vi "HEWH Stand Overide.vi"() -> ()   [LabVIEW 2016]
uses:
  Type Definitions/HEWH Channel Settings.ctl
  Type Definitions/HEWH Tank Indicator.ctl
  Custom Instrument Control/Intellifaucet/Type Definitions/INTELLIFAUCET Set Mode.ctl
  Type Definitions/HEWH Output Information.ctl
  Type Definitions/HEWH GEA2 Cluster.ctl
  Utility/LabVIEW GEA2 Toolkit v1.0.0.0/type defs/Data In.ctl
  Utility/LabVIEW GEA2 Toolkit v1.0.0.0/library/GEA2_Toolkit.lvlib
  Type Definitions/HEWH User Controls.ctl
  Type Definitions/HEWH Power Elements.ctl
  Utility/GEA2 Commands/HEWH/Type Definitions/GEA2 Commands WaterHeater GEA2 Data.ctl
  Type Definitions/HEWH Power Data.ctl
  Utility/Custom Pallet Controls/Custom Pallet String.ctl
  Utility/Custom Pallet Controls/Custom Pallet Quit.ctl
  Utility/Custom Pallet Controls/Custom Pallet DBL.ctl
  Custom Instrument Control/Intellifaucet/Type Definitions/INTELLIFAUCET Tested Flowrate Scenarios.ctl
  Type Definitions/HEWH Draw Pattern Setup.ctl
  Utility/Custom Pallet Controls/Custom Pallet Number.ctl
  Utility/Custom Pallet Controls/Custom Pallet Timer.ctl
  <vilib>/Analysis/NI_AALBase.lvlib
  Type Definitions/HEWH Valve Bank Positions.ctl
  Utility/GEA2 Commands/HEWH/Type Definitions/GEA2 Commands Service Error Codes.ctl
  Utility/GEA2 Commands/HEWH/Type Definitions/GEA2 Commands Status Query.ctl
  Utility/GEA2 Commands/HEWH/Type Definitions/GEA2 Commands Button Status.ctl
  Type Definitions/HEWH Termination Condition Cluster.ctl
  Drivers/Yokogawa WT300 Series/Yokogawa WT300 Series.lvlib
  Drivers/Yokogawa WT200 Series/Yokogawa WT200 Series.lvlib
  <vilib>/Utility/file.llb/Write To Spreadsheet File (DBL).vi
  Utility/Type Definitions/UTILITY Power Analyzer.ctl
  Utility/GEA2 Commands/HEWH/Type Definitions/GEA2 Commands HEWH Mode.ctl
  Utility/GEA2 Commands/HEWH/Type Definitions/GEA2 Commands.ctl
  C:/Technology Lab/NI-2010/Trunk/Utility/LabVIEW GEA2 Toolkit v1.0.0.0/Appliance.NET/GeaCommunication.dll
  Utility/LabVIEW GEA2 Toolkit v1.0.0.0/Appliance.NET/GeaCommunication.dll
  Utility/Type Definitions/UTILITY Notifier.ctl
  <vilib>/Utility/file.llb/Read From Spreadsheet File (string).vi
  Utility/Save File/File Setup.lvlib
  Utility/Save File/File Setup (Public)/Type Definition/Save File DOE Configuration State.ctl
  Utility/Save File/File Setup (Public)/Type Definition/Save File DOE LabView Program.ctl
  Custom Instrument Control/MW100/Type Definitions/Station ID Selector.ctl
  Utility/Save File/File Setup (Public)/Type Definition/Save File HEWH Heating Control Mode.ctl
  Type Definitions/PRAT Test.ctl
  Custom Instrument Control/MW100/Type Definitions/HEWH Solenoid Valve Status.ctl
  Type Definitions/HEWH Calc and Calibration.ctl
  Type Definitions/HEWH Start Conditions.ctl
  Support VIs/Draw Water Specific/Type Definitions/Terminate Draw Conditions.ctl
  Type Definitions/HEWH Draw Flag ENUM.ctl
  Support VIs/Draw Water Specific/Type Definitions/HEWH Special Condition Check.ctl
  Support VIs/Draw Water Specific/Type Definitions/Check Special Condtions.ctl
  <vilib>/Utility/file.llb/Write To Spreadsheet File (string).vi
  Type Definitions/HEWH Equipment References.ctl
  Utility/Custom Pallet Controls/Custom Pallet Chart.ctl
  Utility/Custom Pallet Controls/Custom Pallet Reverse.ctl
  Utility/Custom Pallet Controls/Custom Pallet Configuration.ctl
  Type Definitions/HEWH Program Names.ctl
  Type Definitions/HEWH PreDraw.ctl
  Utility/Save File/File Setup (Public)/Type Definition/Save File DOE Data Save Filepaths.ctl
  Utility/Save File/File Setup (Public)/Type Definition/Save File DOE File Path Control.ctl
  Utility/Type Definitions/UTILITY Power Inputs Control.ctl
  Drivers/IND560 Scale Monitor/Type Definitions/IND560 Configuration.ctl
  Type Definitions/HEWH Agilent Cluster.ctl
  Utility/Type Definitions/UTILITY TC Coefficients.ctl
  Washer DOE/Type Definitions/DOE Test Fixture Hardware.ctl
  Washer DOE/Configuration/GEA2.ctl
  Washer DOE/Type Definitions/DOE Capacity Measurments.ctl
  <vilib>/Platform/fileVersionInfo.llb/FileVersionInformation.ctl
  Utility/Save File/File Setup (Public)/Type Definition/Save File DISH Dishwasher Details.ctl
  Drivers/Omega FMA-1600A Series Gas Flow Meter/Type Definitions/FMA1600A COM Ports.ctl
  Washer DOE/Type Definitions/DOE Appliance Common.ctl
  Washer DOE/Type Definitions/DOE Dryer Standard.ctl
  Utility/Save File/File Setup (Public)/Type Definition/DPT IMC Data.ctl
panel:
  out "Error Out 2":errorcluster
  in  "24HR Error In":errorcluster
  in  "Skip Draw":bool
  in  "Skip Purge":bool
  out "DAQ Loop Complete":bool
  out "Core HEWH Data DAQ LOOP":T1={"Scan Rate Adjust"=0.0, "Draw Count"=0, "Test Patten Setup"={"Dispense Times"=[], "Total Gallons Schedule"=[], "Flow Rate Schedule "=[], "Incoming Water Temperature"=[], "PreDraw Pattern"=[], "24 Hour PreDraw"=enum."Zero Pre-Draws", "Pre-Draw Until?"=[], "Purge Until Cutout"=FALSE, "Heating Flag"=FALSE, "PRAT/RLT Sequence"=[]}, "Condition Cluster Output"={"Condition #1"=FALSE, "Condition #2"=FALSE, "Special Last Draw (HU Test)"=FALSE, "RTD Out Temperature <="=0.0, "Condition #3"=FALSE, "Mean Tank Temperature <="=0.0, "Condition #4"=FALSE, "Decrease Outlet Temperature \nBy (RTD Out)"=0.0, "Condition #5"=FALSE, "Condition #6"=FALSE, "Time (Seconds)"=0.0, "Condition #7"=FALSE, "Condition #8"=FALSE, "Draw Until Condition"={"UE"=FALSE, "LE"=FALSE, "COMP"=FALSE, "FANS"=FALSE}, "Condition #9"=FALSE}, "HEWH Specific DAQ"={"HEWH Data"={"HEWH Standard"={"Voltage (Volts)"=0.0, "Current (Amps)"=0.0, "Power (Watts)"=0.0, "WattHours (Wh)"=0.0, "TC Tree (AVG)"=0.0, "Flow Rate (GPM)"=0.0, "Gallons (Gal)"=0.0, "RTD Out (Deg F)"=0.0, "RTD In (Deg F)"=0.0, "RTD Amb (Deg F)"=0.0, "TC Down"=0.0, "UE Event Lead"=0, "LE Event Lead"=0, "TC Tree Array"=[]}, "PRAT"={"Power (Watts) A"=0.0, "Power (Watts) B"=0.0, "Power (Watts) C"=0.0, "Power (Watts) D"=0.0, "TC1"=0.0, "TC2"=0.0, "TC3"=0.0, "TC4"=0.0, "WattHours (Wh) A"=0.0, "WattHours (Wh) B"=0.0, "WattHours (Wh) C"=0.0, "WattHours (Wh) D"=0.0, "Ambient"=0.0, "Extra Temp"=0.0}, "Additional Power Data"={"Vthd"=0.0, "Frequency (Hz)"=0.0, "Apparent Power (VA)"=0.0, "Power Factor"=0.0, "Current Crest Factor"=0.0, "Voltage Crest Factor"=0.0, "Integration Time (sec)"=0.0}}, "Intellif Valve % Open"=0.0, "Power State"={"UE"=FALSE, "LE"=FALSE, "COMP"=FALSE, "FANS"=FALSE}, "Power Analyzer"=enum."", "Intellifaucet Configuration"=enum."DRK500,Station1"}, "Test Output Data"={"PreDraw Data Table"=[], "Data Table"=[], "MW100 TC Headers"=[]}, "Calc and Calibration"={"Mean SD Var Max Min Array"=[], "Draw Statistics (DBL)"=[], "Calibration Coefficients DBL"=[], "Start Gallons"=0.0, "Starting Temp Decline"=0.0, "K-Factor (Intellifaucet)"=0.0, "All Draw Stats"=[], "RTD Terminate Value"=0.0}, "Current Draw Time"=0.0, "LV Program"=enum."HEWH", "Station ID"=enum."A"} {"Test Patten Setup"."PRAT/RLT Sequence"."Time" format="%<%H:%M:%S>t"; "Test Patten Setup"."Incoming Water Temperature" format="%.2f"; "Test Patten Setup"."Flow Rate Schedule" format="%.2f"; "Test Patten Setup"."Total Gallons Schedule" format="%.2f"; "Test Patten Setup"."Dispense Times" format="%<%H:%M:%S>t"}
  out "Description 4":string
  out "Description":string="HEWH Stand Override"
  out "Station":string
  out "TC Tree Average":T19 format="%.2f"
  out "Elapsed Time Output":T20 format="%<%H:%M:%S>t"
  out "Continuous Data Collection Output":bool
  out "Cutout Draw":bool
  in  "Scan Rate (Seconds)":T19=3.0 format="%#.0f"
  in  "Tab Control 2":T21(tab)
  out "Data Table":string[][](array[string])
  in  "Inlet Valve A":enum8{"OPEN", "CLOSE"}(ring)=enum."CLOSE"
  in  "Drain Valve A":enum8{"OPEN", "CLOSE"}(ring)=enum."CLOSE"
  in  "Outlet Valve A":enum8{"CLOSE", "OPEN"}(ring)=enum."OPEN"
  in  "Stop Custom Draw":bool
  in  "Draw Until?":bool
  out "Multi-Draw":bool
  out "Remaining Draws":T22
  in  "Temperature":T19=58.0 format="%.2f"
  in  "Start Multi-Draw":bool
  in  "Draw Schedule":bool
  in  "GPM Target":T19=3.0 format="%.2f"
  in  "Gallon Target":T19=10.72 format="%.2f"
  out "Description 3":string="Custom Draw"
  out "Draw Time":T20 format="%<%H:%M:%S>t"
  in  "Dispense":bool
  out "Start Draw Routine":bool
  out "Start Draw Timer":bool
  out "Draw Count":T22
  out "Trigger With GEA2":bool
  in  "Super Water Heater":bool
  out "Sofware Version":T23
  in  "Software Version":bool
  in  "Setpoint":bool
  in  "Mode":T24
  in  "HEWH Setpoint":T22=135
  out "Start DAQ Write":bool
  out "Program Names Update":T25
  out "Flow Rate (GPM)":T19 format="%.2f"
  out "Tank Display":T26 {"TC6" format="%.2g"; "TIN" format="%.2g"; "TOUT" format="%.2g"; "TC5" format="%.2g"; "TC4" format="%.2g"; "TC3" format="%.2g"; "TC2" format="%.2g"; "TC1" format="%.2g"}
  out "Gallons":T19 format="%.2f"
  out "Voltage (Volts)":T19=240.0 format="%.3f"
  out "Current":T19=240.0 format="%.3f"
  out "Power (Watts)":T19=240.0 format="%.3f"
  out "Watt Hours (Wh)":T19=240.0 format="%.3f"
  out "Custom Draw\nDispensed Gallons (Gal)":T19 format="%.2f"
  out "POWER":T12
  in  "Shutdown Sequence":string
  in  "Settings":T27
  out "Intellifaucet Type":string
  out "Message":T23
  out "Shutdown DAQ":string="Stop Flow\nMacro: Exit"
  out "POWER DAQ LOOP":T12
  out "Out VLV UI":enum8{"CLOSE", "OPEN"}(ring)
  out "Drain VLV UI":enum8{"OPEN", "CLOSE"}(ring)
  out "In Valve UI":enum8{"OPEN", "CLOSE"}(ring)
  out "User Controls DAQ LOOP":T28={"Main Power Control"=FALSE, "Flow Totalizer Control"=TRUE, "Intellifaucet Temperature"=58.0, "Percent Flow"=100.0, "Safe Mode"=TRUE, "GEA2?"=FALSE, "Use Agilent?"=FALSE, "Valve Set A"=enum."Heating", "Valve Set B"=enum."Heating", "Valve Set C"=enum."Heating", "Valve Set D"=enum."Heating", "Valves"={"In VLV A"=enum."OPEN", "Drain VLV A"=enum."CLOSE", "Out VLV A"=enum."CLOSE", "In VLV B"=enum."CLOSE", "Drain VLV B"=enum."CLOSE", "Out VLV B"=enum."CLOSE", "In VLV C"=enum."OPEN", "Drain VLV C"=enum."CLOSE", "Out VLV C"=enum."CLOSE", "In VLV D"=enum."OPEN", "Drain VLV D"=enum."CLOSE", "Out VLV D"=enum."CLOSE"}} {"Percent Flow" scale=40.0..120.0; "Intellifaucet Temperature" scale=40.0..120.0}
  out "Shutdown":string="Stop Flow\nMacro: Exit"
  out "Elapsed Time":T20 format="%<%H:%M:%S>t"
  in  "Main":T30
  in  "Quit":T31
  in  "Tab Control 3":T32(tab)
  in  "Heat Up Panel":bool
  in  "First Hour Rating Panel":bool
  in  "24 Hour Rating Panel":bool
  in  "Stand Override Panel":bool
  in  "Program Names":T25
  in  "Tab Control 5":enum32{"Control", "Analysis"}(tab)
  in  "Flow Totalizer Control":bool
  in  "Reset Totalizer":bool
  in  "Pressurize Tank?":bool=TRUE
  out "Description 2":string="Intellifaucet Control"
  in  "IF Stop":bool
  in  "IF Start":bool
  in  "Valve % Open":dbl(slide)=100.0 scale=0.0..100.0
  in  "Temperature":dbl(slide)=58.0 scale=40.0..120.0
  in  "HEWH Power":bool
  in  "Write To File":bool
  out "Flow Meter 2":T33
  in  "Y-Axis":string(combo)
  in  "X-Axis":string(combo)
  out "XY Graph":cluster{dbl[], dbl[]}(graph)
  in  "Start 24 Hour Rating":bool
  out "24 Hr Test Complete":bool
  in  "Start First Hour Rating":bool
  in  "Start Heat Up Test":bool
  out "Save File Path":path
  in  "Tab Control 4":T34(tab)
  in  "Purge Time (Seconds)":T19=180.0 format="%.2f"
  in  "Last Draw TC Tree AVG Decline Amount (Degrees F)":T19=0.2 format="%.2f"
  in  "Decrease Outlet\nTemperature By (RTD Out)":T19=15.0 format="%.2f"
  out "RTD Max Min Array":dbl[][](array[numeric])
  in  "First Hour GPM Target":T19=3.0 format="%.2f"
  in  "First Hour Temperature":T19=58.0 format="%.2f"
  in  "Total Test Timer (1hr)":T19=3600.0 format="%.2f"
  in  "T2 Degree Diff for Purge":T19=8.0 format="%.2f"
  in  "Heat Up Temperature":T19=58.0 format="%.2f"
  in  "Heat Up GPM Target":T19=3.0 format="%.2f"
  in  "Step 1 Wait Time":T20=1800.0 format="%<%H:%M:%S>t"
  in  "Step 1A Gallon Target":T19=10.72 format="%.2f"
  in  "Step 2 Gallon Target":T19=10.72 format="%.2f"
  in  "Data File Directory":path=path "c:/data"
  in  "Tab Control":T35(tab)
  out "Write To File Change":bool
  out "Heat Up Step 4 Flag":bool
  out "Start UI Loop":bool
  out "Use Agilent?":bool
  out "Loop Time":dbl
  out "Newfi Time":dbl format="%.2f"
  out "Power Display Time":dbl format="%.2f"
  out "Start Time":dbl format="%.2f"
  in  "Scan Rate Adjust":T19=1000.0 format="%.2f"
  out "MW100 Data":string[][](array[string])
  in  "Standard Command":u8(ring)=13 items=["RQST_SOFTWARE_VERSION", "RQST_T2_RESISTANCE", "RQST_T3A_RESISTANCE", "RQST_T3B_RESISTANCE", "RQST_T4_RESISTANCE", "RQST_T5_RESISTANCE", "RQST_IDLB_RESISTANCE", "RQST_MODE_SELECT_RESISTANCE", "RQST_DATA_FROM_MEMORY", "RQST_DATA_FROM_DATA_FLASH", "RQST_SS_FAULT_COUNTS", "RQST_OTHER_FAULT_COUNTS", "CMD_CLEAR_FAULT_COUNTS", "RQST_HYPERTERM_OUTPUT_DATA", "CMD_RESET_FILTER_TIMES", "CMD_WRITE_SETPOINTS", "CMD_TURN_ON_OFF_DLB", "CMD_ENTER_EXIT_FCT_MODE", "CMD_SET_LEDS", "CMD_SET_EEV_DRIVE_LINES", "REQ_READ_KEY_STATUS", "RQST_READ_PERSONALITY", "CMD_ENTER_FACT_MODE", "CMD_RESET", "CMD_RESTORE_EEPROM_DEFAULTS", "CMD_SET_MODEL_NUMBER", "CMD_SET_SERIAL_NUMBER", "RQST_MODEL_NUMBER", "RQST_SERIAL_NUMBER", "CMD_TOGGLE_SERVICE_MODE", "CMD_TOGGLE_UE_SERV", "CMD_TOGGLE_LE_SERV", "CMD_REFRESH_SERVICE_TIMEOUTS", "RQST_DSM_OVERRIDE_STATUS", "RQST_STATUS_QUERY", "RQST_HEM_KWH_DATA", "RQST_SERVICE_ERROR_CODES", "RQST_OVERRIDE_STATUS", "CMD_UPDATE_DSM_LEVEL", "CMD_OVERRIDE_STATUS_CHANGED", "CMD_CLEAR_OVERRIDE_STATUS", "CMD_CLEAR_ENERGY_USAGE_CTRS", "CMD_DSM_OVERRIDES", "CMD_UPDATE_MODE", "CMD_SET_PID_P_DENOMINATOR", "CMD_SET_PID_I_DENOM_UNDER_THR", "CMD_SET_PID_I_DENOM_OVER_THR", "CMD_SET_START_POS_UNDER_THR", "CMD_SET_START_POS_OVER_THR", "CMD_SET_EEV_STOP_POSITION", "CMD_SET_AMBIENT_THRESH_1", "CMD_SET_AMBIENT_THRESH_2", "CMD_SET_AMBIENT_THRESH_3", "CMD_SET_PID_LOW_SH_TARGET", "CMD_SET_PID_MID_SH_TARGET", "RQST_PID_PARAMETERS", "CMD_COMP_OFF", "CMD_TOGGLE_FAN", "CMD_RQST_LED_STATUS", "CMD_UE_2_SECONDS", "CMD_LE_2_SECONDS", "CMD_COMP_ON", "CMD_HP_RUN_6MIN", "RQST_TEMP_RANGE", "RQST_VACATION_RANGE", "RQST_STD_ELEC_RANGE", "RQST_WATER_CAPACITY", "CMD_CANCEL_EEV_POSITION", "CMD_EEV_POSITION", "CMD_SET_CURRENTS", "RQST_SUPPORTED_MODES"]
  out "Header Info":string[](array[string])
  out "Special Last Draw":bool
  in  "Timer Step Size":dbl=50.0 format="%#_13g"
  out "Full Cutout":bool
  out "States":string[](array[string])
  in  "Debug":bool
  out "Error Out":errorcluster
  out "Data With Header":string[][](array[string])
  out "Start Value Signal Data Table":bool
  in  "Plot File":path=path "C:/work/PlotData.csv"
  in  "LV Program":T17=enum."HEWH"
  out "Water Heater GEA2 Data":T36 {"Hyperterminal Data"."CRC" format="%x"; "Hyperterminal Data"."Length" format="%x"; "Hyperterminal Data"."Command" format="%x"; "Hyperterminal Data"."Destination" format="%x"; "Hyperterminal Data"."Source" format="%x"}
  in  "Equipment VISA":T40={"MW100"="MW100", "AG34970"="A-34972A", "WT210"="WT210"}
  in  "24 Hour Rating":string="24 Hour Rating"
  in  "First Hour Rating":string="First Hour Rating"
  in  "Stand Override":string="HEWH Stand Override"
  in  "Heat Up":string="Heat Up"
  in  "Main 2":string="Main"
  in  "Settings 2":string="Settings"
  in  "Filepath":T41={"General Setup Paths"={"Calibration File Path"=path "", "DOE Capacity Path"=path "", "All Models Excel Sheet"=path "", "Network Model Location"=path "", "Data Folder Path"=path "", "DOE Backup"=path "", "Tool Base Path"=path "C:/GE/Washer DOE", "Configuration Path"=path "", "Appliance Prev Run Path"=path ""}, "Data File Paths"={"Data File Path"=path "", "Debug File Path"=path "", "Bus Log Path"=path "", "Current"=path "", "Summary"=path ""}, "New Summary Created"=FALSE, "Check Location Interval (Second)"=0}
  out "Final Data Cluster":T1={"Scan Rate Adjust"=0.0, "Draw Count"=0, "Test Patten Setup"={"Dispense Times"=[], "Total Gallons Schedule"=[], "Flow Rate Schedule "=[], "Incoming Water Temperature"=[], "PreDraw Pattern"=[], "24 Hour PreDraw"=enum."Zero Pre-Draws", "Pre-Draw Until?"=[], "Purge Until Cutout"=FALSE, "Heating Flag"=FALSE, "PRAT/RLT Sequence"=[]}, "Condition Cluster Output"={"Condition #1"=FALSE, "Condition #2"=FALSE, "Special Last Draw (HU Test)"=FALSE, "RTD Out Temperature <="=0.0, "Condition #3"=FALSE, "Mean Tank Temperature <="=0.0, "Condition #4"=FALSE, "Decrease Outlet Temperature \nBy (RTD Out)"=0.0, "Condition #5"=FALSE, "Condition #6"=FALSE, "Time (Seconds)"=0.0, "Condition #7"=FALSE, "Condition #8"=FALSE, "Draw Until Condition"={"UE"=FALSE, "LE"=FALSE, "COMP"=FALSE, "FANS"=FALSE}, "Condition #9"=FALSE}, "HEWH Specific DAQ"={"HEWH Data"={"HEWH Standard"={"Voltage (Volts)"=0.0, "Current (Amps)"=0.0, "Power (Watts)"=0.0, "WattHours (Wh)"=0.0, "TC Tree (AVG)"=0.0, "Flow Rate (GPM)"=0.0, "Gallons (Gal)"=0.0, "RTD Out (Deg F)"=0.0, "RTD In (Deg F)"=0.0, "RTD Amb (Deg F)"=0.0, "TC Down"=0.0, "UE Event Lead"=0, "LE Event Lead"=0, "TC Tree Array"=[]}, "PRAT"={"Power (Watts) A"=0.0, "Power (Watts) B"=0.0, "Power (Watts) C"=0.0, "Power (Watts) D"=0.0, "TC1"=0.0, "TC2"=0.0, "TC3"=0.0, "TC4"=0.0, "WattHours (Wh) A"=0.0, "WattHours (Wh) B"=0.0, "WattHours (Wh) C"=0.0, "WattHours (Wh) D"=0.0, "Ambient"=0.0, "Extra Temp"=0.0}, "Additional Power Data"={"Vthd"=0.0, "Frequency (Hz)"=0.0, "Apparent Power (VA)"=0.0, "Power Factor"=0.0, "Current Crest Factor"=0.0, "Voltage Crest Factor"=0.0, "Integration Time (sec)"=0.0}}, "Intellif Valve % Open"=0.0, "Power State"={"UE"=FALSE, "LE"=FALSE, "COMP"=FALSE, "FANS"=FALSE}, "Power Analyzer"=enum."", "Intellifaucet Configuration"=enum."DRK500,Station1"}, "Test Output Data"={"PreDraw Data Table"=[], "Data Table"=[], "MW100 TC Headers"=[]}, "Calc and Calibration"={"Mean SD Var Max Min Array"=[], "Draw Statistics (DBL)"=[], "Calibration Coefficients DBL"=[], "Start Gallons"=0.0, "Starting Temp Decline"=0.0, "K-Factor (Intellifaucet)"=0.0, "All Draw Stats"=[], "RTD Terminate Value"=0.0}, "Current Draw Time"=0.0, "LV Program"=enum."HEWH", "Station ID"=enum."A"} {"Test Patten Setup"."PRAT/RLT Sequence"."Time" format="%<%H:%M:%S>t"; "Test Patten Setup"."Incoming Water Temperature" format="%.2f"; "Test Patten Setup"."Flow Rate Schedule" format="%.2f"; "Test Patten Setup"."Total Gallons Schedule" format="%.2f"; "Test Patten Setup"."Dispense Times" format="%<%H:%M:%S>t"}
  in  "Washer Controls":T56={"Test Fixture Hardware"={"Power "={"Yokogawa"={"WT210"={"Sample Rate (1: 0.25s)"=1, "A Range (12: 20A)"=12, "V Range (6: 600V)"=4, "Power VISA Yokogawa WT210"="WT210"}, "WT500"={"Power VISA Yokogawa WT500"="WT500", "V Range (8: 1000V)"=0, "I Range (7: 40A)"=0, "Update Rate (3: 500ms)"=2}, "WT310_2"={"Sample Rate (1: 0.25s)"=1, "A Range (12: 20A)"=11, "V Range (6: 600V)"=4, "Power VISA Yokogawa WT310_2"="WT310_2"}, "WT310_3"={"Sample Rate (1: 0.25s)"=1, "A Range (12: 20A)"=11, "V Range (6: 600V)"=4, "Power VISA Yokogawa WT310_3"="WT310_3"}}, "Aplus"={"Aplus IP Address"="192.168.1.101", "Remote Port"=502, "Instrument"="APLUS", "Instr Driver Revision"="1.03.0053"}, "Power Limits"={"Crest Factor"={"Upper Limit"=1.49, "Lower Limit"=1.34}, "Harmonic Content"={"Uthd"=2.0}, "Voltage"={"% Error"=2.0}, "Stability"={"<1 Watt "={"Wattage"=1.0, "Slope (mW/H)"=10.0}, ">1 Watt"={"1%Power/Hour"=1.0}}}, "Nominal Voltage"=120, "Time Limit (s)"=10800.0, "Power Variation Limit (%)"=50.0, "Power Supply"={"Chroma 61605"="CHROMA", "Use Chroma?"=FALSE}}, "Weight Scale"={"Com Options"={"IND560Scale VISA"="LaurelMeter_Hot", "IP Address"="192.168.1.50", "Remote Port"=502, "Setra Scale VISA"="SETRA", "GSE 350"="GSE350"}, "Select Scale"=""}, "Flow Rates"={"Laurel Cold IP Address"="", "Laurel Hot IP Address"="", "Hot Water Laurel VISA"="34972A_3", "Cold Water Laurel VISA"="MW100", "Remote Port"=0, "Laurel Communication Type"="", "Meters To Collect (Hot Cold)"="", "HOT Laurel Reference"=refnum, "COLD Laurel Reference"=refnum}, "Analog Data"={"Agilent"={"Agilent 34972_1"="34972A_1", "Agilent 34972_2"="34972A_2", "Agilent 34972_3"="34972A_3", "Agilent 34972_4"="34972A_3", "Agilent 34972_5"="34972A_3", "Agilent 34972_6"="34972A_3", "Agilent Gain"=0.0, "TC Type (K,J,T)"="", "Instrument IDN?"="", "TC Channels-List"="", "Analog Channels-List"="", "Agilent Cluster Array"=[], "TC Channels-List 2"="", "Analog Channels-List 2"=""}, "Yokogawa"={"MW100"="MW100", "Intellifaucet"=FALSE}, "Select Analog"="", "TC Coefficients"={"TC Coefficients 1"=[], "TC Coefficients 2"=[], "TC Coefficients 3"=[], "TC Coefficients 4"=[], "TC Coefficients 5"=[], "TC Coefficients 6"=[], "TC Coefficients 7"=[]}, "NI Tasks (Dryer DOE)"=["TC Temps-Module 1", "TC Temps-Module 2", "TC Temps-Module 3", "TC Temps-Module 4", "TC Temps-Module 5", "Gas and Temp-Module 6", "AC_DC Events-Module 7"], "Laurel Analog"={"Laurel IP (Water Temp)"="", "Laurel IP (Pressure)"=""}}, "ITHX-Temp Humidity"={"IP Address 1"="", "Remote Port"=0, "IP Address 2"="", "IP Address 3"=""}, "Gas Meter COM Ports"={"Gas Meter 1"="COM3", "Gas Meter 2"="COM4", "Gas Meter 3"="COM5", "Gas Meter 4"="COM6", "Gas Meter 5"="COM7", "Gas Meter 6"="COM8"}, "Barometric Pressure"={"HEISE 901A"="HEISE", "Use Barometer?"=FALSE}}, "GEA2"={"Address"=35, "Source"=228, "Viper/Hawk"=0}, "DOE Capacity Measurments"={"Weight 1"=35.0, "Model Number 1"="", "Temp 1"=0.0, "Serial Number 1"="", "Lab Number 1"="", "Lab Number 2"="", "Serial Number 2"="", "Temp 2"=0.0, "Model Number 2"="", "Weight 2"=0.0, "Lab Number 3"="", "Serial Number 3"="", "Temp 3"=0.0, "Model Number 3"="", "Weight 3"=0.0, "Lab Number 4"="", "Serial Number 4"="", "Temp 4"=0.0, "Model Number 4"="", "Weight 4"=0.0, "Capacity Measurment Output String"=[]}, "Appliance Details"={"FileVersionInfo"={"FileVersion"="", "ProductName"="", "InternalName"="", "CompanyName"="", "LegalCopyright"="", "FileDescription"=""}, "Dishwasher Info"={"Open Cup Weight (gm):"=0.0, "Auto Cup Weight (gm):"=0.0, "Detergent-Dish:"="", "Inlet Temperature-Dish:"="", "Cycle Mode-Dish:"="", "Unit Control-Dish:"="", "Manufacturer-Dish:"=""}, "Washer Info"={"Hot Water Temperature (Fahrenheit):"="", "Cold Water Temperature (Fahrenheit):"="", "Capacity (cu.ft):"=0.0, "Initial Cloth Weight:"=0.0, "Cloth Lot:"=0, "Model Family:"="", "Program Name:"="", "Cycle Selection:"="", "Wash Temperature:"="", "Rinse Temperature:"="", "Load Size:"=""}, "File Name Output Array"=[], "Calibration Output Array"=[], "Appliance Common"={"Engineer:"="", "Model Number:"="", "Serial Number:"="", "Comments:"="", "Station ID:"="", "Technician:"="", "TR Number:"="", "Lab ID:"="", "Voltage:"="", "Water Pressure (PSI):"="", "Test Date:"="", "Computer Name:"="", "IP Address:"="", "Ambient RH:"="", "Frequency:"="", "Build:"="", "Filename:"="", "Test Type:"="", "Load Run #:"=0, "Ambient Temperature (F):"="", "File Path:"=path "", "Cycles Per Year"=60}, "Water Heater"={"Heating Mode:"=""}, "Dryer"={"Heat Setting:"="", "Washer Water Temperature (60 ± 5°F):"=60, "Water Hardness (PPM):"=17, "Dryness Setting:"="", "Dryer Type:"="", "Exhaust:"="", "Drying Cycle:"="", "Load Type:"="", "Nominal Load Weight"="", "Dryer Initial IMC Data"={"Measured IMC (lbs)"=7.0, "Actual Initial RMC (%)"=7.0, "RMC (Desired %)"=100.0, "Bone Dry Wt(lbs)"=7.0, "Tolerance(%)"=5.0, "Actual Final RMC (%)"=7.0, "CEF (lbf/kWh)"=0.0, "Minimum Weight (lbf)"=0.0, "Average Weight (lbf)"=0.0, "Maximum Weight (lbf)"=0.0, "Measured IMC In Range?"=FALSE, "Moisture Reduction Factor"=55.5, "Field Use Factor"=1.04, "Empty Dryer Cold Weigth"=0.0, "Energy Standard"=enum."D2-Automatic Dryer", "Weight Cloth (lbs)"=0.0, "Relative Moisture Content (%)"=0.0, "Relative Moisture Content - Avg (%)"=0.0}}}} {"Appliance Details"."Dryer"."Dryer Initial IMC Data"."Maximum Weight (lbf)" format="%03_6g"; "Appliance Details"."Dryer"."Dryer Initial IMC Data"."Average Weight (lbf)" format="%03_6g"; "Appliance Details"."Dryer"."Dryer Initial IMC Data"."Minimum Weight (lbf)" format="%03_6g"; "Appliance Details"."Dryer"."Dryer Initial IMC Data"."CEF (lbf/kWh)" format="%03_6g"; "Appliance Details"."Dryer"."Dryer Initial IMC Data"."Actual Final RMC (%)" format="%03_6g"; "Appliance Details"."Dryer"."Dryer Initial IMC Data"."Tolerance(%)" format="%0#_6g"; "Appliance Details"."Dryer"."Dryer Initial IMC Data"."Bone Dry Wt(lbs)" format="%03_6g"; "Appliance Details"."Dryer"."Dryer Initial IMC Data"."RMC (Desired %)" format="%0#_6g"; "Appliance Details"."Dryer"."Dryer Initial IMC Data"."Actual Initial RMC (%)" format="%03_6g"; "Appliance Details"."Dryer"."Dryer Initial IMC Data"."Measured IMC (lbs)" format="%0#_6g"; "GEA2"."Address" format="%x"; "GEA2"."Source" format="%x"; "GEA2"."Viper/Hawk" items=["Viper", "Hawk"]; "Test Fixture Hardware"."Power"."Yokogawa"."WT310_3"."V Range (6: 600V)" items=["Auto", "15V", "30V", "60V", "150V", "300V", "600V"]; "Test Fixture Hardware"."Power"."Yokogawa"."WT310_3"."A Range (12: 20A)" items=["Auto", "5mA", "10mA", "20mA", "50mA", "100mA", "200mA", "0.5A", "1A", "2A", "5A", "10A", "20A", "50mV", "100mV", "200mV", "2.5V", "5V", "10V"]; "Test Fixture Hardware"."Power"."Yokogawa"."WT310_3"."Sample Rate (1: 0.25s)" items=["0.1s", "0.25s", "0.5s", "1s", "2s", "5s"]; "Test Fixture Hardware"."Power"."Yokogawa"."WT310_2"."V Range (6: 600V)" items=["Auto", "15V", "30V", "60V", "150V", "300V", "600V"]; "Test Fixture Hardware"."Power"."Yokogawa"."WT310_2"."A Range (12: 20A)" items=["Auto", "5mA", "10mA", "20mA", "50mA", "100mA", "200mA", "0.5A", "1A", "2A", "5A", "10A", "20A", "50mV", "100mV", "200mV", "2.5V", "5V", "10V"]; "Test Fixture Hardware"."Power"."Yokogawa"."WT310_2"."Sample Rate (1: 0.25s)" items=["0.1s", "0.25s", "0.5s", "1s", "2s", "5s"]; "Test Fixture Hardware"."Power"."Yokogawa"."WT500"."Update Rate (3: 500ms)" items=["-", "100ms", "200ms", "500ms", "1s", "2s", "5s"]; "Test Fixture Hardware"."Power"."Yokogawa"."WT500"."I Range (7: 40A)" items=["AUTO", "500 mA", "1 A", "2 A", "5 A", "10 A", "20 A", "40 A", "S-AUTO", "50 mV", "100 mV", "200 mV", "500 mV", "1 V", "2 V", "5 V", "10 V", "250 mA", "500 mA", "1 A", "2.5 A", "5 A", "10 A", "20 A", "25 mV", "50 mV", "100 mV", "250 mV", "500 mV", "1 V", "2.5 V", "5 V"]; "Test Fixture Hardware"."Power"."Yokogawa"."WT500"."V Range (8: 1000V)" items=["AUTO", "15", "30", "60", "100", "150", "300", "600", "1000", "7.5", "15", "30", "50", "75", "150", "300", "500"]; "Test Fixture Hardware"."Power"."Yokogawa"."WT210"."V Range (6: 600V)" items=["Auto", "15V", "30V", "60V", "150V", "300V", "600V"]; "Test Fixture Hardware"."Power"."Yokogawa"."WT210"."A Range (12: 20A)" items=["Auto", "5mA", "10mA", "20mA", "50mA", "100mA", "200mA", "0.5A", "1A", "2A", "5A", "10A", "20A", "50mV", "100mV", "200mV", "2.5V", "5V", "10V"]; "Test Fixture Hardware"."Power"."Yokogawa"."WT210"."Sample Rate (1: 0.25s)" items=["0.1s", "0.25s", "0.5s", "1s", "2s", "5s"]}
  in  "Error In":errorcluster
  out "Flow Meter":dbl(graph)
  out "Total Dispensed Gallons":dbl(graph)
  out "Average TC Tree Temperature":dbl(graph)
  # "This is the software that I used in production. I have moved most of the draw sequence out....so it does not work.\n\nI recommned using the HEWH RLT PRAT software. It combined all packages in one software"
  # "Select Only One Condition"
  # "Just Draw Water!"
  # "Condition #1"
  # "Draw Until Any Heat Source"
  # "Condition #2"
  # "Start Dispense Pattern"
  # "Draw Until Specific Heat Source"
  # "Condition #3"
  # "Dispense PRAT Sequence"
  # "Not Working"
  # "Condition #4"
  # "Condition #5"
  # "Condition #6"
  # "Draw Pattern Setup (24 Hour)"
  # "Pre-Draw Items"
  # "Draw Start \nTime"
  # "Draw End\nTime"
  # "Max Temp\nDuring Draw"
  # "Min Temp\nDuring Draw"
  # "Mean Flow\nRate (GPM)"
  # "Flow Rate\nSTDev"
  # "Total\nGallons"
  # "Draw Count"
  # "Select Only One Condition"
  # "Just Draw Water!"
  # "Condition #1"
  # "Draw Until Any Heat Source"
  # "Condition #2"
  # "Start Dispense Pattern"
  # "Draw Until Specific Heat Source"
  # "Condition #3"
  # "Dispense PRAT Sequence"
  # "Not Working"
  # "Condition #4"
  # "Condition #5"
  # "Condition #6"
  # "Draw Pattern Setup (24 Hour)"
  # "Pre-Draw Items"
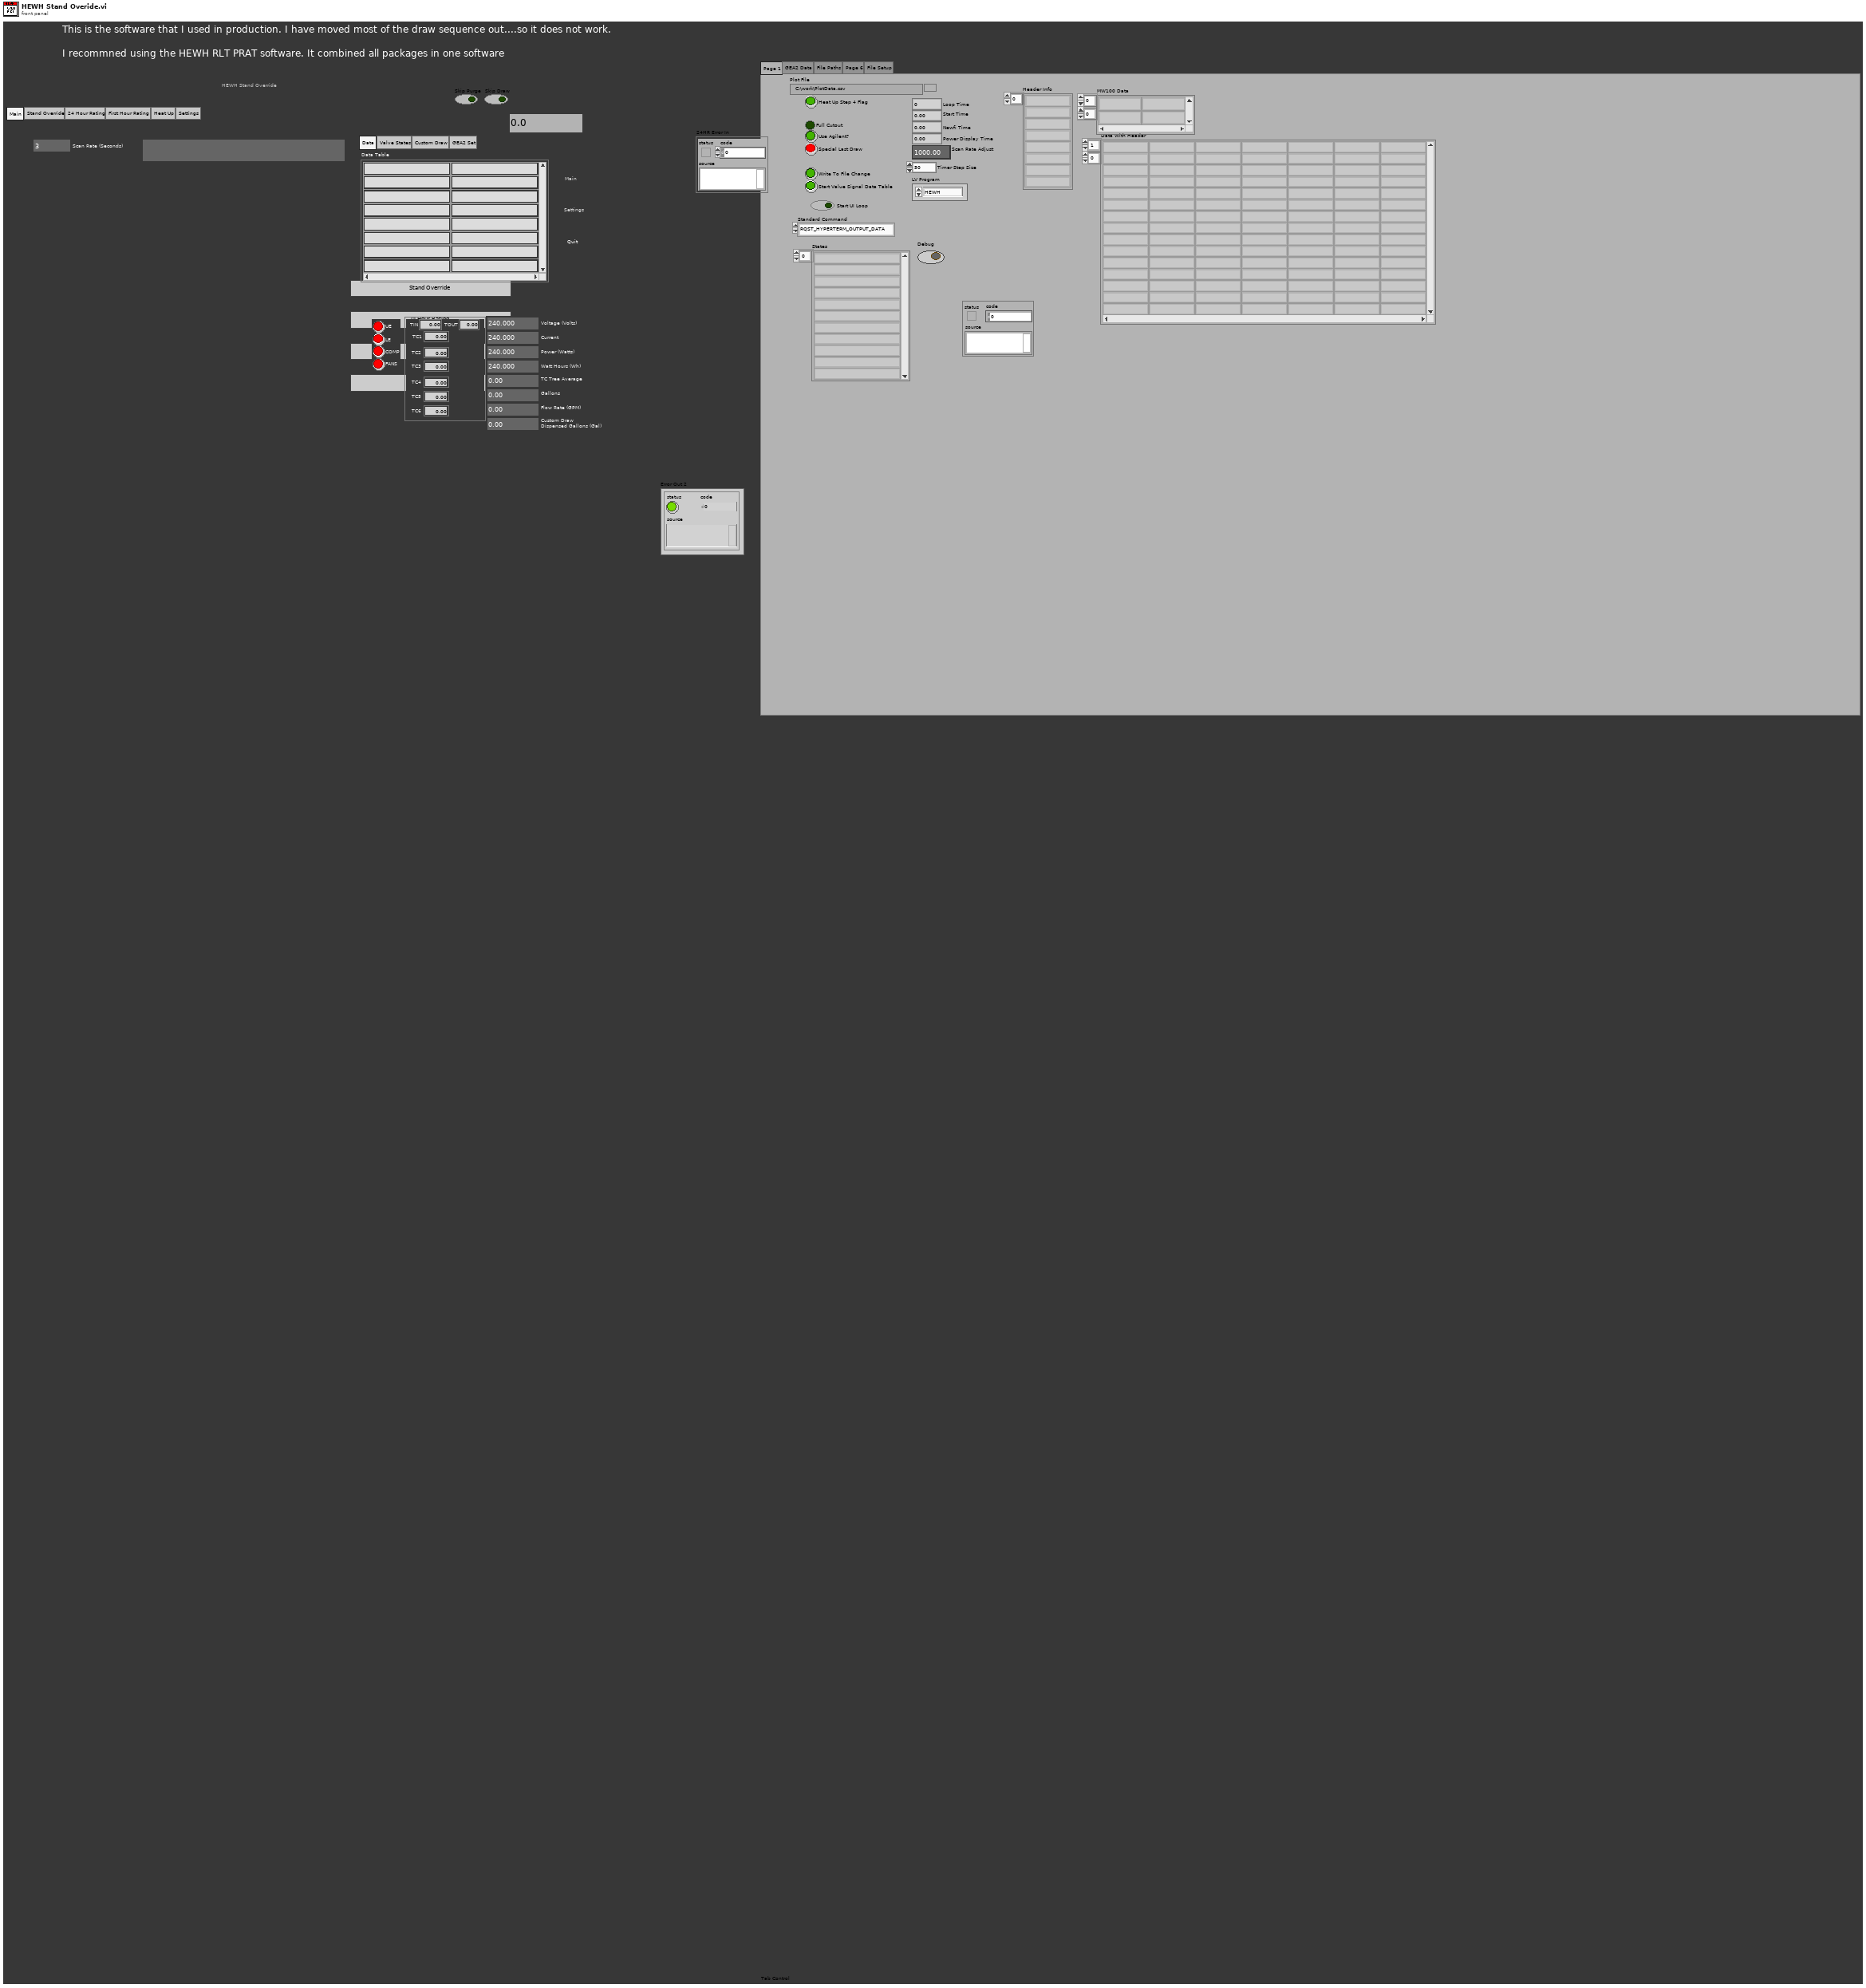
[diagram p1: front panel]
types:
  T1 = typedef "HEWH Output Information.ctl" = cluster{"Scan Rate Adjust":dbl, "Draw Count":i32, "Test Patten Setup":T2, "Condition Cluster Output":T11, "HEWH Specific DAQ":cluster{"HEWH Data":T13, "Intellif Valve % Open":dbl, "Power State":T12, "Power Analyzer":T14, "Intellifaucet Configuration":T15}, "Test Output Data":cluster{"PreDraw Data Table":string[][], "Data Table":string[][], "MW100 TC Headers":string[]}, "Calc and Calibration":T16, "Current Draw Time":dbl, "LV Program":T17, "Station ID":T18}
  T2 = typedef "HEWH Draw Pattern Setup.ctl" = cluster{"Dispense Times":dbl[], "Total Gallons Schedule":dbl[], "Flow Rate Schedule ":dbl[], "Incoming Water Temperature":dbl[], "PreDraw Pattern":dbl[][], "24 Hour PreDraw":T3, "Pre-Draw Until?":bool[], "Purge Until Cutout":bool, "Heating Flag":bool, "PRAT/RLT Sequence":T4[]}
  T3 = typedef "HEWH PreDraw.ctl" = enum16{"Zero Pre-Draws", "One Pre- Draws", "Two Pre-Draws", "Three Pre-Draws", ""}
  T4 = typedef "PRAT Test.ctl" = cluster{"Sequence #":dbl, "Cycles":i32, "Mode Setting":T5, "Flow Rate (GPM)":dbl, "Temperature (F)":dbl, "Reset Timer":bool, "Use Temp Decline Method":bool, "Terminate Condition":T6, "Condition Value #1":dbl, "UE":bool, "LE":bool, "Comp":bool, "Fan":bool, "Test End Time (Sec)":dbl, "Purge Until Cutout":bool, "Start Conditions":T7, "Condition Value #2":dbl, "Remove Power":bool, "Time":dbl, "Check Special Cond.":T8, "Condition#":T9, "Draw Flags":T10, "Data Processing Delay (FHD 15sec, UEF 5 Sec)":dbl, "Test Complete":bool}
  T5 = typedef "File Setup.lvlib/Save File HEWH Heating Control Mode.ctl" = string
  T6 = typedef "Terminate Draw Conditions.ctl" = enum16{"C1-Terminate Draw @ Gallon Mark", "C2-Special Last Draw (HU Test)", "C3-RTD Out <=", "C4-Mean Tank Temp <=", "C5-Decrease RTD Out (Deg F)", "C6-Time (Seconds)", "C7-Until Any Heat Source", "C8-Specific Heat Source", "C9-Do Nothing"}
  T7 = typedef "HEWH Start Conditions.ctl" = enum16{"Heat Source Cutout", "At Time (Seconds)", "Every X (Seconds)", "T2 >= X° Below Setpoint", "Seconds From Complete", "Wait for LE & Comp Cutout", "Wait for Comp Cutout", "Wait for LE Cutout", "Wait for UE Cutout"}
  T8 = typedef "Check Special Condtions.ctl" = enum16{"SC1-Do Nothing", "SC2-Check Heat Source (On-C2/Off-C1)", "SC3-Check Skip Condition", "SC4-Check Heat Source ON/Fail"}
  T9 = typedef "HEWH Special Condition Check.ctl" = enum16{"N/A", "C1", "C2", "Reset/Fail", "Skip Draw Sequence"}
  T10 = typedef "HEWH Draw Flag ENUM.ctl" = enum16{"N/A", "None(0)", "Sml(1)", "Med(2)", "SmlMed(3)", "Lrg(4)", "SmlLrg(5)", "MedLrg(6)", "SmlMedLrg(7)"}
  T11 = typedef "HEWH Termination Condition Cluster.ctl" = cluster{"Condition #1":bool, "Condition #2":bool, "Special Last Draw (HU Test)":bool, "RTD Out Temperature <=":dbl, "Condition #3":bool, "Mean Tank Temperature <=":dbl, "Condition #4":bool, "Decrease Outlet Temperature \nBy (RTD Out)":dbl, "Condition #5":bool, "Condition #6":bool, "Time (Seconds)":dbl, "Condition #7":bool, "Condition #8":bool, "Draw Until Condition":T12, "Condition #9":bool}
  T12 = typedef "HEWH Power Elements.ctl" = cluster{"UE":bool, "LE":bool, "COMP":bool, "FANS":bool}
  T13 = typedef "HEWH Power Data.ctl" = cluster{"HEWH Standard":cluster{"Voltage (Volts)":dbl, "Current (Amps)":dbl, "Power (Watts)":dbl, "WattHours (Wh)":dbl, "TC Tree (AVG)":dbl, "Flow Rate (GPM)":dbl, "Gallons (Gal)":dbl, "RTD Out (Deg F)":dbl, "RTD In (Deg F)":dbl, "RTD Amb (Deg F)":dbl, "TC Down":dbl, "UE Event Lead":i32, "LE Event Lead":i32, "TC Tree Array":dbl[]}, "PRAT":cluster{"Power (Watts) A":dbl, "Power (Watts) B":dbl, "Power (Watts) C":dbl, "Power (Watts) D":dbl, "TC1":dbl, "TC2":dbl, "TC3":dbl, "TC4":dbl, "WattHours (Wh) A":dbl, "WattHours (Wh) B":dbl, "WattHours (Wh) C":dbl, "WattHours (Wh) D":dbl, "Ambient":dbl, "Extra Temp":dbl}, "Additional Power Data":cluster{"Vthd":dbl, "Frequency (Hz)":dbl, "Apparent Power (VA)":dbl, "Power Factor":dbl, "Current Crest Factor":dbl, "Voltage Crest Factor":dbl, "Integration Time (sec)":dbl}}
  T14 = typedef "UTILITY Power Analyzer.ctl" = enum16{"", "APLUS", "WT210", "WT500", "WT300", "OSI", "Debug", "WT230", "WT300_1", "WT300_2"}
  T15 = typedef "INTELLIFAUCET Tested Flowrate Scenarios.ctl" = enum16{"DRK500,Station1", "DRK375,Lab", "SRK500,Station1,5GPM FR", "DRK375,STATION3,1/2\"HOSE", "DRK500,Station1,downspout", "DRK375,Station3,thruEcocute", "DRK375,Station3,purge", "Build2,2B,Purge", "Global, Purge", "Global, Tank", "DRK250"}
  T16 = typedef "HEWH Calc and Calibration.ctl" = cluster{"Mean SD Var Max Min Array":string[][], "Draw Statistics (DBL)":dbl[][], "Calibration Coefficients DBL":dbl[][], "Start Gallons":dbl, "Starting Temp Decline":dbl, "K-Factor (Intellifaucet)":dbl, "All Draw Stats":string[][], "RTD Terminate Value":dbl}
  T17 = typedef "File Setup.lvlib/Save File DOE LabView Program.ctl" = enum16{"No Name Found", "DOE Stand", "Dishwasher Kitchen", "Portable Stand", "HEWH", "Dryer", "Dryer WILT", "HCC", "PRAT", "HEWH RLT"}
  T18 = typedef "Station ID Selector.ctl" = enum16{"", "A", "B", "C", "D", "Global"}
  T19 = typedef "Custom Pallet DBL.ctl" = dbl
  T20 = typedef "Custom Pallet Timer.ctl" = dbl
  T21 = enum32{"Data", "Valve States", "Custom Draw", "GEA2 Set"}
  T22 = typedef "Custom Pallet Number.ctl" = u8
  T23 = typedef "Custom Pallet String.ctl" = string
  T24 = typedef "GEA2 Commands HEWH Mode.ctl" = enum16{"Hybrid", "Std Electric", "eHeat", "HighDemand", "Vacation"}
  T25 = typedef "HEWH Program Names.ctl" = cluster{"Stand Override":bool, "24 Hour Rating":bool, "First Hour Rating":bool, "Heat Up":bool, "Channel Tester":bool}
  T26 = typedef "HEWH Tank Indicator.ctl" = cluster{"TC1":dbl, "TC2":dbl, "TC3":dbl, "TC4":dbl, "TC5":dbl, "TIN":dbl, "TOUT":dbl, "TC6":dbl, "TC6-Color":u32, "TC5-Color":u32, "TC4-Color":u32, "TC3-Color":u32, "TC2-Color":u32, "TC1-Color":u32, "RTD-Out":u32, "RTD-In":u32}
  T27 = typedef "Custom Pallet Configuration.ctl" = bool
  T28 = typedef "HEWH User Controls.ctl" = cluster{"Main Power Control":bool, "Flow Totalizer Control":bool, "Intellifaucet Temperature":dbl, "Percent Flow":dbl, "Safe Mode":bool, "GEA2?":bool, "Use Agilent?":bool, "Valve Set A":enum16{"Heating", "Purge", "Resting", "Draw"}, "Valve Set B":enum16{"Heating", "Purge", "Resting", "Draw"}, "Valve Set C":enum16{"Heating", "Purge", "Resting", "Draw"}, "Valve Set D":enum16{"Heating", "Purge", "Resting", "Draw"}, "Valves":cluster{"In VLV A":T29, "Drain VLV A":T29, "Out VLV A":T29, "In VLV B":T29, "Drain VLV B":T29, "Out VLV B":T29, "In VLV C":T29, "Drain VLV C":T29, "Out VLV C":T29, "In VLV D":T29, "Drain VLV D":T29, "Out VLV D":T29}}
  T29 = typedef "HEWH Solenoid Valve Status.ctl" = enum8{"CLOSE", "OPEN"}
  T30 = typedef "Custom Pallet Reverse.ctl" = bool
  T31 = typedef "Custom Pallet Quit.ctl" = bool
  T32 = enum32{"Main", "Stand Override", "24 Hour Rating", "First Hour Rating", "Heat Up", "Settings"}
  T33 = typedef "Custom Pallet Chart.ctl" = dbl
  T34 = enum32{"Stand Override", "24 Hour Rating", "First Hour Rating", "Heat Up", "Channel Tester"}
  T35 = enum32{"Page 1", "GEA2 Data", "File Paths", "Page 6", "File Setup"}
  T36 = typedef "GEA2 Commands WaterHeater GEA2 Data.ctl" = cluster{"GEA2 Label Array":string[], "PID_PARAMETERS":string[][], "SUPPORTED_MODES":string[][], "Button Status":T37, "Status Query":T38, "Service Error Codes":T39, "HEM_KWH_DATA":string[][], "OTHER_FAULT_COUNTS":string[][], "GEA2 Raw Message":string, "Hyperterminal Data":cluster{"Source":u8, "Destination":u8, "Command":u8, "Length":u8, "CRC":u16, "UE - state (1/0 on off)":u8, "LE - state (1/0 on off)":u8, "Comp - state (1/0 on off)":u8, "Fan  - state (1/0 on off)":u8, "Setpoint Deg F":i32, "T2(TankSensor)":dbl, "T3A(EvapIn)":dbl, "T3B(EvapOut)":dbl, "T4(CompressorDischarge)":dbl, "T5(Ambient)":dbl, "Current":dbl, "Voltage (Volts)":u16, "EEV Position (0-480)":u16, "Reason for last heating cycle termination":u16, "Reason Data word 1":string, "Reason Data word 2":string, "Reason Data word 3":string, "Reason Data word 4":string, "SW Debug Data":string, "Flow Events (Bit Encoded)":u16, "Heating Control Mode":u16}, "Extra Data":cluster{"Water Capacity (Gallons)":u32, "Max Vacation Duration Days":u32, "Min Vacation Duration Days":u32, "Max Set Point (Deg F)":u32, "Min Set Point (Deg F)":u32, "T5 Resistance":u32, "T4 Resistance":u32, "T3B Resistance":u32, "T2 Resistance":u32, "STD_ELEC_RANGE":string, "SS_FAULT_COUNTS":string, "SERIAL_NUMBER":string, "READ_PERSONALITY":u8, "RQST_OVERRIDE_STATUS":string, "MODEL_SELECT_AD_VALUE":u32, "MODEL NUMBER":string, "IDLB_RESISTANCE":u32, "DSM Override Status":string, "RQST_DATA_FROM_Memory":string, "RQST_DATA_FROM_DATA_FLASH":string, "RQST_CURRENT_PID_SH_TARGET":u16, "Unit System Mode":string}}
  T37 = typedef "GEA2 Commands Button Status.ctl" = cluster{"Switch 1":bool, "Switch 2":bool, "Switch 3":bool, "Switch 4":bool, "Switch 5":bool, "Switch 6":bool, "Switch 7":bool, "Switch 8":bool, "Switch 9":bool, "Switch 10":bool, "Switch 11":bool, "Switch 12":bool, "Switch 13":bool, "Switch 14":bool, "Switch 15":bool, "Switch 16":bool}
  T38 = typedef "GEA2 Commands Status Query.ctl" = cluster{"Days Remaining (For Std Electric and Vacation)":u8, "Unit Status":string, "Current Tank Temp in Deg F":u8, "Current Setpoint in Deg F":u8, "Filter Status (% used)":u8, "Fallback Status (Fallback heating mode)":string, "Fallback Temp":u8, "\"Set Mode\" Selection":string}
  T39 = typedef "GEA2 Commands Service Error Codes.ctl" = cluster{"Reserved":bool, "Reserved 1":bool, "Reserved 2":bool, "Reserved 3":bool, "Reserved 4":bool, "Reserved 5":bool, "Reserved 6":bool, "Reserved 7":bool, "DataFlash Fail Status":bool, "Stuck Key Fail Status":bool, "Dry Tank Fail Status":bool, "Miswire Fail Status":bool, "Reserved 8":bool, "Reserved 9":bool, "Reserved 10":bool, "Reserved 11":bool, "UE Fail Status":bool, "LE Fail Status":bool, "Filter Fail Status":bool, "T3A Fail Status":bool, "T3B Fail Status":bool, "T4 Fail Status":bool, "T5 Fail Status":bool, "T2 Fail Status":bool, "SS Cond A Status":bool, "SS Cond B Status":bool, "SS Cond C Status":bool, "SS Cond D Status":bool, "SS Cond E Status":bool, "SS Cond F Status":bool, "SS Fan Status":bool, "CMP Fail Status":bool}
  T40 = typedef "HEWH Equipment References.ctl" = cluster{"MW100":refnum<visa-resource-name>, "AG34970":refnum<visa-resource-name>, "WT210":refnum<visa-resource-name>}
  T41 = typedef "File Setup.lvlib/Save File DOE File Path Control.ctl" = cluster{"General Setup Paths":cluster{"Calibration File Path":path, "DOE Capacity Path":path, "All Models Excel Sheet":path, "Network Model Location":path, "Data Folder Path":path, "DOE Backup":path, "Tool Base Path":path, "Configuration Path":path, "Appliance Prev Run Path":path}, "Data File Paths":T42, "New Summary Created":bool, "Check Location Interval (Second)":i32}
  T42 = typedef "File Setup.lvlib/Save File DOE Data Save Filepaths.ctl" = cluster{"Data File Path":path, "Debug File Path":path, "Bus Log Path":path, "Current":path, "Summary":path}
  T43 = typedef "DOE Test Fixture Hardware.ctl" = cluster{"Power ":T44, "Weight Scale":cluster{"Com Options":T45, "Select Scale":string}, "Flow Rates":cluster{"Laurel Cold IP Address":string, "Laurel Hot IP Address":string, "Hot Water Laurel VISA":refnum<visa-resource-name>, "Cold Water Laurel VISA":refnum<visa-resource-name>, "Remote Port":u16, "Laurel Communication Type":string, "Meters To Collect (Hot Cold)":string, "HOT Laurel Reference":refnum<k5>, "COLD Laurel Reference":refnum<k5>}, "Analog Data":cluster{"Agilent":cluster{"Agilent 34972_1":refnum<visa-resource-name>, "Agilent 34972_2":refnum<visa-resource-name>, "Agilent 34972_3":refnum<visa-resource-name>, "Agilent 34972_4":refnum<visa-resource-name>, "Agilent 34972_5":refnum<visa-resource-name>, "Agilent 34972_6":refnum<visa-resource-name>, "Agilent Gain":dbl, "TC Type (K,J,T)":string, "Instrument IDN?":string, "TC Channels-List":string, "Analog Channels-List":string, "Agilent Cluster Array":T46[], "TC Channels-List 2":string, "Analog Channels-List 2":string}, "Yokogawa":cluster{"MW100":refnum<visa-resource-name>, "Intellifaucet":bool}, "Select Analog":string, "TC Coefficients":T47, "NI Tasks (Dryer DOE)":refnum<k21>[], "Laurel Analog":cluster{"Laurel IP (Water Temp)":string, "Laurel IP (Pressure)":string}}, "ITHX-Temp Humidity":cluster{"IP Address 1":string, "Remote Port":u16, "IP Address 2":string, "IP Address 3":string}, "Gas Meter COM Ports":T48, "Barometric Pressure":cluster{"HEISE 901A":refnum<visa-resource-name>, "Use Barometer?":bool}}
  T44 = typedef "UTILITY Power Inputs Control.ctl" = cluster{"Yokogawa":cluster{"WT210":cluster{"Sample Rate (1: 0.25s)":i32, "A Range (12: 20A)":i32, "V Range (6: 600V)":i32, "Power VISA Yokogawa WT210":refnum<visa-resource-name>}, "WT500":cluster{"Power VISA Yokogawa WT500":refnum<visa-resource-name>, "V Range (8: 1000V)":i32, "I Range (7: 40A)":i32, "Update Rate (3: 500ms)":i32}, "WT310_2":cluster{"Sample Rate (1: 0.25s)":i32, "A Range (12: 20A)":i32, "V Range (6: 600V)":i32, "Power VISA Yokogawa WT310_2":refnum<visa-resource-name>}, "WT310_3":cluster{"Sample Rate (1: 0.25s)":i32, "A Range (12: 20A)":i32, "V Range (6: 600V)":i32, "Power VISA Yokogawa WT310_3":refnum<visa-resource-name>}}, "Aplus":cluster{"Aplus IP Address":string, "Remote Port":i32, "Instrument":string, "Instr Driver Revision":string}, "Power Limits":cluster{"Crest Factor":cluster{"Upper Limit":dbl, "Lower Limit":dbl}, "Harmonic Content":cluster{"Uthd":dbl}, "Voltage":cluster{"% Error":dbl}, "Stability":cluster{"<1 Watt ":cluster{"Wattage":dbl, "Slope (mW/H)":dbl}, ">1 Watt":cluster{"1%Power/Hour":dbl}}}, "Nominal Voltage":i32, "Time Limit (s)":dbl, "Power Variation Limit (%)":dbl, "Power Supply":cluster{"Chroma 61605":refnum<visa-resource-name>, "Use Chroma?":bool}}
  T45 = typedef "IND560 Configuration.ctl" = cluster{"IND560Scale VISA":refnum<visa-resource-name>, "IP Address":string, "Remote Port":u16, "Setra Scale VISA":refnum<visa-resource-name>, "GSE 350":refnum<visa-resource-name>}
  T46 = typedef "HEWH Agilent Cluster.ctl" = cluster{"Label":string, "Agilent Channel":string, "Panel ID":string, "Source":string, "Temperature":dbl}
  T47 = typedef "UTILITY TC Coefficients.ctl" = cluster{"TC Coefficients 1":dbl[], "TC Coefficients 2":dbl[], "TC Coefficients 3":dbl[], "TC Coefficients 4":dbl[], "TC Coefficients 5":dbl[], "TC Coefficients 6":dbl[], "TC Coefficients 7":dbl[]}
  T48 = typedef "FMA1600A COM Ports.ctl" = cluster{"Gas Meter 1":refnum<visa-resource-name>, "Gas Meter 2":refnum<visa-resource-name>, "Gas Meter 3":refnum<visa-resource-name>, "Gas Meter 4":refnum<visa-resource-name>, "Gas Meter 5":refnum<visa-resource-name>, "Gas Meter 6":refnum<visa-resource-name>}
  T49 = typedef "GEA2.ctl" = cluster{"Address":u8, "Source":u8, "Viper/Hawk":u8}
  T50 = typedef "DOE Capacity Measurments.ctl" = cluster{"Weight 1":dbl, "Model Number 1":string, "Temp 1":dbl, "Serial Number 1":string, "Lab Number 1":string, "Lab Number 2":string, "Serial Number 2":string, "Temp 2":dbl, "Model Number 2":string, "Weight 2":dbl, "Lab Number 3":string, "Serial Number 3":string, "Temp 3":dbl, "Model Number 3":string, "Weight 3":dbl, "Lab Number 4":string, "Serial Number 4":string, "Temp 4":dbl, "Model Number 4":string, "Weight 4":dbl, "Capacity Measurment Output String":string[][]}
  T51 = typedef "File Setup.lvlib/Save File DISH Dishwasher Details.ctl" = cluster{"FileVersionInfo":T52, "Dishwasher Info":cluster{"Open Cup Weight (gm):":dbl, "Auto Cup Weight (gm):":dbl, "Detergent-Dish:":string, "Inlet Temperature-Dish:":string, "Cycle Mode-Dish:":string, "Unit Control-Dish:":string, "Manufacturer-Dish:":string}, "Washer Info":cluster{"Hot Water Temperature (Fahrenheit):":string, "Cold Water Temperature (Fahrenheit):":string, "Capacity (cu.ft):":dbl, "Initial Cloth Weight:":dbl, "Cloth Lot:":i32, "Model Family:":string, "Program Name:":string, "Cycle Selection:":string, "Wash Temperature:":string, "Rinse Temperature:":string, "Load Size:":string}, "File Name Output Array":string[][], "Calibration Output Array":string[][], "Appliance Common":T53, "Water Heater":cluster{"Heating Mode:":string}, "Dryer":cluster{"Heat Setting:":T23, "Washer Water Temperature (60 ± 5°F):":u16, "Water Hardness (PPM):":u16, "Dryness Setting:":T23, "Dryer Type:":string, "Exhaust:":string, "Drying Cycle:":string, "Load Type:":string, "Nominal Load Weight":string, "Dryer Initial IMC Data":T54}}
  T52 = typedef "FileVersionInformation.ctl" = cluster{"FileVersion":string, "ProductName":string, "InternalName":string, "CompanyName":string, "LegalCopyright":string, "FileDescription":string}
  T53 = typedef "DOE Appliance Common.ctl" = cluster{"Engineer:":string, "Model Number:":string, "Serial Number:":string, "Comments:":string, "Station ID:":string, "Technician:":string, "TR Number:":string, "Lab ID:":string, "Voltage:":string, "Water Pressure (PSI):":string, "Test Date:":string, "Computer Name:":string, "IP Address:":string, "Ambient RH:":string, "Frequency:":string, "Build:":string, "Filename:":string, "Test Type:":string, "Load Run #:":i32, "Ambient Temperature (F):":string, "File Path:":path, "Cycles Per Year":u32}
  T54 = typedef "DPT IMC Data.ctl" = cluster{"Measured IMC (lbs)":dbl, "Actual Initial RMC (%)":dbl, "RMC (Desired %)":dbl, "Bone Dry Wt(lbs)":dbl, "Tolerance(%)":dbl, "Actual Final RMC (%)":dbl, "CEF (lbf/kWh)":dbl, "Minimum Weight (lbf)":dbl, "Average Weight (lbf)":dbl, "Maximum Weight (lbf)":dbl, "Measured IMC In Range?":bool, "Moisture Reduction Factor":dbl, "Field Use Factor":dbl, "Empty Dryer Cold Weigth":dbl, "Energy Standard":T55, "Weight Cloth (lbs)":dbl, "Relative Moisture Content (%)":dbl, "Relative Moisture Content - Avg (%)":dbl}
  T55 = typedef "DOE Dryer Standard.ctl" = enum16{"D2-Automatic Dryer", "D2-Timer Dryer", "D1-Automatic Dryer", "D1-Timer Dryer", "Other"}
  T56 = cluster{"Test Fixture Hardware":T43, "GEA2":T49, "DOE Capacity Measurments":T50, "Appliance Details":T51}
  T57 = typedef "UTILITY Notifier.ctl" = enum16{"Set", "Read", "Release Ref"}
  T58 = typedef "GEA2 Commands.ctl" = enum16{"CMD_CANCEL_EEV_POSITION", "CMD_CLEAR_ENERGY_USAGE_CTRS", "CMD_CLEAR_FAULT_COUNTS", "CMD_CLEAR_OVERRIDE_STATUS", "CMD_COMP_OFF", "CMD_COMP_ON", "CMD_DSM_OVERRIDES", "CMD_EEV_POSITION", "CMD_ENTER_EXIT_FCT_MODE", "CMD_ENTER_FACT_MODE", "CMD_HP_RUN_6MIN", "CMD_INITIATE_REMOTE_DSM_OVERRIDE", "CMD_LE_2_SECONDS", "CMD_REFRESH_SERVICE_TIMEOUTS", "CMD_RESET", "CMD_RESET_FILTER_TIMES", "CMD_RESTORE_EEPROM_DEFAULTS", "CMD_RQST_LED_STATUS", "CMD_SET_AMBIENT_THRESH_1", "CMD_SET_AMBIENT_THRESH_2", "CMD_SET_AMBIENT_THRESH_3", "CMD_SET_CURRENTS", "CMD_SET_EEV_DRIVE_LINES", "CMD_SET_EEV_STOP_POSITION", "CMD_SET_LEDS", "CMD_SET_MODEL_NUMBER", "CMD_SET_PID_I_DENOM_OVER_THR", "CMD_SET_PID_I_DENOM_UNDER_THR", "CMD_SET_PID_LOW_SH_TARGET", "CMD_SET_PID_MID_SH_TARGET", "CMD_SET_PID_P_DENOMINATOR", "CMD_SET_SERIAL_NUMBER", "CMD_SET_START_POS_OVER_THR", "CMD_SET_START_POS_UNDER_THR", "CMD_TOGGLE_FAN", "CMD_TOGGLE_LE_SERV", "CMD_TOGGLE_SERVICE_MODE", "CMD_TOGGLE_UE_SERV", "CMD_TURN_ON_OFF_DLB", "CMD_UE_2_SECONDS", "CMD_UPDATE_DSM_LEVEL", "CMD_UPDATE_MODE", "CMD_WRITE_SETPOINTS", "REQ_READ_KEY_STATUS", "REQ_SYSTEM_MODE", "RQST_CURRENT_PID_SH_TARGET", "RQST_DATA_FROM_DATA_FLASH", "RQST_DATA_FROM_MEMORY", "RQST_DSM_OVERRIDE_STATUS", "RQST_HEM_KWH_DATA", "RQST_HYPERTERM_OUTPUT_DATA", "RQST_IDLB_RESISTANCE", "RQST_MODEL_NUMBER", "RQST_MODEL_SELECT_AD_VALUE", "RQST_OTHER_FAULT_COUNTS", "RQST_OVERRIDE_STATUS", "RQST_PID_PARAMETERS", "RQST_READ_PERSONALITY", "RQST_SERIAL_NUMBER", "RQST_SERVICE_ERROR_CODES", "RQST_Software_Version", "RQST_SS_FAULT_COUNTS", "RQST_STATUS_QUERY", "RQST_STD_ELEC_RANGE", "RQST_SUPPORTED_MODES", "RQST_T2_RESISTANCE", "RQST_T3B_RESISTANCE", "RQST_T4_RESISTANCE", "RQST_T5_RESISTANCE", "RQST_TEMP_RANGE", "RQST_VACATION_RANGE", "RQST_WATER_CAPACITY"}
  T59 = typedef "GEA2_Toolkit.lvlib/Data In.ctl" = cluster{"Source":u8, "Destination":u8, "Command":u8, "Message":string}
  T60 = typedef "HEWH GEA2 Cluster.ctl" = cluster{"GEA2 Reference Out":refnum<k24>, "Data In":T59, "Water Heater GEA2 Data":T36, "GEA2 Commands and Requests":T58}
  T61 = cluster{"Equipment VISA":T40, "Save Data":string[][], "GEA2 Reference Out":T60, "User Controls DAQ LOOP":T28, "Core HEWH Data DAQ LOOP":T1, "POWER DAQ LOOP":T12}
  T62 = typedef "GEA2_Toolkit.lvlib/Data Out.ctl" = cluster{"Source":u8, "Destination":u8, "Command":u8, "Length":u8, "CRC":u16, "Message":string}
  T63 = typedef "ViperHawk Data.ctl" = cluster{"GEA Diagnostic Data - Washer":T64, "Software Version":T65, "Debug Search Parameters":T66, "Message Count":i32, "Number of Messages":i32, "Partial Message String":string, "Full Message to Save":string, "Board ID":string, "Board Index":i32, "Source Address":u8, "Destination Address":u8, "Data to send":u8[], "ReceivedData":u8[], "Debug/GEA Data":string[], "Command":u8, "GEA2 Reference Out":refnum<k24>, "GEA2 Event Registration":refnum<event-registration>, "Bus Data":string, "GEA Data":string[][], "Network Variable Location":i32, "Water Heater GEA2 Data":T36}
  T64 = typedef "ViperHawk Diagnostic Data.ctl" = cluster{"Speed (RPM)":u32, "Load Size":u32, "Temperature":u32, "Water Pressure":dbl, "Detergent":u32, "Fabric Softener":u32, "Tub Direction":string, "Detergent Valve":bool, "Fabric Softener Valve":bool, "Recirculating Pump":bool, "Drain Valve":bool, "Hot Valve":bool, "Cold Valve":bool, "Lid Closed Status":string, "Lid Lock Status":string, "Error Count":u32, "IGBT Temperature (Deg C)":u32, "Motor Speed":u32, "Latched OOB":u32, "Raw OOB":u32, "Plaster Status":u32, "Inverter Power (W)":u32, "Target Speed(BRPM)":u32, "Latched Agitate Motor Temp (Deg C)":u32, "Current Motor Temp (Deg C)":u32, "Profiler Status":string, "Current Inverter Action":string, "Error Codes":string, "Lid Locked":bool, "Lid Closed":bool, "9E Diagnostic Data":cluster{"Total Cycle Time (Min)":u32, "Total Cycle Count (Current)":u16, "Total Error Count":u16, "Machine Error History":u32, "Washer UI History":u32, "Inverter Error History":u32, "Cycle Storage Limit":u8, "Error Storage Limit":u8, "Cycle Pages Supported":u8, "Error Pages Supported":u8, "Inverter Reset Count":u16}, "9F Diagnostic Data":cluster{"Cycle Buffer Index":string, "Page Number":string, "Total Cycle Count":u32, "Delay Start Time":u32, "Stain Selected":string, "Selected Cycle":u32, "eWash":string, "Soil Level":string, "Temperature":string, "Overnight Ready":string, "Spin Setting":string, "Control Lock Status":string, "Stain Remover":string, "Steam Assist":string, "My Cycle":string, "PreWash":string, "Debug Log Enabled":string, "Rinse":string, "Signal Level":string, "PreSoak":string}}
  T65 = typedef "Save File.lvlib/Save File Software Version.ctl" = cluster{"Critical Major SW Version":string, "Critical Minor SW Version":string, "Major SW Version":string, "Minor SW Version":string, "Parametric Data Ver. Major":string, "Parametric Data Ver. Minor":string, "Diagnostics Data Ver. Major":string, "Diagnostics Data Ver. Minor":string, "Current Personality Setting":string}
  T66 = typedef "ViperHawk Search Control.ctl" = cluster{"Pause":string[], "Run":string[], "EOC":string[], "Error Codes":string[]}
  T67 = typedef "UTILITY Power Data.ctl" = cluster{"Current (A):Element 1":dbl, "Current (A):Element 2":dbl, "Power (W):Sigma":dbl, "Watt Hours (Wh):Sigma":dbl, "Voltage (V):Element 2":dbl, "Voltage (V):Element 1":dbl, "Current Crest Factor:Element 1":dbl, "Current Crest Factor:Element 2":dbl, "Voltage Harmonic (%):Element 1":dbl, "Voltage Harmonic (%):Element 2":dbl, "Voltage Crest Factor:Element 1":dbl, "Voltage Crest Factor:Element 2":dbl, "Time:Element 1":dbl, "Frequency (Hz):Element 1":dbl, "Apparent Power (VA):Element 1":dbl, "Apparent Power (VA):Element 2":dbl, "Power Factor:Element 1":dbl, "Power Factor:Element 2":dbl, "Max Watt Hours":dbl, "Voltage (V):Element 2 Avg":dbl, "Voltage (V):Element 1 Avg":dbl}
  T68 = enum32{"invalid app kind", "Development System", "Run Time System", "Student Edition", "Embedded LabVIEW", "Evaluation", "Custom"}
  T69 = typedef "HEWH Valve Bank Positions.ctl" = enum16{"Heating", "Purge", "Resting", "Draw"}
  T70 = enum32{"Invalid", "Standard", "Closed", "Hidden", "Minimized", "Maximized"}
  T71 = typedef "File Setup.lvlib/Save File DOE Configuration State.ctl" = enum16{"Open Front Panel", "Load Config"}
  T72 = typedef "INTELLIFAUCET Set Mode.ctl" = enum16{"Adjust Temp", "Adjust Flow", "Start Flow", "Stop Flow"}
  T73 = typedef "HEWH Output Information.ctl" = cluster{"Scan Rate Adjust":dbl, "Draw Count":i32, "Test Patten Setup":T74, "Condition Cluster Output":T11, "HEWH Specific DAQ":cluster{"HEWH Data":T13, "Intellif Valve % Open":dbl, "Power State":T12, "Power Analyzer":T14, "Intellifaucet Configuration":T15}, "Test Output Data":cluster{"PreDraw Data Table":string[][], "Data Table":string[][], "MW100 TC Headers":string[]}, "Calc and Calibration":T75, "Current Draw Time":dbl, "LV Program":T17, "Station ID":T18}
  T74 = typedef "HEWH Draw Pattern Setup.ctl" = cluster{"Total Gallons Schedule":dbl[], "PRAT/RLT Sequence":T4[], "Current Sequence Index":i32}
  T75 = typedef "HEWH Calc and Calibration.ctl" = cluster{"RTD Max Min Array":dbl[][], "Draw Statistics":dbl[][], "Calibration Coefficients DBL":dbl[][], "Min RTD Temp\nDuring Draw":dbl, "Start Gallons":dbl, "Starting Temp Decline A":dbl, "Max RTD Temp\nDuring Draw":dbl, "Draw Start Time":dbl, "Delay Start Time":dbl, "Current Purge Start Time":dbl, "K-Factor (Intellifaucet)":dbl, "Starting Temp Decline B":dbl, "Starting Temp Decline C":dbl, "Starting Temp Decline D":dbl}
  T76 = cluster{"Core":cluster{"Current VI Reference":refnum<vi>, "Close Panel on Exit?":bool}, "Data File Directory":path, "Core HEWH Data":T73, "Equipment VISA":T40, "User Controls":T28, "Save Data":string[][], "Filepath":T41, "LV Program":T17, "Washer Controls":cluster{"Test Fixture Hardware":T43, "GEA2":T49, "DOE Capacity Measurments":T50, "Appliance Details":T51}}
  T77 = cluster{"Current VI Reference":refnum<vi>, "Close Panel on Exit?":bool}
  T78 = typedef "DOE Main Control.ctl" = cluster{"Test Fixture Hardware":T43, "GEA2":T49, "DOE Capacity Measurments":T50, "Initialize.Washer In":T79}
  T79 = typedef "Save File.lvlib/Save File Washer.ctl" = cluster{"Appliance Details":T51, "Display Data (RLT)":T80}
  T80 = typedef "Save File Appliance Display.ctl" = cluster{"Status Color":u32, "Serial Number Display":string, "Cycle Count Display":i32, "Station Label Display":string, "Current Run Start Time Display":dbl, "Board ID Display":string, "RPM Display":u32, "Current Display":dbl, "Current Path Display":path, "Saving Display":bool, "Unit Type Display":T81, "Total Time On Display":dbl, "UI Button":bool}
  T81 = typedef "Save File.lvlib/Save File Unit Type.ctl" = enum32{"", "Viper", "Hawk", "2015"}
  T82 = typedef "File Setup.lvlib/Save File DOE File Path Control.ctl" = cluster{"General Setup Paths":cluster{"Calibration File Path":path, "DOE Capacity Path":path, "Data Folder Path":path, "RLT Backup Data Path":path, "Tool Base Path":path, "General Startup Config Path":path, "File Save Previous Run Path":path, "File Save Configuration Data Path":path}, "Data File Paths":T42, "New Summary Created":bool, "Check Location Interval (Second)":i32}
  T83 = typedef "HEWH Output Information.ctl" = cluster{"Scan Rate Adjust":dbl, "Draw Count":i32, "Test Patten Setup":T74, "HEWH Specific DAQ":T84, "Test Output Data":cluster{"PreDraw Data Table":string[][], "Data Table":string[][], "MW100 TC Headers":string[]}, "Calc and Calibration":T16, "Current Draw Time":dbl, "LV Program":T17, "Station ID":T18, "Current Cond":T9, "Test Complete":bool}
  T84 = typedef "HEWH Specific DAQ.ctl" = cluster{"HEWH Data":T13, "Intellif Valve % Open":dbl, "Power State":T12, "Power Analyzer":T14}
  T85 = typedef "HEWH Channel Settings.ctl" = u32
  T86 = cluster{"User Controls DAQ LOOP":T28, "Program Names":T25}
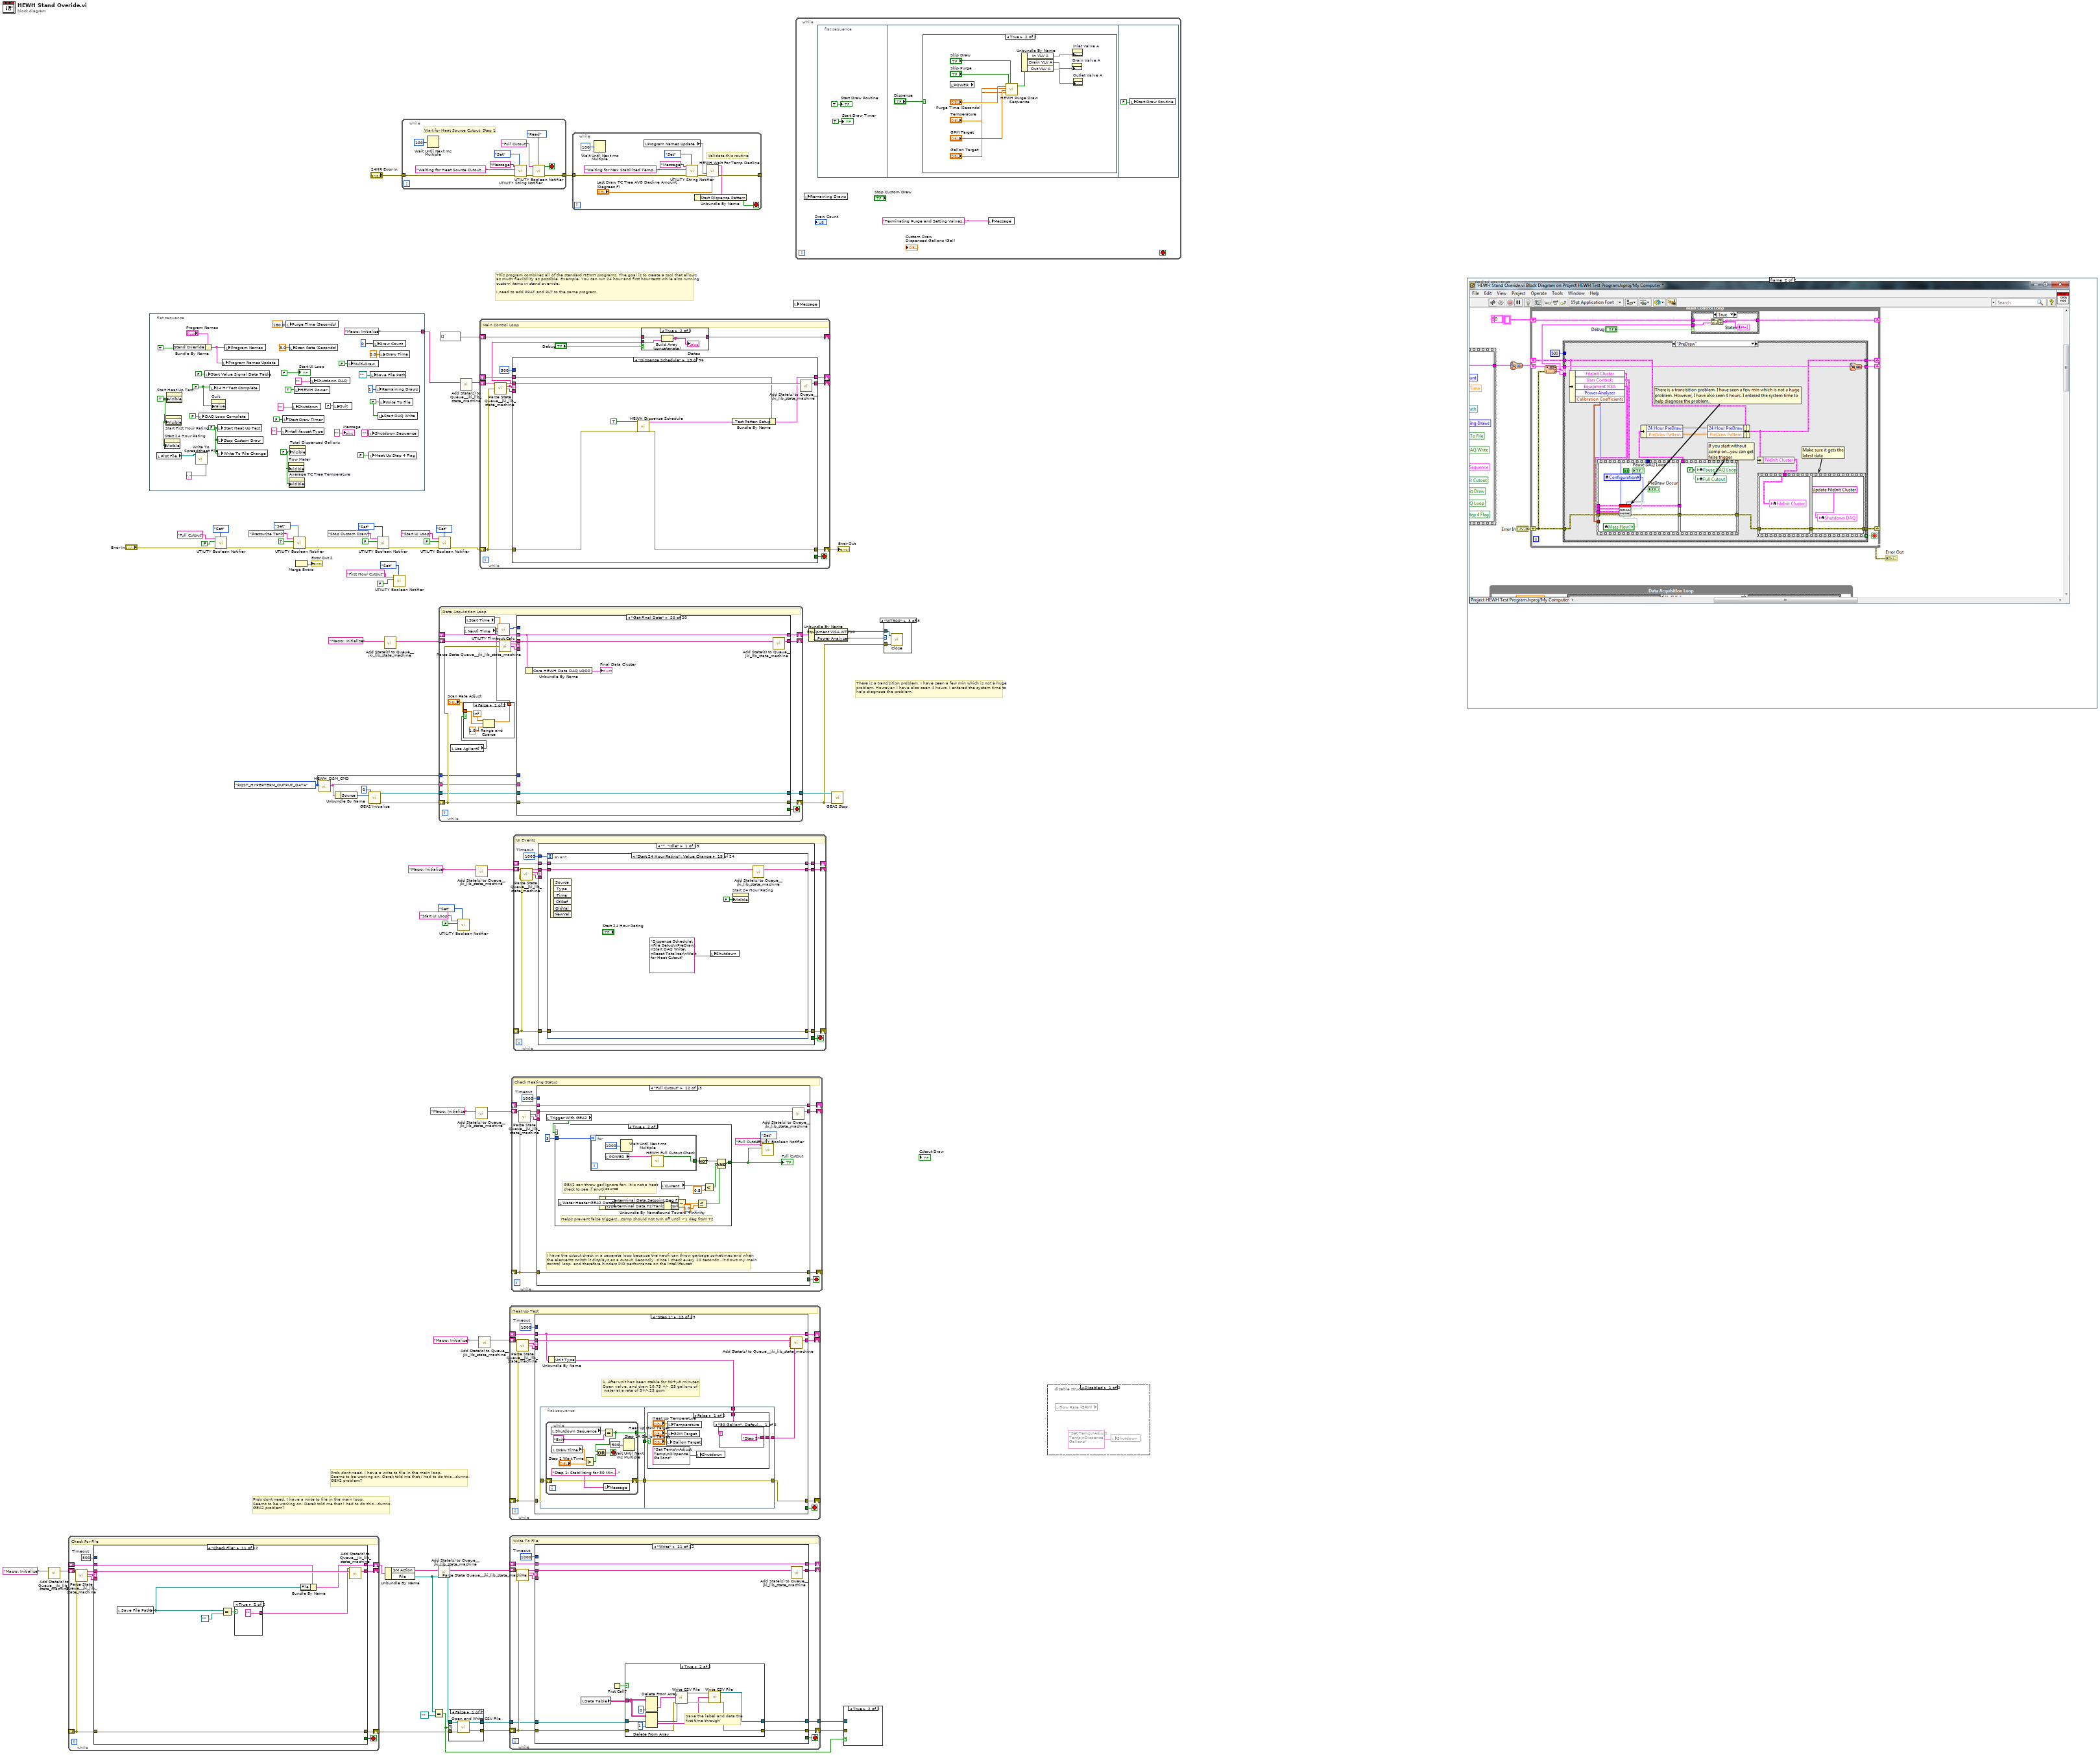
[diagram p0: block diagram]
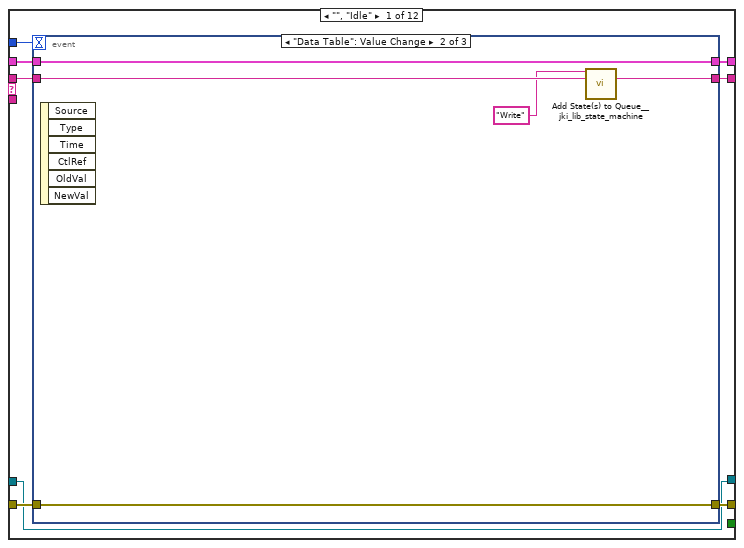
[diagram p5: hidden frame]
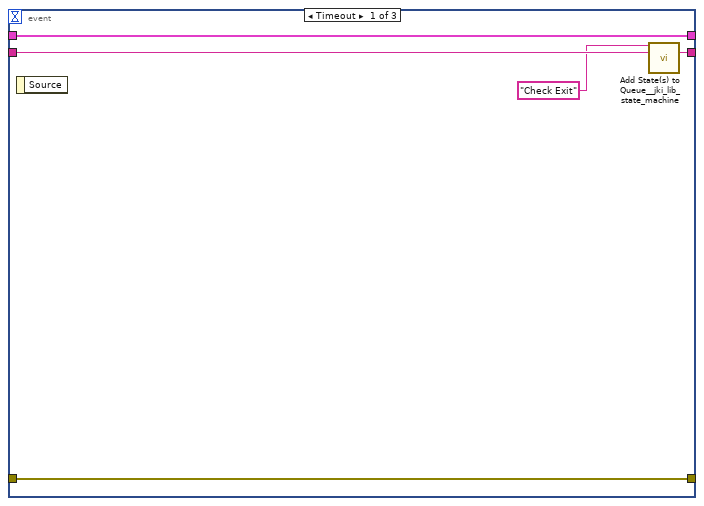
[diagram p6: hidden frame]
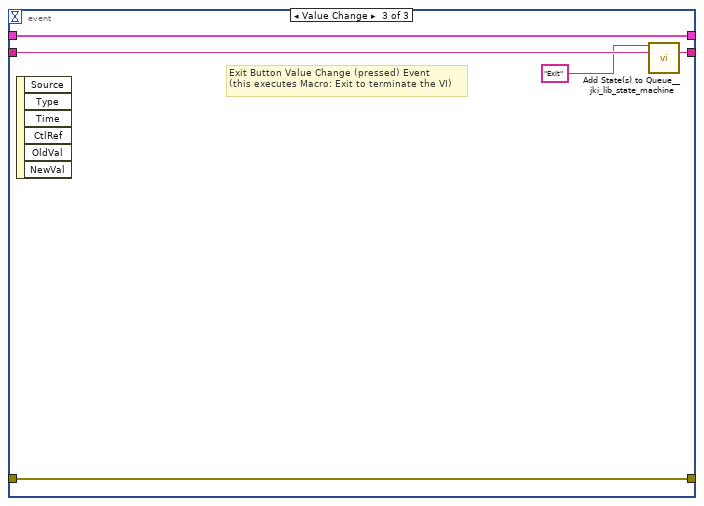
[diagram p7: hidden frame]
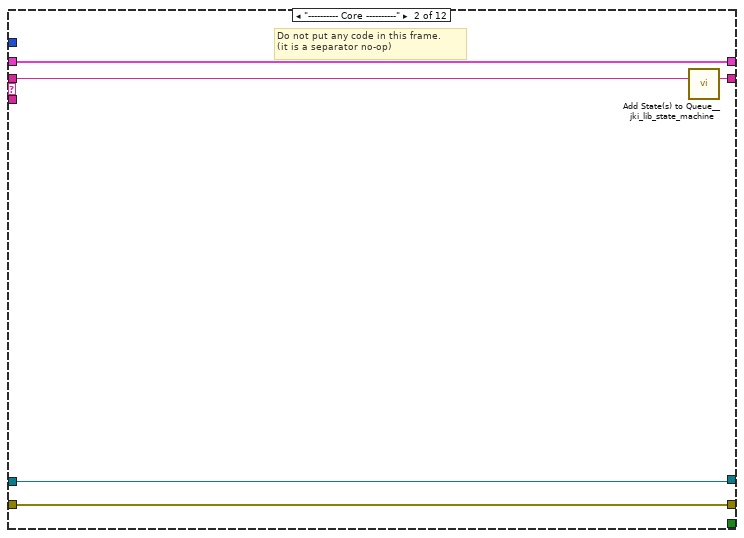
[diagram p8: hidden frame]
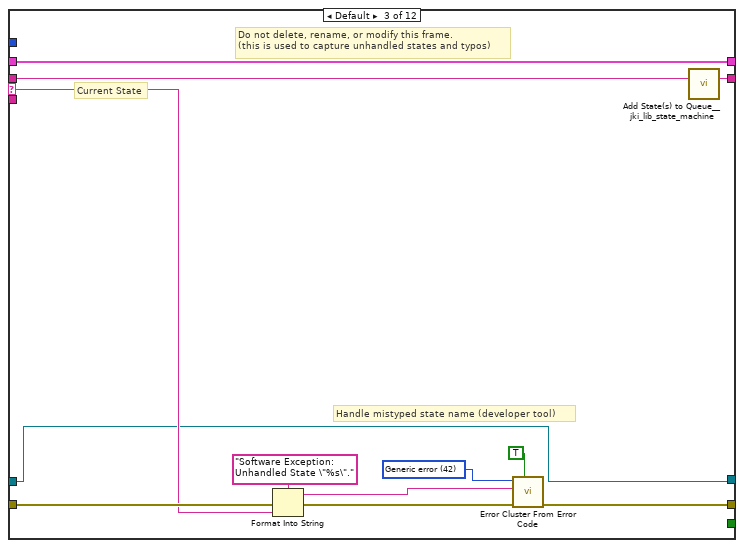
[diagram p9: hidden frame]
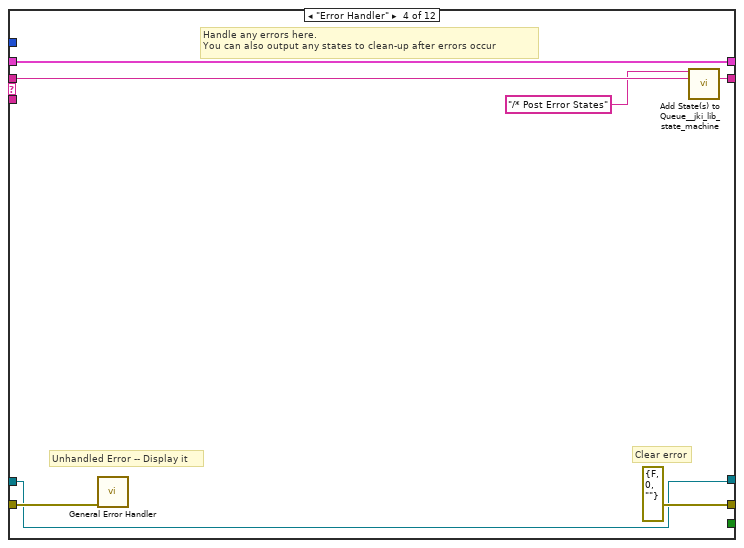
[diagram p10: hidden frame]
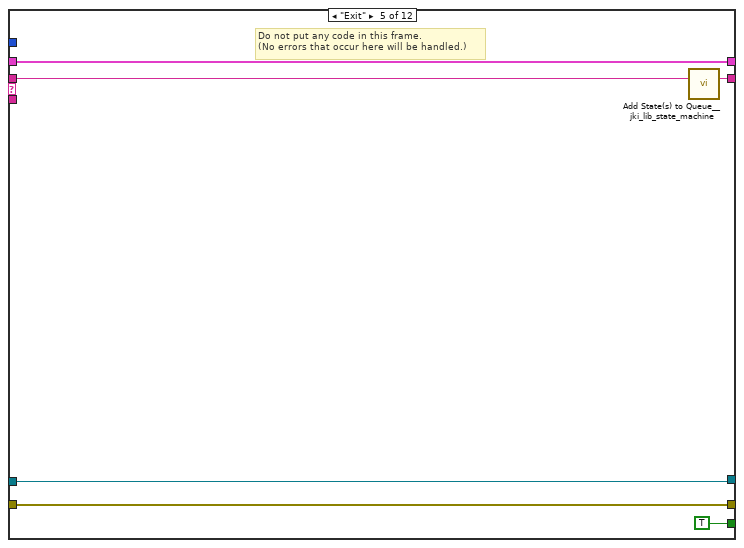
[diagram p11: hidden frame]
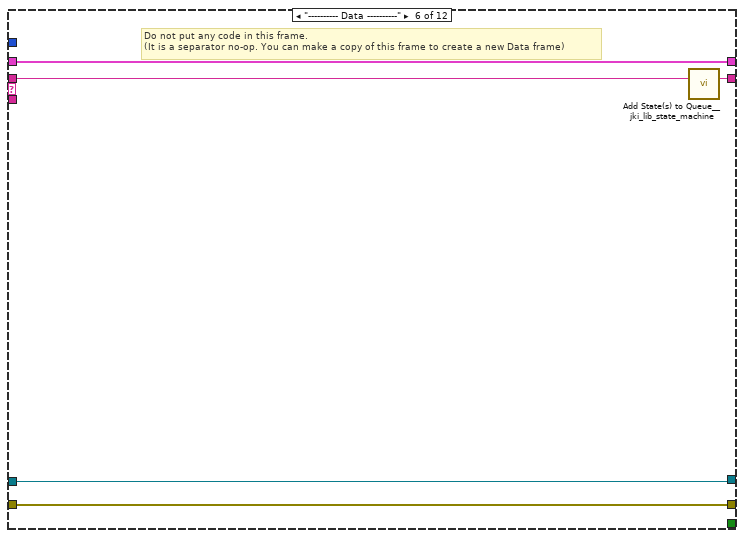
[diagram p12: hidden frame]
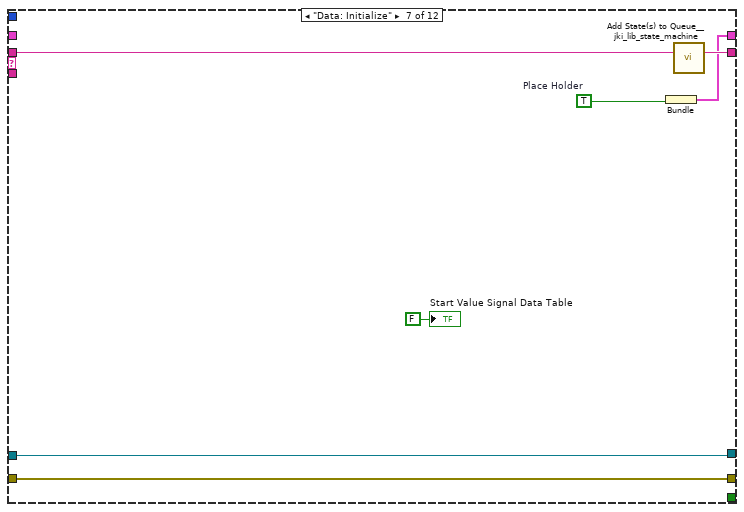
[diagram p13: hidden frame]
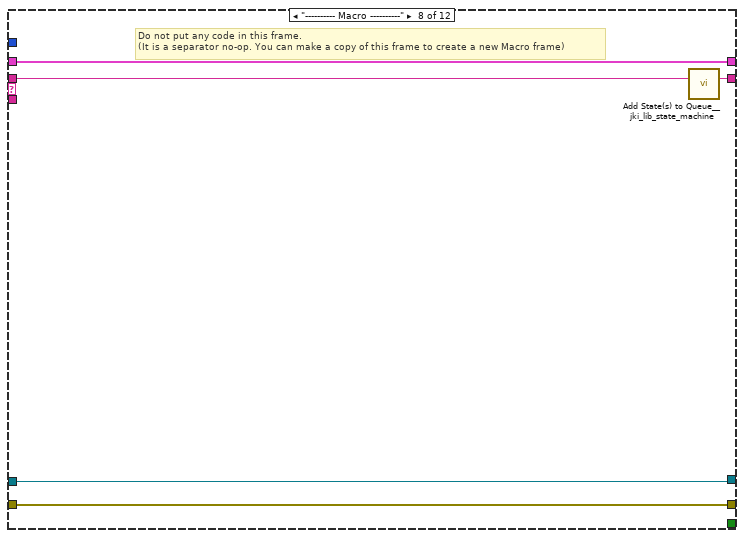
[diagram p14: hidden frame]
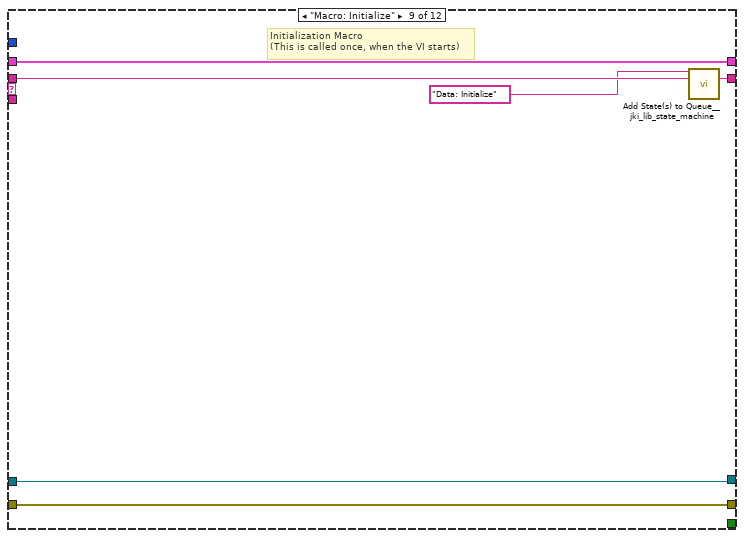
[diagram p15: hidden frame]
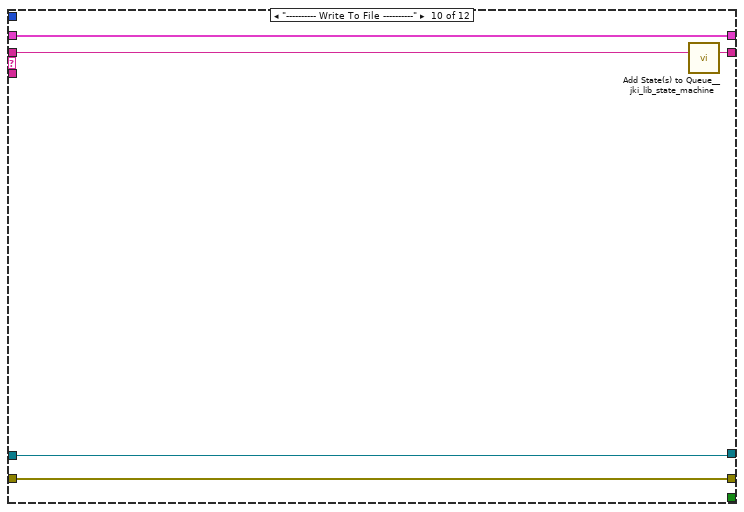
[diagram p16: hidden frame]
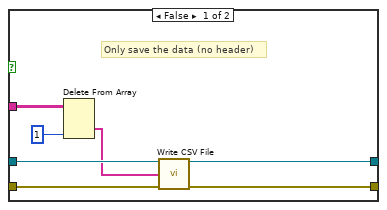
[diagram p17: hidden frame]
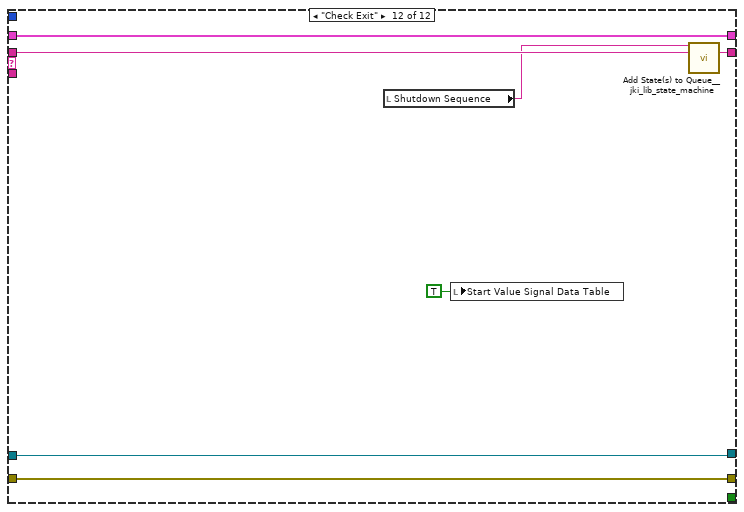
[diagram p18: hidden frame]
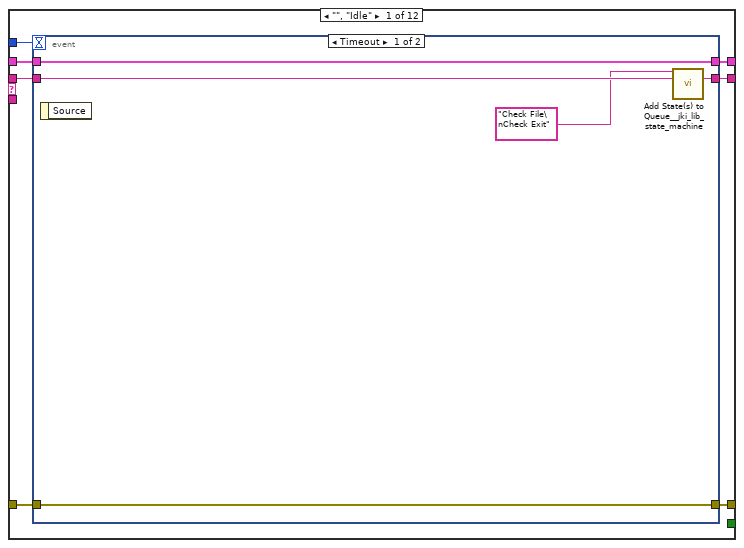
[diagram p19: hidden frame]
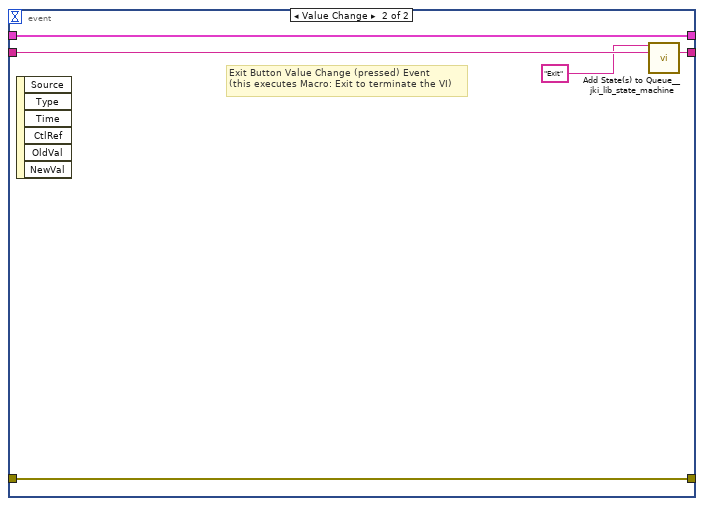
[diagram p20: hidden frame]
diagram:
  w52 = GEA2_Commands."RQST_HYPERTERM_OUTPUT_DATA" ("GEA2 Commands and Requests")
  # "There is a transisition problem. I have seen a few min which is not a huge \nproblem. However, I have also seen 4 hours. I entered the system time to\nhelp diagnose the problem."
  # "This program combines all of the standard HEWH programs. The goal is to create a tool that allows\nas much flexibility as possible. Example. You can run 24 hour and first hour tests while also running \ncustom items in stand override.\n\nI need to add PRAT and RLT to the same program."
  # "Prob dont need. I have a write to file in the main loop.\nSeems to be working on. Derek told me that i had to do this...dunno.\nGEA2 problem?"
  # "Prob dont need. I have a write to file in the main loop.\nSeems to be working on. Derek told me that i had to do this...dunno.\nGEA2 problem?"
  n1 = call <vilib>:"Add State(s) to Queue__jki_lib_state_machine.vi"("State(s) in (\"\")"="Macro: Initialize") -> ("States Out"=w27:string)  [unwired: 14 in]
  n2 = while "Write to File" {
    shift-right: [w66] -> w31
    shift-left: _ -> [w65]
    shift-right: [w69] -> w32
    shift-left: _ -> [w63]
    shift-right: [w68] -> _
    shift-left: w27 -> [w70]
    stop <- w67 stop-if-true
    w64 = 500  # Timeout
    # "Check For File"
    n3 = call <vilib>:"Parse State Queue__jki_lib_state_machine.vi"("State Queue"=w70, "Error In (no error)"=w63) -> ("Remaining States"=w72:string, "Current State"=w73:string, "Arguments"=w71:string)  [unwired: 11 in]
    n4 = case shown="\"Check File\"" w73 {
      selector: w73 -> [_ _ w95 _ _ _ _ _ _ _ _ _]
      tunnel: w72 -> [w80 w94 w99 w111 w121 w127 w133 w144 w149 w153 w162 w169]
      tunnel: w71 -> [_ _ _ _ _ _ _ _ _ _ _ _]
      tunnel: w65 -> [w78 w91 w97 w108 w116 w124 _ w141 w146 w150 w159 w167]
      tunnel: [w77 w92 w101 errorcluster {"status"=FALSE, "code"=0, "source"=""} ("error out") w119 w125 w130 w142 w147 w151 w160 w166] -> w69
      tunnel: w63 -> [w76 w92 w100 w107 w119 w125 w130 w142 w147 w151 w160 w166]
      tunnel: [w79 w93 w98 w110 w120 w126 w132 w143 w148 w152 w161 w168] -> w68
      tunnel: [_ _ _ _ TRUE _ _ _ _ _ _ _] -> w67
      tunnel: [w75 w91 w97 w108 w117 w124 w131 w141 w146 w150 w158 w167] -> w66
      tunnel: w64 -> [w74 _ _ _ _ _ _ _ _ _ _ _]
      frame "", "Idle" {
        n5 = event shown="[0] Timeout" {
          selector: _ -> [_ _]
          dyn-events: _ -> [_ _]
          timeout: w74 -> [_ _]
          tunnel: w80 -> [w85 w90]
          tunnel: [w84 w89] -> w79
          tunnel: w78 -> [w83 w87]
          tunnel: [w82 w88] -> w77
          tunnel: w76 -> [w82 w88]
          tunnel: [w83 w87] -> w75
          event Timeout {
            n6 = event-data() -> ()  [unwired: 1 in, 1 out]
            n7 = call <vilib>:"Add State(s) to Queue__jki_lib_state_machine.vi"("State(s) in Front (\"\")"="Check File\nCheck Exit" ("State(s) in Front (\"\")"), "State(s) in (\"\")"=w85) -> ("States Out"=w84:string)  [unwired: 13 in]
          }
          event Value Change {
            # "Exit Button Value Change (pressed) Event\n(this executes Macro: Exit to terminate the VI)"
            n8 = event-data() -> ()  [unwired: 1 in, 6 out]
            n9 = call <vilib>:"Add State(s) to Queue__jki_lib_state_machine.vi"("State(s) in Front (\"\")"="Exit", "State(s) in (\"\")"=w90) -> ("States Out"=w89:string)  [unwired: 13 in]
          }
        }
      }
      frame "---------- Core ----------" {
        # "Do not put any code in this frame.\n(it is a separator no-op)"
        n10 = call <vilib>:"Add State(s) to Queue__jki_lib_state_machine.vi"("State(s) in (\"\")"=w94) -> ("States Out"=w93:string)  [unwired: 14 in]
      }
      frame Default {
        w104 = 42 items=["No error", "Argument error", "Memory is full", "Out of zone", "End of file", "File already open", "Generic file I/O error", "File not found", "File permission error", "Disk is full", "Duplicate path", "Too many files open", "System feature not enabled", "Resource file not found", "Cannot add resource", "Resource not found", "Image not found", "Image memory error", "Pen does not exist", "Config type invalid", "Config token not found", "Config parse error", "Config memory error", "Bad external code format", "Bad external code offset", "External code not present", "Null window", "Destroy window error", "Null menu", "Print aborted", "Bad print record", "Print driver error", "Windows error during printing", "Memory error during printing", "Print dialog error", "Generic print error", "Invalid device refnum", "Device not found", "Device parameter error", "Device unit error", "Cannot open device", "Device call aborted", "Generic error", "Cancelled by user", "Object ID too low", "Object ID too high", "Object not in heap", "Unknown heap", "Unknown object (invalid DefProc)", "Unknown object (DefProc not in table)", "Message out of range", "Invalid (null) method", "Unknown message", "Manager call not supported", "Bad address", "Network operation in progress", "Network operation timed out", "Connection is busy", "Network attribute not supported", "Network error", "Address in use", "System out of memory", "Connection aborted", "Connection refused", "Not connected", "Already connected", "Connection closed", "Initialization error (interapplication manager)", "Bad occurrence", "Wait on unbound occurrence handler", "Occurrence queue overflow", "Datalog type conflict", "Unused", "Unrecognized type (interapplication manager)", "Memory corrupt", "Failed to make temporary DLL", "Old CIN version", "Drag socket not found", "Failed to load drop-object", "Failed to register OLE object", "Failed to release OLE object", "Format specifier type mismatch", "Unknown format specifier", "Too few format specifiers", "Too many format specifiers", "Scan failed", "Newer CIN version", "Error converting to variant", "Runtime menu error", "Password tampered", "Variant attribute not found", "Incompatible variant data type", "Event data is not available", "Event Store is not present", "Occurrence is not found", "Event Queue is not created", "Event info is not available", "Refnum passed is NULL", "Error retrieving Class GUID", "Error retrieving CoClass GUID", "Error retrieving TypeLib GUID.", "Bad built application magic bytes.", "Specific driver is different from the specific driver associated with the Logical Name.", "There is no session opened to the class driver.", "Max Error", "MAX - Error with config objects", "MAX - Error loading configuration", "MAX - Group not supported"]
        # "Current State"
        # "Do not delete, rename, or modify this frame.\n(this is used to capture unhandled states and typos)"
        # "Handle mistyped state name (developer tool)"
        n11 = Format Into String(format string="Software Exception: Unhandled State \"%s\"." ("message"), error in=w100, w95) -> (resulting string=w103:string, error out=w102:errorcluster)  [unwired: 1 in]
        n12 = call <vilib>:"Error Cluster From Error Code.vi"("show call chain? (False)"=TRUE, "error in (no error)"=w102, "error message (\"\")"=w103, "error code (0)"=w104) -> ("error out"=w101:errorcluster)  [unwired: 5 in]
        n13 = call <vilib>:"Add State(s) to Queue__jki_lib_state_machine.vi"("State(s) in (\"\")"=w99) -> ("States Out"=w98:string)  [unwired: 14 in]
      }
      frame "Error Handler" {
        # "Unhandled Error -- Display it"
        # "Handle any errors here.\nYou can also output any states to clean-up after errors occur"
        # "Clear error"
        n14 = call <vilib>:"General Error Handler.vi"("error in (no error)"=w107) -> ()  [unwired: 10 in, 5 out]
        n15 = call <vilib>:"Add State(s) to Queue__jki_lib_state_machine.vi"("State(s) in Front (\"\")"="/* Post Error States", "State(s) in (\"\")"=w111) -> ("States Out"=w110:string)  [unwired: 13 in]
      }
      frame "Exit" {
        n16 = Unbundle By Name(w116) -> ("File"=w114:path)
        n17 = Equal?(x=w114, y=path "") -> (x = y?=w113:bool)
        n18 = case shown="False" w113 {
          tunnel: ["Macro: Initialize" "Exit"] -> w112
          frame False {
          }
          frame True {
          }
        }
        n19 = Bundle By Name(cluster=w116, "SM Action"=w112) -> (w117:cluster{"File":path, "SM Action":string})
        n20 = call <vilib>:"Add State(s) to Queue__jki_lib_state_machine.vi"("State(s) in (\"\")"=w121) -> ("States Out"=w120:string)  [unwired: 14 in]
      }
      frame "---------- Data ----------" {
        # "Do not put any code in this frame.\n(It is a separator no-op. You can make a copy of this frame to create a new Data frame)"
        n21 = call <vilib>:"Add State(s) to Queue__jki_lib_state_machine.vi"("State(s) in (\"\")"=w127) -> ("States Out"=w126:string)  [unwired: 14 in]
      }
      frame "Data: Initialize" {
        n22 = while {
          tunnel: [w139] -> w129
          tunnel: [w138] -> w128
          stop <- w135 stop-if-true
          w138 = ""  # SM Action
          w139 = path ""  # File
          n23 = call "UTILITY Boolean Notifier.vi"("Status"=UTILITY_Notifier."Read", "Set Status"=FALSE, "name (unnamed)"="Start UI Loop") -> ("latest READ notification"=w135:bool)  [unwired: 7 in, 1 out]
          n24 = Wait Until Next ms Multiple(millisecond multiple=u32 250) -> ()  [unwired: 1 out]
        }
        n25 = Bundle("File"=w129, "SM Action"=w128) -> (w131:cluster{"File":path, "SM Action":string})  [unwired: 1 in]
        n26 = call <vilib>:"Add State(s) to Queue__jki_lib_state_machine.vi"("State(s) in (\"\")"=w133) -> ("States Out"=w132:string)  [unwired: 14 in]
      }
      frame "---------- Macro ----------" {
        # "Do not put any code in this frame.\n(It is a separator no-op. You can make a copy of this frame to create a new Macro frame)"
        n27 = call <vilib>:"Add State(s) to Queue__jki_lib_state_machine.vi"("State(s) in (\"\")"=w144) -> ("States Out"=w143:string)  [unwired: 14 in]
      }
      frame "Macro: Initialize" {
        n28 = call <vilib>:"Add State(s) to Queue__jki_lib_state_machine.vi"("State(s) in Front (\"\")"="Data: Initialize", "State(s) in (\"\")"=w149) -> ("States Out"=w148:string)  [unwired: 13 in]
      }
      frame "---------- Write To File ----------" {
        n29 = call <vilib>:"Add State(s) to Queue__jki_lib_state_machine.vi"("State(s) in (\"\")"=w153) -> ("States Out"=w152:string)  [unwired: 14 in]
      }
      frame "Check File" {
        n30 = local read "Save File Path"() -> (w156:path)
        n31 = Equal?(x=w156, y=path "") -> (x = y?=w155:bool)
        n32 = case shown="True" w155 {
          tunnel: ["Exit" ""] -> w154
          frame False {
          }
          frame True {
          }
        }
        n33 = Bundle By Name(cluster=w159, "File"=w156) -> (w158:cluster{"File":path, "SM Action":string})
        n34 = call <vilib>:"Add State(s) to Queue__jki_lib_state_machine.vi"("State(s) in Front (\"\")"=w154, "State(s) in (\"\")"=w162) -> ("States Out"=w161:string)  [unwired: 13 in]
      }
      frame "Check Exit" {
        n35 = local read "Shutdown Sequence"() -> (w165:string)
        n36 = call <vilib>:"Add State(s) to Queue__jki_lib_state_machine.vi"("State(s) in Front (\"\")"=w165, "State(s) in (\"\")"=w169) -> ("States Out"=w168:string)  [unwired: 13 in]
      }
    }
  }
  n37 = flat-sequence {
    tunnel: ["Macro: Initialize"] -> w61
    frame #0 {
      w173 = TRUE ("Visible")
      w175 = FALSE ("Start Heat Up Test")
      w176 = FALSE ("24 Hr Test Complete")
      w181 = FALSE ("Visible")
      w185 = FALSE ("Write To File")
      n38 = local read "Plot File"() -> (w170:path)
      n39 = property on="Start 24 Hour Rating" class="Bool"("Visible"=w173) -> ()  [unwired: 2 in, 2 out]
      n40 = property on="Start First Hour Rating" class="Bool"("Visible"=w173) -> ()  [unwired: 2 in, 2 out]
      n41 = property on="Start Heat Up Test" class="Bool (strict)"("Visible"=w173) -> ()  [unwired: 2 in, 2 out]
      n42 = Bundle By Name(cluster="Program Names", "Stand Override"=TRUE) -> (w182:T25)
      n43 = call-poly <vilib>:"Write To Spreadsheet File.vi"("delimiter (\\t)"="," ("delimiter (\\t)"), "file path (dialog if empty)"=w170) -> ()  [unwired: 6 in, 1 out]
      n44 = local write "DAQ Loop Complete"(FALSE ("DAQ Loop Complete")) -> ()
      n45 = local write "Start Value Signal Data Table"(FALSE ("Start Value Signal Data Table")) -> ()
      n46 = local write "24 Hr Test Complete"(w176) -> ()
      n47 = property on="Quit" class="Bool (strict)"("Value"=w176) -> ()  [unwired: 2 in, 2 out]
      n48 = local write "Start Heat Up Test"(w175) -> ()
      n49 = local write "Stop Custom Draw"(w175) -> ()
      n50 = local write "Write To File Change"(w175) -> ()
      n51 = local write "Program Names Update"(w182) -> ()
      n52 = local write "Program Names"(w182) -> ()
      n53 = local write "Intellifaucet Type"("" ("Shutdown")) -> ()
      n54 = local write "Start Draw Timer"(FALSE ("Start Draw Timer")) -> ()
      n55 = local write "Purge Time (Seconds)"(T19 180.0 ("Purge Time (Seconds)")) -> ()
      n56 = property on="Flow Meter" class="WFChart (strict)"("Visible"=w181) -> ()  [unwired: 2 in, 2 out]
      n57 = property on="Average TC Tree Temperature" class="WFChart (strict)"("Visible"=w181) -> ()  [unwired: 2 in, 2 out]
      n58 = local write "Scan Rate (Seconds)"(T19 3.0 ("Scan Rate (Seconds)")) -> ()
      n59 = property on="Total Dispensed Gallons" class="WFChart (strict)"("Visible"=w181) -> ()  [unwired: 2 in, 2 out]
      n60 = local write "Shutdown"("" ("Shutdown")) -> ()
      n61 = local write "HEWH Power"(TRUE ("HEWH Power")) -> ()
      n62 = local write "Shutdown DAQ"("") -> ()
      n63 = local write "Quit"(T31 FALSE ("Quit")) -> ()
      n64 = local write "Multi-Draw"(FALSE ("Mult-Draw")) -> ()
      n65 = local write "Shutdown Sequence"("" ("Shutdown Sequence")) -> ()
      n66 = local write "Heat Up Step 4 Flag"(FALSE ("Skip Purge")) -> ()
      n67 = local write "Save File Path"(path "" ("Save File Path")) -> ()
      n68 = local write "Draw Count"(u8 0) -> ()
      n69 = local write "Remaining Draws"(T22 1 ("Remaining Draws")) -> ()
      n70 = local write "Start DAQ Write"(w185) -> ()
      n71 = local write "Write To File"(w185) -> ()
      n72 = local write "Draw Time"(T20 0.0 ("Draw Time")) -> ()
      "Start UI Loop" <- FALSE
      "Message" <- T23 "" ("Message")
    }
  }
  n73 = call "UTILITY Boolean Notifier.vi"("Status"=UTILITY_Notifier."Set", "error in (no error)"="Error In", "Set Status"=FALSE, "name (unnamed)"="Full Cutout") -> ("error out"=w4:errorcluster)  [unwired: 6 in, 1 out]
  n74 = call "UTILITY Boolean Notifier.vi"("Status"=UTILITY_Notifier."Set", "error in (no error)"=w4, "Set Status"=TRUE, "name (unnamed)"="Pressurize Tank?") -> ("error out"=w9:errorcluster)  [unwired: 6 in, 1 out]
  n75 = Merge Errors() -> (→"Error Out 2":errorcluster)  [unwired: 2 in]
  n76 = call "HEWH_DSM_CMD.vi"("GEA2 Commands and Requests"=w52) -> ("Input Data"=w49:T59)  [unwired: 8 in, 1 out]
  n77 = Unbundle By Name(w49) -> ("Source"=w41:u8)
  n78 = call "GEA2 Initialize.vi"("Board Index"=0, "Source Address"=w41) -> ("GEA2 Reference Out"=w51:refnum<k24>, "error out"=w44:errorcluster)  [unwired: 11 in, 1 out]
  n79 = call "UTILITY Boolean Notifier.vi"("Status"=UTILITY_Notifier."Set", "error in (no error)"=w9, "Set Status"=FALSE, "name (unnamed)"="Stop Custom Draw") -> ("error out"=w13:errorcluster)  [unwired: 6 in, 1 out]
  n80 = call <vilib>:"Add State(s) to Queue__jki_lib_state_machine.vi"("State(s) in (\"\")"="Macro: Initialize") -> ("States Out"=w57:string)  [unwired: 14 in]
  n81 = Unbundle By Name(w31) -> ("SM Action"=w29:string, "File"=w30:path)
  n82 = call "UTILITY Boolean Notifier.vi"("Status"=UTILITY_Notifier."Set", "Set Status"=FALSE, "name (unnamed)"="First Hour Cutout") -> ()  [unwired: 7 in, 2 out]
  n83 = while {
    tunnel: "24HR Error In" -> [w202]
    tunnel: [w200] -> w2
    stop <- w204 stop-if-true
    # "Wait for Heat Source Cutout: Step 1"
    n84 = Wait Until Next ms Multiple(millisecond multiple=u32 100) -> ()  [unwired: 1 out]
    n85 = call "UTILITY String Notifier.vi"("Status"=UTILITY_Notifier."Set", "error in (no error)"=w202, "Set Status"="Waiting for Heat Source Cutout....", "name (unnamed)"="Message") -> ("error out"=w201:errorcluster)  [unwired: 6 in, 1 out]
    n86 = call "UTILITY Boolean Notifier.vi"("Status"=UTILITY_Notifier."Read", "error in (no error)"=w201, "name (unnamed)"="Full Cutout") -> ("error out"=w200:errorcluster, "latest READ notification"=w204:bool)  [unwired: 7 in]
  }
  n87 = Equal?(x=w30, y=path "") -> (x = y?=w34:bool)
  n88 = call <vilib>:"Add State(s) to Queue__jki_lib_state_machine.vi"("State(s) in (\"\")"=w29) -> ("States Out"=w39:string)  [unwired: 14 in]
  n89 = call "UTILITY Boolean Notifier.vi"("Status"=UTILITY_Notifier."Set", "error in (no error)"=w13, "Set Status"=FALSE, "name (unnamed)"="Start UI Loop") -> ("error out"=w25:errorcluster)  [unwired: 6 in, 1 out]
  n90 = while "Data Acquisition Loop" {
    shift-right: [w222] -> w48
    shift-left: _ -> [w221]
    shift-right: [w225] -> w45
    shift-left: w44 -> [w220]
    shift-right: [w224] -> _
    shift-left: w57 -> [w226]
    tunnel: w52 -> [w213]
    tunnel: w49 -> [w210]
    tunnel: w51 -> [w212]
    tunnel: [w211] -> w50
    stop <- w223 stop-if-true
    # "Data Acquisition Loop"
    n91 = local read "Use Agilent?"() -> (w216:bool)
    n92 = case shown="False" w216 {
      tunnel: "Scan Rate Adjust" -> [w232 w237]
      tunnel: [w230 w234] -> w214
      frame False {
        n93 = In Range and Coerce(upper limit=inf, x=w232, lower limit=1.0) -> (coerced(x)=w230:T19)  [unwired: 1 out]
      }
      frame True {
        n94 = In Range and Coerce(upper limit=inf, x=w237, lower limit=2.0) -> (coerced(x)=w234:T19)  [unwired: 1 out]
      }
    }
    n95 = local read "Newfi Time"() -> (w218:dbl)
    n96 = local read "Start Time"() -> (w219:dbl)
    n97 = call "UTILITY Timeout Calc.vi"(9:w218, "Gather Data Period"=w214, 11:w219) -> ("coerced(x)"=w217:i32)  [unwired: 7 in, 1 out]
    n98 = call <vilib>:"Parse State Queue__jki_lib_state_machine.vi"("State Queue"=w226, "Error In (no error)"=w220) -> ("Remaining States"=w228:string, "Current State"=w229:string, "Arguments"=w227:string)  [unwired: 11 in]
    n99 = case shown="\"Get Final Data\"" w229 {
      selector: w229 -> [_ _ w279 _ _ _ _ _ _ _ _ _ _ _ _ _ _ _ _ _]
      tunnel: w228 -> [w245 w277 w283 w296 w304 w309 w320 w336 w347 w352 w358 w363 w379 w408 w463 w474 w494 w514 w527 w533]
      tunnel: w227 -> [_ _ _ _ _ _ _ _ _ _ _ _ _ _ _ _ _ _ _ _]
      tunnel: w221 -> [w243 w274 w281 w293 w302 w306 _ w333 w345 w349 w355 w360 w366 w405 w453 w469 w481 w511 w526 w532]
      tunnel: [w242 w275 w285 errorcluster {"status"=FALSE, "code"=0, "source"=""} ("error out") w301 w307 w317 w334 w338 w350 w356 w361 w377 w395 w454 w472 w487 w512 w528 w534] -> w225
      tunnel: w220 -> [w241 w275 w284 w292 w301 w307 w317 w334 w339 w350 w356 w361 w377 w398 w447 w472 w488 w512 w528 w534]
      tunnel: [w244 w276 w282 w295 w303 w308 w319 w335 w346 w351 w357 w362 w378 w407 w462 w473 w493 w513 w529 w535] -> w224
      tunnel: [_ _ _ _ w299 _ _ _ _ _ _ _ _ _ _ _ _ _ _ _] -> w223
      tunnel: [w240 w274 w281 w293 w302 w306 w318 w333 w345 w349 w355 w360 w365 w406 w452 w468 w481 w511 w521 w532] -> w222
      tunnel: w217 -> [w239 _ _ _ _ _ _ _ _ _ _ _ _ _ _ _ _ _ _ _]
      tunnel: w213 -> [_ _ _ _ _ _ _ _ _ _ _ _ _ _ w445 _ _ _ _ _]
      tunnel: w212 -> [w238 w273 w278 w290 w300 w305 w310 w332 w337 w348 w353 w359 w364 w394 w444 w466 w490 w509 w519 w530]
      tunnel: [w238 w273 w278 w290 w300 w305 w310 w332 w337 w348 w353 w359 w364 w394 w443 w466 w490 w509 w519 w530] -> w211
      tunnel: w210 -> [_ _ _ _ _ _ _ _ _ _ _ _ _ _ w442 _ _ _ _ _]
      frame "", "Idle" {
        n100 = event shown="[0] Timeout" {
          selector: _ -> [_ _]
          dyn-events: _ -> [_ _]
          timeout: w239 -> [_ _]
          tunnel: w245 -> [w254 w272]
          tunnel: [w249 w272] -> w244
          tunnel: w243 -> [w252 w270]
          tunnel: [w253 w271] -> w242
          tunnel: w241 -> [w253 w271]
          tunnel: [w252 w269] -> w240
          event Timeout {
            # "Pause the main data collection routine during pre-draw"
            n101 = event-data() -> ()  [unwired: 1 in, 1 out]
            n102 = local read item#-1() -> (w246)
            n103 = case shown="False" w246 {
              tunnel: [w257 ""] -> w247
              frame False {
                n104 = local read "Write To File Change"() -> (w255:bool)
                n105 = local read "Start DAQ Write"() -> (w256:bool)
                n106 = case shown="True" w256 {
                  tunnel: ["Time\nCollect Data\nGet Newfi Data\nUpdate Power Display" w260] -> w257
                  tunnel: w255 -> [_ w259]
                  frame False {
                  }
                  frame True {
                    n107 = case shown="True" w259 {
                      tunnel: ["Time\nCollect Data\nGet Newfi Data\nUpdate Power Display\nWrite Data" "Time\nCollect Data\nGet Newfi Data\nUpdate Power Display\nCheck Write Timer\nWrite Data"] -> w260
                      frame False {
                      }
                      frame True {
                      }
                    }
                  }
                }
              }
              frame True {
              }
            }
            n108 = local read "Shutdown DAQ"() -> (w248:string)
            n109 = call <vilib>:"Add State(s) to Queue__jki_lib_state_machine.vi"("State(s) in Front (\"\")"=w247, "State(s) in (\"\")"=w254) -> ("States Out"=w251:string)  [unwired: 13 in]
            n110 = call <vilib>:"Add State(s) to Queue__jki_lib_state_machine.vi"("State(s) in Front (\"\")"=w248, "State(s) in (\"\")"=w251) -> ("States Out"=w250:string)  [unwired: 13 in]
            n111 = flat-sequence {
              tunnel: w250 -> [w265]
              tunnel: [w265] -> w249
              frame #0 {
                n112 = local write "Shutdown DAQ"("" ("Shutdown")) -> ()
              }
            }
          }
          event Value Change {
            # "The scan rate uses a  control loop to insure it has the \nbest timing...this adjustment get the rate in the ball park...\nwhen i simply put the  scan rate into the timeout\nbox...it give weird scans..."
            n113 = event-data() -> ("NewVal"=w268:T19)  [unwired: 1 in, 5 out]
            n114 = Multiply(x=w268, y=T19 1000.0) -> (x*y=w266:T19)
            n115 = Bundle By Name(cluster=w270, "Core HEWH Data DAQ LOOP.Scan Rate Adjust"=w266) -> (w269:T61)
          }
        }
      }
      frame "---------- Core ----------" {
        # "Do not put any code in this frame.\n(it is a separator no-op)"
        n116 = call <vilib>:"Add State(s) to Queue__jki_lib_state_machine.vi"("State(s) in (\"\")"=w277) -> ("States Out"=w276:string)  [unwired: 14 in]
      }
      frame Default {
        w288 = 42 items=["No error", "Argument error", "Memory is full", "Out of zone", "End of file", "File already open", "Generic file I/O error", "File not found", "File permission error", "Disk is full", "Duplicate path", "Too many files open", "System feature not enabled", "Resource file not found", "Cannot add resource", "Resource not found", "Image not found", "Image memory error", "Pen does not exist", "Config type invalid", "Config token not found", "Config parse error", "Config memory error", "Bad external code format", "Bad external code offset", "External code not present", "Null window", "Destroy window error", "Null menu", "Print aborted", "Bad print record", "Print driver error", "Windows error during printing", "Memory error during printing", "Print dialog error", "Generic print error", "Invalid device refnum", "Device not found", "Device parameter error", "Device unit error", "Cannot open device", "Device call aborted", "Generic error", "Cancelled by user", "Object ID too low", "Object ID too high", "Object not in heap", "Unknown heap", "Unknown object (invalid DefProc)", "Unknown object (DefProc not in table)", "Message out of range", "Invalid (null) method", "Unknown message", "Manager call not supported", "Bad address", "Network operation in progress", "Network operation timed out", "Connection is busy", "Network attribute not supported", "Network error", "Address in use", "System out of memory", "Connection aborted", "Connection refused", "Not connected", "Already connected", "Connection closed", "Initialization error (interapplication manager)", "Bad occurrence", "Wait on unbound occurrence handler", "Occurrence queue overflow", "Datalog type conflict", "Unused", "Unrecognized type (interapplication manager)", "Memory corrupt", "Failed to make temporary DLL", "Old CIN version", "Drag socket not found", "Failed to load drop-object", "Failed to register OLE object", "Failed to release OLE object", "Format specifier type mismatch", "Unknown format specifier", "Too few format specifiers", "Too many format specifiers", "Scan failed", "Newer CIN version", "Error converting to variant", "Runtime menu error", "Password tampered", "Variant attribute not found", "Incompatible variant data type", "Event data is not available", "Event Store is not present", "Occurrence is not found", "Event Queue is not created", "Event info is not available", "Refnum passed is NULL", "Error retrieving Class GUID", "Error retrieving CoClass GUID", "Error retrieving TypeLib GUID.", "Bad built application magic bytes.", "Specific driver is different from the specific driver associated with the Logical Name.", "There is no session opened to the class driver.", "Max Error", "MAX - Error with config objects", "MAX - Error loading configuration", "MAX - Group not supported"]
        # "Current State"
        # "Do not delete, rename, or modify this frame.\n(this is used to capture unhandled states and typos)"
        # "Handle mistyped state name (developer tool)"
        n117 = Format Into String(format string="Software Exception: Unhandled State \"%s\"." ("message"), error in=w284, w279) -> (resulting string=w287:string, error out=w286:errorcluster)  [unwired: 1 in]
        n118 = call <vilib>:"Error Cluster From Error Code.vi"("show call chain? (False)"=TRUE, "error in (no error)"=w286, "error message (\"\")"=w287, "error code (0)"=w288) -> ("error out"=w285:errorcluster)  [unwired: 5 in]
        n119 = call <vilib>:"Add State(s) to Queue__jki_lib_state_machine.vi"("State(s) in (\"\")"=w283) -> ("States Out"=w282:string)  [unwired: 14 in]
      }
      frame "Error Handler" {
        # "Unhandled Error -- Display it"
        # "Handle any errors here.\nYou can also output any states to clean-up after errors occur"
        # "Clear error"
        n120 = call <vilib>:"General Error Handler.vi"("error in (no error)"=w292) -> ()  [unwired: 10 in, 5 out]
        n121 = call <vilib>:"Add State(s) to Queue__jki_lib_state_machine.vi"("State(s) in Front (\"\")"="/* Post Error States", "State(s) in (\"\")"=w296) -> ("States Out"=w295:string)  [unwired: 13 in]
      }
      frame "Exit" {
        w299 = TRUE
        # "Do not put any code in this frame.\n(No errors that occur here will be handled.)"
        n122 = local read "Plot File"() -> (w298:path)
        n123 = call-poly <vilib>:"Write To Spreadsheet File.vi"("delimiter (\\t)"="," ("delimiter (\\t)"), "file path (dialog if empty)"=w298) -> ()  [unwired: 6 in, 1 out]
        n124 = call <vilib>:"Add State(s) to Queue__jki_lib_state_machine.vi"("State(s) in (\"\")"=w304) -> ("States Out"=w303:string)  [unwired: 14 in]
        "DAQ Loop Complete" <- w299
      }
      frame "---------- Data ----------" {
        # "Do not put any code in this frame.\n(It is a separator no-op. You can make a copy of this frame to create a new Data frame)"
        n125 = call <vilib>:"Add State(s) to Queue__jki_lib_state_machine.vi"("State(s) in (\"\")"=w309) -> ("States Out"=w308:string)  [unwired: 14 in]
      }
      frame "Data: Initialize" {
        # "Initialize the shift-register data, here.\n(data names are defined by what you wire into the bundle function)"
        n126 = while {
          tunnel: [w330] -> w316
          tunnel: [w329] -> w315
          tunnel: [w325] -> w314
          tunnel: [w328] -> w313
          tunnel: [w327] -> w312
          tunnel: [w326] -> w311
          stop <- w322 stop-if-true
          w325 = T60 {"GEA2 Reference Out"=refnum, "Data In"={"Source"=0, "Destination"=0, "Command"=0, "Message"=""}, "Water Heater GEA2 Data"={"GEA2 Label Array"=[], "PID_PARAMETERS"=[], "SUPPORTED_MODES"=[], "Button Status"={"Switch 1"=FALSE, "Switch 2"=FALSE, "Switch 3"=FALSE, "Switch 4"=FALSE, "Switch 5"=FALSE, "Switch 6"=FALSE, "Switch 7"=FALSE, "Switch 8"=FALSE, "Switch 9"=FALSE, "Switch 10"=FALSE, "Switch 11"=FALSE, "Switch 12"=FALSE, "Switch 13"=FALSE, "Switch 14"=FALSE, "Switch 15"=FALSE, "Switch 16"=FALSE}, "Status Query"={"Days Remaining (For Std Electric and Vacation)"=0, "Unit Status"="", "Current Tank Temp in Deg F"=0, "Current Setpoint in Deg F"=0, "Filter Status (% used)"=0, "Fallback Status (Fallback heating mode)"="", "Fallback Temp"=0, "\"Set Mode\" Selection"=""}, "Service Error Codes"={"Reserved"=FALSE, "Reserved 1"=FALSE, "Reserved 2"=FALSE, "Reserved 3"=FALSE, "Reserved 4"=FALSE, "Reserved 5"=FALSE, "Reserved 6"=FALSE, "Reserved 7"=FALSE, "DataFlash Fail Status"=FALSE, "Stuck Key Fail Status"=FALSE, "Dry Tank Fail Status"=FALSE, "Miswire Fail Status"=FALSE, "Reserved 8"=FALSE, "Reserved 9"=FALSE, "Reserved 10"=FALSE, "Reserved 11"=FALSE, "UE Fail Status"=FALSE, "LE Fail Status"=FALSE, "Filter Fail Status"=FALSE, "T3A Fail Status"=FALSE, "T3B Fail Status"=FALSE, "T4 Fail Status"=FALSE, "T5 Fail Status"=FALSE, "T2 Fail Status"=FALSE, "SS Cond A Status"=FALSE, "SS Cond B Status"=FALSE, "SS Cond C Status"=FALSE, "SS Cond D Status"=FALSE, "SS Cond E Status"=FALSE, "SS Cond F Status"=FALSE, "SS Fan Status"=FALSE, "CMP Fail Status"=FALSE}, "HEM_KWH_DATA"=[], "OTHER_FAULT_COUNTS"=[], "GEA2 Raw Message"="", "Hyperterminal Data"={"Source"=0, "Destination"=0, "Command"=0, "Length"=0, "CRC"=0, "UE - state (1/0 on off)"=0, "LE - state (1/0 on off)"=0, "Comp - state (1/0 on off)"=0, "Fan  - state (1/0 on off)"=0, "Setpoint Deg F"=0, "T2(TankSensor)"=0.0, "T3A(EvapIn)"=0.0, "T3B(EvapOut)"=0.0, "T4(CompressorDischarge)"=0.0, "T5(Ambient)"=0.0, "Current"=0.0, "Voltage (Volts)"=0, "EEV Position (0-480)"=0, "Reason for last heating cycle termination"=0, "Reason Data word 1"="", "Reason Data word 2"="", "Reason Data word 3"="", "Reason Data word 4"="", "SW Debug Data"="", "Flow Events (Bit Encoded)"=0, "Heating Control Mode"=0}, "Extra Data"={"Water Capacity (Gallons)"=0, "Max Vacation Duration Days"=0, "Min Vacation Duration Days"=0, "Max Set Point (Deg F)"=0, "Min Set Point (Deg F)"=0, "T5 Resistance"=0, "T4 Resistance"=0, "T3B Resistance"=0, "T2 Resistance"=0, "STD_ELEC_RANGE"="", "SS_FAULT_COUNTS"="", "SERIAL_NUMBER"="", "READ_PERSONALITY"=0, "RQST_OVERRIDE_STATUS"="", "MODEL_SELECT_AD_VALUE"=0, "MODEL NUMBER"="", "IDLB_RESISTANCE"=0, "DSM Override Status"="", "RQST_DATA_FROM_Memory"="", "RQST_DATA_FROM_DATA_FLASH"="", "RQST_CURRENT_PID_SH_TARGET"=0, "Unit System Mode"=""}}, "GEA2 Commands and Requests"=enum."CMD_CANCEL_EEV_POSITION"}  # GEA2 Reference Out
          w329 = string[][] []  # Save Data
          n127 = Wait Until Next ms Multiple(millisecond multiple=u32 250) -> ()  [unwired: 1 out]
          n128 = local read "User Controls DAQ LOOP"() -> (w328:T28)
          n129 = local read "Core HEWH Data DAQ LOOP"() -> (w327:T1)
          n130 = local read "POWER DAQ LOOP"() -> (w326:T12)
          n131 = local read "Equipment VISA"() -> (w330:T40)
          n132 = call "UTILITY Boolean Notifier.vi"("Status"=UTILITY_Notifier."Read", "Set Status"=FALSE, "name (unnamed)"="Start UI Loop") -> ("latest READ notification"=w322:bool)  [unwired: 7 in, 1 out]
        }
        n133 = Bundle("Equipment VISA"=w316, "Save Data"=w315, "GEA2 Reference Out"=w314, "User Controls DAQ LOOP"=w313, "Core HEWH Data DAQ LOOP"=w312, "POWER DAQ LOOP"=w311) -> (w318:T61)  [unwired: 1 in]
        n134 = call <vilib>:"Add State(s) to Queue__jki_lib_state_machine.vi"("State(s) in (\"\")"=w320) -> ("States Out"=w319:string)  [unwired: 14 in]
      }
      frame "---------- UI ----------" {
        n135 = call <vilib>:"Add State(s) to Queue__jki_lib_state_machine.vi"("State(s) in (\"\")"=w336) -> ("States Out"=w335:string)  [unwired: 14 in]
      }
      frame "Get Software Version" {
        w343 = GEA2_Commands."RQST_Software_Version" ("GEA2 Commands and Requests")
        n136 = call "HEWH_DSM_CMD.vi"("GEA2 Commands and Requests"=w343) -> ("Input Data"=w341:T59)  [unwired: 8 in, 1 out]
        n137 = call "Send and Receive Example.vi"("Input Data"=w341, "Error In"=w339) -> ("Coverted Data Out"=w340:T62, "Error Out"=w338:errorcluster)  [unwired: 11 in, 1 out]
        n138 = call "GEA2 Message Decoder.vi"("GEA2 Commands and Requests"=w343, "Coverted Data Out"=w340) -> ("GEA Information Out"=w344:T63)  [unwired: 9 in]
        n139 = Unbundle By Name(w344) -> ("Software String"=w342:string)
        n140 = local write "Sofware Version"(w342) -> ()
        n141 = call <vilib>:"Add State(s) to Queue__jki_lib_state_machine.vi"("State(s) in (\"\")"=w347) -> ("States Out"=w346:string)  [unwired: 14 in]
      }
      frame "---------- Macro ----------" {
        n142 = call <vilib>:"Add State(s) to Queue__jki_lib_state_machine.vi"("State(s) in (\"\")"=w352) -> ("States Out"=w351:string)  [unwired: 14 in]
      }
      frame "Macro: Initialize" {
        n143 = call <vilib>:"Add State(s) to Queue__jki_lib_state_machine.vi"("State(s) in Front (\"\")"="Data: Initialize\nGet Software Version", "State(s) in (\"\")"=w358) -> ("States Out"=w357:string)  [unwired: 13 in]
      }
      frame "---------- Data Collection ----------" {
        n144 = call <vilib>:"Add State(s) to Queue__jki_lib_state_machine.vi"("State(s) in (\"\")"=w363) -> ("States Out"=w362:string)  [unwired: 14 in]
      }
      frame "Time" {
        # "I have found if you use all of the aglient TC's you can only scan at approximately 2s. Only MW100 will allow 1s probably\nfaster..but I limited to 1 sec. This routine also adjusts the scan rate (like a PID controller). I cannot just put in a constant \nvalue...does not seem to work."
        n145 = Unbundle By Name(w366) -> ("Core HEWH Data DAQ LOOP.Scan Rate Adjust"=w370:dbl, "User Controls DAQ LOOP.Use Agilent?"=w374:bool)
        n146 = case shown="False" w374 {
          tunnel: "Scan Rate (Seconds)" -> [w382 w387]
          tunnel: [w380 w384] -> w376
          frame False {
            n147 = In Range and Coerce(upper limit=inf, x=w382, lower limit=1.0) -> (coerced(x)=w380:T19)  [unwired: 1 out]
          }
          frame True {
            n148 = In Range and Coerce(upper limit=inf, x=w387, lower limit=2.0) -> (coerced(x)=w384:T19)  [unwired: 1 out]
          }
        }
        n149 = local read "Newfi Time"() -> (w368:dbl)
        n150 = local write "Scan Rate (Seconds)"(w376) -> ()
        n151 = call "UTILITY E-Time.vi"() -> ("Elapsed Time (sec)"=w367:dbl)  [unwired: 9 in, 2 out]
        "Start Time" <- w367
        n152 = Subtract(x=w367, y=w368) -> (x-y=w369:dbl)
        "Loop Time" <- w369
        n153 = Subtract(x=w369, y=w376) -> (x-y=w372:T19)
        n154 = Less Than 0?(x=w372) -> (x < 0?=w373:bool)
        n155 = case shown="False" w373 {
          tunnel: w370 -> [w390 w391]
          tunnel: [w389 w392] -> w371
          frame False {
            n156 = local read "Timer Step Size"() -> (w388:dbl)
            n157 = Subtract(x=w390, y=w388) -> (x-y=w389:dbl)
            n158 = local write "Scan Rate Adjust"(w389) -> ()
          }
          frame True {
            n159 = Add(x=w391, y="Timer Step Size") -> (x+y=w392:dbl)
            n160 = local write "Scan Rate Adjust"(w392) -> ()
          }
        }
        n161 = Bundle By Name(cluster=w366, "Core HEWH Data DAQ LOOP.Scan Rate Adjust"=w371) -> (w365:T61)
        n162 = call <vilib>:"Add State(s) to Queue__jki_lib_state_machine.vi"("State(s) in (\"\")"=w379) -> ("States Out"=w378:string)  [unwired: 14 in]
      }
      frame "Collect Data" {
        # "Over-Write MW Power \ndata"
        # "I allow the MW100 to run as fast as possible.\nThis is the control loop. It helps with a quicker \nintellifaucet control algorithm. This routine just \ncollects the data periodically"
        n163 = Unbundle By Name(w405) -> ("User Controls DAQ LOOP.Use Agilent?"=w404:bool, "Equipment VISA"=w402:T40, "Core HEWH Data DAQ LOOP"=w403:T1, "Core HEWH Data DAQ LOOP.HEWH Specific DAQ.Power Analyzer"=w401:T14)
        n164 = case shown="True" w404 {
          tunnel: w398 -> [w428 w432]
          tunnel: [w428 w431] -> w397
          tunnel: w403 -> [_ w429]
          tunnel: [string[][] [] ("Agilent Data") w430] -> w399
          frame False {
          }
          frame True {
            n165 = call "HEWH Get Agilent Data.vi"("error in (no error)"=w432, 10:w429) -> ("error out"=w431:errorcluster, 1:w430)  [unwired: 6 in, 2 out]
          }
        }
        n166 = case shown="\"WT300\"" w401 {
          tunnel: w402 -> [_ w416]
          tunnel: [w411 w418] -> w400
          tunnel: w399 -> [w410 w415]
          tunnel: w398 -> [w409 w417]
          tunnel: [w409 w413] -> w396
          frame "OSI", Default {
            n167 = local read "MW100 Data"() -> (w412:string[][])
            n168 = Build Array (concatenate)(w412, w410) -> (w411:string[][])
          }
          frame "WT300" {
            n169 = local read "MW100 Data"() -> (w425:string[][])
            n170 = Unbundle By Name(w416) -> ("WT210"=w426:refnum<visa-resource-name>)
            n171 = call "WT300 Get Data.vi"("error in (no error)"=w417, "VISA resource name"=w426) -> ("error out"=w414:errorcluster, "Power Data"=w423:T67)  [unwired: 4 in, 4 out]
            n172 = Unbundle By Name(w423) -> ("Voltage (V):Element 1"=w422:dbl, "Current (A):Element 1"=w421:dbl, "Power (W):Sigma"=w420:dbl, "Watt Hours (Wh):Sigma"=w419:dbl)
            n173 = call "HEWH WT210 Data Save.vi"("MW100 Data"=w425, "output cluster"=w423) -> ("MW100 Data"=w424:string[][])  [unwired: 9 in]
            n174 = local write "Voltage (Volts)"(w422) -> ()
            n175 = local write "Current"(w421) -> ()
            n176 = local write "Power (Watts)"(w420) -> ()
            n177 = local write "Watt Hours (Wh)"(w419) -> ()
            n178 = Build Array (concatenate)(w424, w415) -> (w418:string[][])
            n179 = call <vilib>:"Clear Errors.vi"("error in (no error)"=w414) -> ("error out"=w413:errorcluster)  [unwired: 5 in, 1 out]
          }
        }
        n180 = Bundle By Name(cluster=w405, "Save Data"=w400) -> (w406:T61)
        n181 = Merge Errors(w397, w396) -> (w395:errorcluster)
        n182 = call <vilib>:"Add State(s) to Queue__jki_lib_state_machine.vi"("State(s) in (\"\")"=w408) -> ("States Out"=w407:string)  [unwired: 14 in]
      }
      frame "Get Newfi Data" {
        # "Get GEA2 Data"
        n183 = Unbundle By Name(w453) -> ("Save Data"=w456:string[][])
        n184 = local read "Draw Time"() -> (w451:T20)
        n185 = call "GEA2 Send and Receive Message.vi"("GEA2 Reference In"=w444, "Input Data"=w442, "Error In"=w447) -> ("GEA2 Reference Out"=w443:refnum<k24>, "Converted Data Out"=w435:T62, "Error Out"=w446:errorcluster)  [unwired: 7 in, 3 out]
        n186 = Number To Fractional String(number=w451) -> (F-format string=w449:string)  [unwired: 3 in]
        n187 = call "GEA2 Message Decoder.vi"("GEA2 Commands and Requests"=w445, "Coverted Data Out"=w435) -> ("GEA Information Out"=w433:T63)  [unwired: 9 in]
        "Water Heater GEA2 Data" <- w433
        n188 = Unbundle By Name(w433) -> ("Water Heater GEA2 Data.GEA2 Label Array"=w436:string[], "GEA2 Data"=w441:string[])
        n189 = call "UTILITY System Time.vi"() -> ("System Time"=w434:string[])  [unwired: 10 in, 1 out]
        n190 = local read "Elapsed Time"() -> (w457:T20)
        n191 = Build Array("Draw Elapsed Time (s)" ("Serial Data 2"), w449) -> (w448:string[])
        n192 = Number To Fractional String(number=w457) -> (F-format string=w458:string)  [unwired: 3 in]
        n193 = Build Array("Elapsed Time (s)" ("Serial Data 2"), w458) -> (w460:string[])
        n194 = Build Array(w436, w441) -> (w440:string[][])
        n195 = local read "Start Value Signal Data Table"() -> (w437:bool)
        n196 = Build Array(w434, w448, w460) -> (w461:string[][])
        n197 = Transpose 2D Array(2D array=w440) -> (transposed array=w439:string[][])
        n198 = Build Array (concatenate)(w461, w439, w456) -> (w438:string[][])
        "Data Table" <- w438
        n199 = Bundle By Name(cluster=w453, "Core HEWH Data DAQ LOOP.Test Output Data.Data Table"=w438, "GEA2 Reference Out.Water Heater GEA2 Data"=w433) -> (w452:T61)
        n200 = case shown="True" w437 {
          tunnel: w438 -> [_ w464]
          frame False {
          }
          frame True {
            n201 = property on="Data Table Sig" class="Arr (strict)"("Val(Sgnl)"=w464) -> ()  [unwired: 2 in, 2 out]
          }
        }
        n202 = call "UTILITY E-Time.vi"("error in (no error)"=w446) -> ("error out"=w454:errorcluster, "Elapsed Time (sec)"=→"Newfi Time":dbl)  [unwired: 8 in, 1 out]
        n203 = call <vilib>:"Add State(s) to Queue__jki_lib_state_machine.vi"("State(s) in (\"\")"=w463) -> ("States Out"=w462:string)  [unwired: 14 in]
      }
      frame "Update Power Display" {
        n204 = Unbundle By Name(w469) -> ("User Controls DAQ LOOP.GEA2?"=w471:bool, "POWER DAQ LOOP"=w470:T12, "GEA2 Reference Out.Water Heater GEA2 Data"=w465:T36)
        n205 = case shown="True" w471 {
          tunnel: w470 -> [w475 w480]
          tunnel: [w475 w476] -> w467
          tunnel: w465 -> [_ w479]
          frame False {
            # "If no GEA2, let the control loop take care of the display."
          }
          frame True {
            n206 = call "HEWH Update Power Display.vi"("Water Heater GEA2 Data"=w479, "POWER DAQ LOOP in"=w480) -> ("POWER DAQ LOOP out"=w476:T12)  [unwired: 9 in]
            n207 = local write "POWER"(w476) -> ()
            n208 = call "HEWH Power Notifier.vi"("Status"=UTILITY_Notifier."Set", "Set Status"=w476, "name (unnamed)"="Power") -> ()  [unwired: 7 in, 2 out]
          }
        }
        n209 = Bundle By Name(cluster=w469, "POWER DAQ LOOP"=w467) -> (w468:T61)
        n210 = call <vilib>:"Add State(s) to Queue__jki_lib_state_machine.vi"("State(s) in (\"\")"=w474) -> ("States Out"=w473:string)  [unwired: 14 in]
      }
      frame "Write Data" {
        # "I use this array\nto plot on the analysis\ntab"
        # "I use the collection as you go technique for stand override currently. If its a full test..I wait until the end to put\nheaders on. (The file will collect...it will just be over written)"
        n211 = Unbundle By Name(w481) -> ("Core HEWH Data DAQ LOOP.Test Output Data.Data Table"=w486:string[][], "File Path"=→"Save File Path")
        n212 = Delete From Array(array=w486, index (col)=0 ("disabled index (col)")) -> (deleted portion=w489:string[])  [unwired: 2 in, 1 out]
        "Header Info" <- w489
        n213 = Delete From Array(array=w486, index (col)=1 ("disabled index (col)")) -> (deleted portion=w484:string[])  [unwired: 2 in, 1 out]
        n214 = First Call?() -> (First Call?: T/F=w482:bool)
        n215 = case shown="False" w482 {
          tunnel: w489 -> [_ w501]
          tunnel: w488 -> [w499 w508]
          tunnel: [w499 w508] -> w487
          tunnel: w484 -> [w495 w500]
          tunnel: "Plot File" -> [w496 w502]
          frame False {
            n216 = call-poly <vilib>:"Write To Spreadsheet File.vi"("delimiter (\\t)"="," ("delimiter (\\t)"), "append to file? (new file:F)"=TRUE, "1D data"=w495, "file path (dialog if empty)"=w496) -> ()  [unwired: 4 in, 1 out]
          }
          frame True {
            n217 = property on="Y-Axis" class="CmbBox"("Strings[]"=w501) -> ()  [unwired: 2 in, 2 out]
            n218 = property on="X-Axis" class="CmbBox"("Strings[]"=w501) -> ()  [unwired: 2 in, 2 out]
            n219 = call-poly <vilib>:"Write To Spreadsheet File.vi"("delimiter (\\t)"="," ("delimiter (\\t)"), "append to file? (new file:F)"=TRUE, "1D data"=w501, "file path (dialog if empty)"=w502) -> ("new file path (Not A Path if cancelled)"=w503:path)  [unwired: 4 in]
            n220 = call-poly <vilib>:"Write To Spreadsheet File.vi"("delimiter (\\t)"="," ("delimiter (\\t)"), "append to file? (new file:F)"=TRUE, "1D data"=w500, "file path (dialog if empty)"=w503) -> ()  [unwired: 4 in, 1 out]
          }
        }
        n221 = call <vilib>:"Add State(s) to Queue__jki_lib_state_machine.vi"("State(s) in (\"\")"=w494) -> ("States Out"=w493:string)  [unwired: 14 in]
      }
      frame "Check Write Timer" {
        n222 = local read "Continuous Data Collection Output"() -> (w510:bool)
        n223 = case shown="False" w510 {
          frame False {
            n224 = local read "Elapsed Time Output"() -> (w515:T20)
            n225 = local read "Elapsed Time"() -> (w516:T20)
            n226 = Greater?(x=w516, y=w515) -> (0:w517:bool)
            n227 = case shown="True" w517 {
              frame False {
              }
              frame True {
                # "Stop Test and add headers"
                n228 = local write "Shutdown"("Add Headers" ("Shutdown")) -> ()
              }
            }
          }
          frame True {
          }
        }
        n229 = call <vilib>:"Add State(s) to Queue__jki_lib_state_machine.vi"("State(s) in (\"\")"=w514) -> ("States Out"=w513:string)  [unwired: 14 in]
      }
      frame "Update FileInit Cluster" {
        # "Due to the reset, i have to\nreinitialize the scan rate adjust \nvalue"
        # "This state is only updated\nwhen you complete the FileInit Setup and after PreDraw"
        # "I update these values because I dont require a File setup screen until you \nstart writing data. This is because I select which program name goes in the\nheader and filename. It also allows you to collect data in Stand Override, then\nseemlessly start collecting data to a new file in 24 Hour Rating."
        n230 = local read "Core HEWH Data DAQ LOOP"() -> (w525:T1)
        n231 = local read "User Controls DAQ LOOP"() -> (w523:T28)
        n232 = local read "POWER DAQ LOOP"() -> (w524:T12)
        n233 = Bundle By Name(cluster=w526, "Core HEWH Data DAQ LOOP"=w525, "POWER DAQ LOOP"=w524, "User Controls DAQ LOOP"=w523) -> (w522:T61)
        n234 = local read "Scan Rate Adjust"() -> (w520:T19)
        n235 = Bundle By Name(cluster=w522, "Core HEWH Data DAQ LOOP.Scan Rate Adjust"=w520) -> (w521:T61)
        n236 = call <vilib>:"Add State(s) to Queue__jki_lib_state_machine.vi"("State(s) in (\"\")"=w527) -> ("States Out"=w529:string)  [unwired: 14 in]
      }
      frame "Get Final Data" {
        n237 = Unbundle By Name(w532) -> ("Core HEWH Data DAQ LOOP"=→"Final Data Cluster":T1)
        n238 = call <vilib>:"Add State(s) to Queue__jki_lib_state_machine.vi"("State(s) in (\"\")"=w533) -> ("States Out"=w535:string)  [unwired: 14 in]
      }
    }
  }
  n239 = case shown="False" w34 {
    tunnel: w30 -> [w539 _]
    tunnel: [w538 errorcluster {"status"=FALSE, "code"=0, "source"=""} ("Error Out")] -> w38
    tunnel: [w537 refnum<file> refnum ("Refnum Out")] -> w37
    tunnel: w32 -> [w536 _]
    frame False {
      n240 = call "Open and Write CSV File.vi"("File Path Control"=w539, "Error In"=w536) -> ("Refnum Out"=w537:refnum<file>, "Error Out"=w538:errorcluster)  [unwired: 12 in]
    }
    frame True {
    }
  }
  n241 = call "UTILITY Boolean Notifier.vi"("Status"=UTILITY_Notifier."Set", "Set Status"=FALSE, "name (unnamed)"="Start UI Loop") -> ()  [unwired: 7 in, 2 out]
  n242 = call <vilib>:"Add State(s) to Queue__jki_lib_state_machine.vi"("State(s) in (\"\")"=w61) -> ("States Out"=w62:string)  [unwired: 14 in]
  n243 = call <vilib>:"Add State(s) to Queue__jki_lib_state_machine.vi"("State(s) in (\"\")"="Macro: Initialize") -> ("States Out"=w42:string)  [unwired: 14 in]
  n244 = call <vilib>:"Add State(s) to Queue__jki_lib_state_machine.vi"("State(s) in (\"\")"="Macro: Initialize") -> ("States Out"=w59:string)  [unwired: 14 in]
  n245 = call <vilib>:"Add State(s) to Queue__jki_lib_state_machine.vi"("State(s) in (\"\")"="Macro: Initialize") -> ("States Out"=w53:string)  [unwired: 14 in]
  n246 = while "Main Control Loop" {
    shift-right: [w549] -> _
    shift-left: _ -> [w548]
    shift-right: [w552] -> w60
    shift-left: w25 -> [w547]
    shift-right: [w551] -> _
    shift-left: w62 -> [w553]
    shift-right: [w544] -> _
    shift-left: string[] [] -> [w545]
    stop <- w550 stop-if-true
    # "Main Control Loop"
    n247 = call <vilib>:"Parse State Queue__jki_lib_state_machine.vi"("State Queue"=w553, "Error In (no error)"=w547) -> ("Remaining States"=w555:string, "Current State"=w543:string, "Arguments"=w554:string)  [unwired: 11 in]
    n248 = case shown="\"Dispense Schedule\"" w543 {
      selector: w543 -> [_ _ w625 _ _ _ _ _ _ _ _ _ _ _ _ _ _ _ _ _ _ _ _ _ _ _ _ _ _ _ _ _ _ _ _ _ _ _ _ _ _ _ _ _ _ _ _ _ _ _ _ _ _ _ _ _]
      tunnel: w555 -> [w566 w624 w629 w647 w653 w658 w662 w678 w693 w697 w708 w714 w725 w754 w769 w780 w799 w813 w821 w829 w851 w865 w876 w882 w898 w903 w908 w919 w921 w930 w937 w944 w951 w956 w963 w970 w978 w986 w991 w1003 w1036 w1054 w1072 w1078 w1097 w1112 w1122 w1136 w1152 w1161 w1167 w1181 w1195 w1234 w1238 w1256]
      tunnel: w554 -> [_ _ _ _ _ _ _ _ _ _ _ w709 w719 _ _ _ _ _ _ _ _ _ _ _ _ _ _ _ _ _ _ _ _ _ _ _ _ _ _ _ _ _ _ _ _ _ _ _ _ _ _ _ _ _ _ _]
      tunnel: w548 -> [w564 w621 w627 w638 w650 w656 w659 _ w689 w694 w698 w712 w721 w751 w767 w772 w796 w808 w817 w826 w833 w861 w871 w880 w897 w900 w905 w916 w922 w931 w938 w945 w952 w955 w960 w967 w977 w985 w988 w994 w1032 w1038 w1067 w1075 w1082 w1111 w1121 w1131 w1147 w1155 w1166 w1176 w1184 w1227 w1237 w1246]
      tunnel: [w563 w622 w631 w644 errorcluster {"status"=FALSE, "code"=0, "source"=""} ("error out") w655 w660 w676 w690 w695 w704 w710 w722 w752 w765 w778 w793 w809 w818 w827 w838 w858 w874 w877 w893 w901 w904 w917 w920 w925 w934 w941 w949 w954 w958 w965 w974 w982 w989 w1002 w1030 w1049 w1071 w1076 w1096 w1107 w1120 w1135 w1151 w1160 w1165 w1180 w1194 w1233 w1236 w1254] -> w552
      tunnel: w547 -> [w562 w622 w630 w644 w648 w655 w660 w676 w686 w695 w705 w711 w723 w752 w764 w777 w795 w810 w819 w828 w846 w854 w874 w879 w894 w901 w904 w917 w920 w926 w935 w942 w950 w954 w961 w968 w975 w983 w989 w1002 w1033 w1050 w1071 w1077 w1096 w1110 w1120 w1135 w1151 w1160 w1165 w1180 w1194 w1233 w1236 w1249]
      tunnel: [w565 w623 w628 w646 w652 w657 w661 w677 w692 w696 w707 w713 w724 w753 w768 w779 w798 w812 w820 w830 w850 w864 w875 w883 w899 w902 w907 w918 w923 w932 w939 w946 w953 w957 w964 w971 w979 w987 w990 w997 w1035 w1053 w1062 w1080 w1098 w1113 w1123 w1137 w1153 w1162 w1168 w1182 w1196 w1235 w1239 w1257] -> w551
      tunnel: [_ _ _ _ _ TRUE _ _ _ _ _ _ _ _ _ _ _ _ _ _ _ _ _ _ _ _ _ _ _ _ _ _ _ _ _ _ _ _ _ _ _ _ _ _ _ _ _ _ _ _ _ _ _ _ _ _] -> w550
      tunnel: [w561 w621 w627 w645 w650 w656 w659 w666 w689 w694 w698 w712 w721 w751 w757 w772 w797 w806 w816 w825 w833 w860 w870 w880 w897 w900 w905 w916 w922 w931 w938 w945 w952 w955 w960 w967 w977 w985 w988 w994 w1034 w1038 w1065 w1074 w1082 w1111 w1121 w1131 w1146 w1155 w1166 w1173 w1192 w1226 w1237 w1246] -> w549
      tunnel: 500 ("coerced(x)") -> [w560 _ _ _ _ _ _ _ _ _ _ _ _ _ _ _ _ _ _ _ _ _ _ _ _ _ _ _ _ _ _ _ _ _ _ _ _ _ _ _ _ _ _ _ _ _ _ _ _ _ _ _ _ _ _ _]
      frame "", "Idle" {
        n249 = event shown="[2] \"Reset Totalizer\": Value Change" {
          selector: _ -> [_ _ _ _ _ _ _ _]
          dyn-events: _ -> [_ _ _ _ _ _ _ _]
          timeout: w560 -> [_ _ _ _ _ _ _ _]
          tunnel: w566 -> [w572 w577 w584 w592 w599 w605 w614 w620]
          tunnel: [w567 w576 w583 w591 w598 w606 w614 w619] -> w565
          tunnel: w564 -> [w570 w580 w586 w589 w597 w603 w613 w617]
          tunnel: [w571 w581 w585 w593 w600 w607 w609 w618] -> w563
          tunnel: w562 -> [w571 w581 w585 w593 w600 w607 w610 w618]
          tunnel: [w570 w579 w586 w588 w596 w602 w613 w617] -> w561
          event Timeout {
            # "If the purge until condition is true or draw count is greater than\none (this is becasuse the draw increment is already\npassed by the time it sees the timeout loop.) \nGo ahead and update the test timer"
            n250 = event-data() -> ()  [unwired: 1 in, 1 out]
            n251 = local read "Start Draw Timer"() -> (w568:bool)
            n252 = case shown="True" w568 {
              tunnel: ["Check for UI Event\nGather Data\nUpdate Power Display\nCheck For Draw" ("State(s) in Front (\"\")") "Check for UI Event\nGather Data\nUpdate Power Display\nCheck For Draw\nDraw Time" ("State(s) in Front (\"\")")] -> w569
              frame False {
              }
              frame True {
              }
            }
            n253 = call <vilib>:"Add State(s) to Queue__jki_lib_state_machine.vi"("State(s) in Front (\"\")"=w569, "State(s) in (\"\")"=w572) -> ("States Out"=w567:string)  [unwired: 13 in]
          }
          event "HEWH Power": Value Change {
            n254 = event-data() -> ("NewVal"=w578:bool)  [unwired: 1 in, 5 out]
            n255 = call <vilib>:"Add State(s) to Queue__jki_lib_state_machine.vi"("State(s) in Front (\"\")"="Main Power" ("State(s) in Front (\"\")"), "State(s) in (\"\")"=w577) -> ("States Out"=w576:string)  [unwired: 13 in]
            n256 = Bundle By Name(cluster=w580, "User Controls.Main Power Control"=w578) -> (w579:T76)
          }
          event "Reset Totalizer": Value Change {
            n257 = event-data() -> ()  [unwired: 1 in, 6 out]
            n258 = call <vilib>:"Add State(s) to Queue__jki_lib_state_machine.vi"("State(s) in Front (\"\")"="Reset Totalizer" ("State(s) in Front (\"\")"), "State(s) in (\"\")"=w584) -> ("States Out"=w583:string)  [unwired: 13 in]
          }
          event "Flow Totalizer Control": Value Change {
            n259 = event-data() -> ("NewVal"=w587:bool)  [unwired: 1 in, 5 out]
            n260 = Bundle By Name(cluster=w589, "User Controls.Flow Totalizer Control"=w587) -> (w588:T76)
            n261 = call <vilib>:"Add State(s) to Queue__jki_lib_state_machine.vi"("State(s) in Front (\"\")"="Totalize Flow" ("State(s) in Front (\"\")"), "State(s) in (\"\")"=w592) -> ("States Out"=w591:string)  [unwired: 13 in]
          }
          event "Temperature": Value Change {
            n262 = event-data() -> ("NewVal"=w595:dbl)  [unwired: 1 in, 5 out]
            n263 = Bundle By Name(cluster=w597, "User Controls.Intellifaucet Temperature"=w595) -> (w596:T76)
            n264 = call <vilib>:"Add State(s) to Queue__jki_lib_state_machine.vi"("State(s) in Front (\"\")"="Adjust Temp" ("State(s) in Front (\"\")"), "State(s) in (\"\")"=w599) -> ("States Out"=w598:string)  [unwired: 13 in]
          }
          event "Valve % Open": Value Change {
            n265 = event-data() -> ("NewVal"=w601:dbl)  [unwired: 1 in, 5 out]
            n266 = Bundle By Name(cluster=w603, "User Controls.Percent Flow"=w601) -> (w602:T76)
            n267 = call <vilib>:"Add State(s) to Queue__jki_lib_state_machine.vi"("State(s) in Front (\"\")"="Adjust Flow" ("State(s) in Front (\"\")"), "State(s) in (\"\")"=w605) -> ("States Out"=w606:string)  [unwired: 13 in]
          }
          event "Pressurize Tank?": Value Change {
            n268 = event-data() -> ("NewVal"=w608:bool)  [unwired: 1 in, 5 out]
            n269 = call "UTILITY Boolean Notifier.vi"("Status"=UTILITY_Notifier."Set", "error in (no error)"=w610, "Set Status"=w608, "name (unnamed)"="Pressurize Tank?") -> ("error out"=w609:errorcluster)  [unwired: 6 in, 1 out]
          }
          event Panel Close? {
            # "Close Panel button (pressed) Event\n(this executes Macro: Exit to terminate the VI)"
            n270 = event-data() -> ()  [unwired: 1 in, 1 out]
            n271 = event-data("Discard?"=TRUE) -> ()  [unwired: 1 in, 1 out]
            n272 = call <vilib>:"Add State(s) to Queue__jki_lib_state_machine.vi"("State(s) in Front (\"\")"="Macro: Exit", "State(s) in (\"\")"=w620) -> ("States Out"=w619:string)  [unwired: 13 in]
          }
        }
      }
      frame "---------- Core ----------" {
        # "Do not put any code in this frame.\n(it is a separator no-op)"
        n273 = call <vilib>:"Add State(s) to Queue__jki_lib_state_machine.vi"("State(s) in (\"\")"=w624) -> ("States Out"=w623:string)  [unwired: 14 in]
      }
      frame Default {
        w634 = 42 items=["No error", "Argument error", "Memory is full", "Out of zone", "End of file", "File already open", "Generic file I/O error", "File not found", "File permission error", "Disk is full", "Duplicate path", "Too many files open", "System feature not enabled", "Resource file not found", "Cannot add resource", "Resource not found", "Image not found", "Image memory error", "Pen does not exist", "Config type invalid", "Config token not found", "Config parse error", "Config memory error", "Bad external code format", "Bad external code offset", "External code not present", "Null window", "Destroy window error", "Null menu", "Print aborted", "Bad print record", "Print driver error", "Windows error during printing", "Memory error during printing", "Print dialog error", "Generic print error", "Invalid device refnum", "Device not found", "Device parameter error", "Device unit error", "Cannot open device", "Device call aborted", "Generic error", "Cancelled by user", "Object ID too low", "Object ID too high", "Object not in heap", "Unknown heap", "Unknown object (invalid DefProc)", "Unknown object (DefProc not in table)", "Message out of range", "Invalid (null) method", "Unknown message", "Manager call not supported", "Bad address", "Network operation in progress", "Network operation timed out", "Connection is busy", "Network attribute not supported", "Network error", "Address in use", "System out of memory", "Connection aborted", "Connection refused", "Not connected", "Already connected", "Connection closed", "Initialization error (interapplication manager)", "Bad occurrence", "Wait on unbound occurrence handler", "Occurrence queue overflow", "Datalog type conflict", "Unused", "Unrecognized type (interapplication manager)", "Memory corrupt", "Failed to make temporary DLL", "Old CIN version", "Drag socket not found", "Failed to load drop-object", "Failed to register OLE object", "Failed to release OLE object", "Format specifier type mismatch", "Unknown format specifier", "Too few format specifiers", "Too many format specifiers", "Scan failed", "Newer CIN version", "Error converting to variant", "Runtime menu error", "Password tampered", "Variant attribute not found", "Incompatible variant data type", "Event data is not available", "Event Store is not present", "Occurrence is not found", "Event Queue is not created", "Event info is not available", "Refnum passed is NULL", "Error retrieving Class GUID", "Error retrieving CoClass GUID", "Error retrieving TypeLib GUID.", "Bad built application magic bytes.", "Specific driver is different from the specific driver associated with the Logical Name.", "There is no session opened to the class driver.", "Max Error", "MAX - Error with config objects", "MAX - Error loading configuration", "MAX - Group not supported"]
        # "Current State"
        # "Handle mistyped state name (developer tool)"
        n274 = Format Into String(format string="Software Exception: Unhandled State \"%s\"." ("message"), error in=w630, w625) -> (resulting string=w633:string, error out=w632:errorcluster)  [unwired: 1 in]
        n275 = call <vilib>:"Error Cluster From Error Code.vi"("show call chain? (False)"=TRUE, "error in (no error)"=w632, "error message (\"\")"=w633, "error code (0)"=w634) -> ("error out"=w631:errorcluster)  [unwired: 5 in]
        n276 = call <vilib>:"Add State(s) to Queue__jki_lib_state_machine.vi"("State(s) in (\"\")"=w629) -> ("States Out"=w628:string)  [unwired: 14 in]
      }
      frame "Initialize Core Data" {
        # "Do not delete, rename, or modify this frame.\n(this is used to determine panel behavior on exit)"
        # "If panel starts closed or is an EXE, then close it when we exit"
        n277 = property class="VI"() -> ("Front Panel.Open"=w643:bool)  [unwired: 2 in, 2 out]
        n278 = property class="App"() -> ("App.Kind"=w642:T68)  [unwired: 2 in, 2 out]
        n279 = control-ref of="Current VI Reference"() -> (w636:refnum<vi>)
        n280 = Not(x=w643) -> (.not. x?=w640:bool)
        n281 = Equal?(x=w642, y=T68."Run Time System" ("Application:Kind")) -> (x = y?=w639:bool)
        n282 = Or(x=w640, y=w639) -> (x .or. y?=w637:bool)
        n283 = Bundle By Name(cluster=w638, "Core.Current VI Reference"=w636, "Core.Close Panel on Exit?"=w637) -> (w645:T76)
        n284 = call <vilib>:"Add State(s) to Queue__jki_lib_state_machine.vi"("State(s) in (\"\")"=w647) -> ("States Out"=w646:string)  [unwired: 14 in]
      }
      frame "Error Handler" {
        # "The program is throwing an error after predraw..i think its a mw100 problem..\ngo back and fix"
        # "Unhandled Error -- Display it"
        # "Handle any errors here.\nYou can also output any states to clean-up after errors occur"
        # "Clear error"
        n285 = call <vilib>:"Clear Errors.vi"("error in (no error)"=w648) -> ()  [unwired: 5 in, 2 out]
        n286 = call <vilib>:"General Error Handler.vi"() -> ()  [unwired: 11 in, 5 out]
        n287 = call <vilib>:"Add State(s) to Queue__jki_lib_state_machine.vi"("State(s) in Front (\"\")"="/* Post Error States", "State(s) in (\"\")"=w653) -> ("States Out"=w652:string)  [unwired: 13 in]
      }
      frame "Exit" {
        # "Do not put any code in this frame.\n(No errors that occur here will be handled.)"
        n288 = call <vilib>:"Add State(s) to Queue__jki_lib_state_machine.vi"("State(s) in (\"\")"=w658) -> ("States Out"=w657:string)  [unwired: 14 in]
      }
      frame "---------- Data ----------" {
        # "Do not put any code in this frame.\n(It is a separator no-op. You can make a copy of this frame to create a new Data frame)"
        n289 = call <vilib>:"Add State(s) to Queue__jki_lib_state_machine.vi"("State(s) in (\"\")"=w662) -> ("States Out"=w661:string)  [unwired: 14 in]
      }
      frame "Data: Initialize" {
        w670 = string[][] []  # Save Data
        w671 = T28 {"Main Power Control"=FALSE, "Flow Totalizer Control"=FALSE, "Intellifaucet Temperature"=0.0, "Percent Flow"=0.0, "Safe Mode"=FALSE, "GEA2?"=FALSE, "Use Agilent?"=FALSE, "Valve Set A"=enum."Heating", "Valve Set B"=enum."Heating", "Valve Set C"=enum."Heating", "Valve Set D"=enum."Heating", "Valves"={"In VLV A"=enum."CLOSE", "Drain VLV A"=enum."OPEN", "Out VLV A"=enum."OPEN", "In VLV B"=enum."OPEN", "Drain VLV B"=enum."OPEN", "Out VLV B"=enum."OPEN", "In VLV C"=enum."CLOSE", "Drain VLV C"=enum."OPEN", "Out VLV C"=enum."OPEN", "In VLV D"=enum."CLOSE", "Drain VLV D"=enum."OPEN", "Out VLV D"=enum."OPEN"}}  # User Controls
        w673 = T73 {"Scan Rate Adjust"=0.0, "Draw Count"=0, "Test Patten Setup"={"Total Gallons Schedule"=[], "PRAT/RLT Sequence"=[{"Sequence #"=1.0, "Cycles"=35, "Mode Setting"="", "Flow Rate (GPM)"=0.0, "Temperature (F)"=0.0, "Reset Timer"=FALSE, "Use Temp Decline Method"=FALSE, "Terminate Condition"=enum."C1-Terminate Draw @ Gallon Mark", "Condition Value #1"=1.0, "UE"=FALSE, "LE"=FALSE, "Comp"=FALSE, "Fan"=FALSE, "Test End Time (Sec)"=0.0, "Purge Until Cutout"=FALSE, "Start Conditions"=enum."Heat Source Cutout", "Condition Value #2"=0.0, "Remove Power"=FALSE, "Time"=0.0, "Check Special Cond."=enum."SC1-Do Nothing", "Condition#"=enum."C1", "Draw Flags"=enum."N/A", "Data Processing Delay (FHD 15sec, UEF 5 Sec)"=0.0, "Test Complete"=FALSE}, {"Sequence #"=2.0, "Cycles"=15, "Mode Setting"="", "Flow Rate (GPM)"=0.0, "Temperature (F)"=0.0, "Reset Timer"=FALSE, "Use Temp Decline Method"=FALSE, "Terminate Condition"=enum."C1-Terminate Draw @ Gallon Mark", "Condition Value #1"=1.0, "UE"=FALSE, "LE"=FALSE, "Comp"=FALSE, "Fan"=FALSE, "Test End Time (Sec)"=0.0, "Purge Until Cutout"=FALSE, "Start Conditions"=enum."Heat Source Cutout", "Condition Value #2"=0.0, "Remove Power"=FALSE, "Time"=0.0, "Check Special Cond."=enum."SC1-Do Nothing", "Condition#"=enum."C1", "Draw Flags"=enum."N/A", "Data Processing Delay (FHD 15sec, UEF 5 Sec)"=0.0, "Test Complete"=FALSE}, {"Sequence #"=3.0, "Cycles"=35, "Mode Setting"="", "Flow Rate (GPM)"=0.0, "Temperature (F)"=0.0, "Reset Timer"=FALSE, "Use Temp Decline Method"=FALSE, "Terminate Condition"=enum."C1-Terminate Draw @ Gallon Mark", "Condition Value #1"=2.0, "UE"=FALSE, "LE"=FALSE, "Comp"=FALSE, "Fan"=FALSE, "Test End Time (Sec)"=0.0, "Purge Until Cutout"=FALSE, "Start Conditions"=enum."Heat Source Cutout", "Condition Value #2"=0.0, "Remove Power"=FALSE, "Time"=0.0, "Check Special Cond."=enum."SC1-Do Nothing", "Condition#"=enum."C1", "Draw Flags"=enum."N/A", "Data Processing Delay (FHD 15sec, UEF 5 Sec)"=0.0, "Test Complete"=FALSE}, {"Sequence #"=4.0, "Cycles"=15, "Mode Setting"="", "Flow Rate (GPM)"=0.0, "Temperature (F)"=0.0, "Reset Timer"=FALSE, "Use Temp Decline Method"=FALSE, "Terminate Condition"=enum."C1-Terminate Draw @ Gallon Mark", "Condition Value #1"=2.0, "UE"=FALSE, "LE"=FALSE, "Comp"=FALSE, "Fan"=FALSE, "Test End Time (Sec)"=0.0, "Purge Until Cutout"=FALSE, "Start Conditions"=enum."Heat Source Cutout", "Condition Value #2"=0.0, "Remove Power"=FALSE, "Time"=0.0, "Check Special Cond."=enum."SC1-Do Nothing", "Condition#"=enum."C1", "Draw Flags"=enum."N/A", "Data Processing Delay (FHD 15sec, UEF 5 Sec)"=0.0, "Test Complete"=FALSE}, {"Sequence #"=5.0, "Cycles"=35, "Mode Setting"="", "Flow Rate (GPM)"=0.0, "Temperature (F)"=0.0, "Reset Timer"=FALSE, "Use Temp Decline Method"=FALSE, "Terminate Condition"=enum."C1-Terminate Draw @ Gallon Mark", "Condition Value #1"=0.0, "UE"=FALSE, "LE"=FALSE, "Comp"=FALSE, "Fan"=FALSE, "Test End Time (Sec)"=0.0, "Purge Until Cutout"=FALSE, "Start Conditions"=enum."Heat Source Cutout", "Condition Value #2"=0.0, "Remove Power"=FALSE, "Time"=0.0, "Check Special Cond."=enum."SC1-Do Nothing", "Condition#"=enum."C1", "Draw Flags"=enum."N/A", "Data Processing Delay (FHD 15sec, UEF 5 Sec)"=0.0, "Test Complete"=FALSE}, {"Sequence #"=6.0, "Cycles"=15, "Mode Setting"="", "Flow Rate (GPM)"=0.0, "Temperature (F)"=0.0, "Reset Timer"=FALSE, "Use Temp Decline Method"=FALSE, "Terminate Condition"=enum."C1-Terminate Draw @ Gallon Mark", "Condition Value #1"=0.0, "UE"=FALSE, "LE"=FALSE, "Comp"=FALSE, "Fan"=FALSE, "Test End Time (Sec)"=0.0, "Purge Until Cutout"=FALSE, "Start Conditions"=enum."Heat Source Cutout", "Condition Value #2"=0.0, "Remove Power"=FALSE, "Time"=0.0, "Check Special Cond."=enum."SC1-Do Nothing", "Condition#"=enum."C1", "Draw Flags"=enum."N/A", "Data Processing Delay (FHD 15sec, UEF 5 Sec)"=0.0, "Test Complete"=FALSE}, {"Sequence #"=7.0, "Cycles"=35, "Mode Setting"="", "Flow Rate (GPM)"=0.0, "Temperature (F)"=0.0, "Reset Timer"=FALSE, "Use Temp Decline Method"=FALSE, "Terminate Condition"=enum."C1-Terminate Draw @ Gallon Mark", "Condition Value #1"=1.0, "UE"=FALSE, "LE"=FALSE, "Comp"=FALSE, "Fan"=FALSE, "Test End Time (Sec)"=0.0, "Purge Until Cutout"=FALSE, "Start Conditions"=enum."Heat Source Cutout", "Condition Value #2"=0.0, "Remove Power"=FALSE, "Time"=0.0, "Check Special Cond."=enum."SC1-Do Nothing", "Condition#"=enum."C1", "Draw Flags"=enum."N/A", "Data Processing Delay (FHD 15sec, UEF 5 Sec)"=0.0, "Test Complete"=FALSE}, {"Sequence #"=8.0, "Cycles"=15, "Mode Setting"="", "Flow Rate (GPM)"=0.0, "Temperature (F)"=0.0, "Reset Timer"=FALSE, "Use Temp Decline Method"=FALSE, "Terminate Condition"=enum."C1-Terminate Draw @ Gallon Mark", "Condition Value #1"=1.0, "UE"=FALSE, "LE"=FALSE, "Comp"=FALSE, "Fan"=FALSE, "Test End Time (Sec)"=0.0, "Purge Until Cutout"=FALSE, "Start Conditions"=enum."Heat Source Cutout", "Condition Value #2"=0.0, "Remove Power"=FALSE, "Time"=0.0, "Check Special Cond."=enum."SC1-Do Nothing", "Condition#"=enum."C1", "Draw Flags"=enum."N/A", "Data Processing Delay (FHD 15sec, UEF 5 Sec)"=0.0, "Test Complete"=FALSE}], "Current Sequence Index"=0}, "Condition Cluster Output"={"Condition #1"=FALSE, "Condition #2"=FALSE, "Special Last Draw (HU Test)"=FALSE, "RTD Out Temperature <="=0.0, "Condition #3"=FALSE, "Mean Tank Temperature <="=0.0, "Condition #4"=FALSE, "Decrease Outlet Temperature \nBy (RTD Out)"=0.0, "Condition #5"=FALSE, "Condition #6"=FALSE, "Time (Seconds)"=0.0, "Condition #7"=FALSE, "Condition #8"=FALSE, "Draw Until Condition"={"UE"=FALSE, "LE"=FALSE, "COMP"=FALSE, "FANS"=FALSE}, "Condition #9"=FALSE}, "HEWH Specific DAQ"={"HEWH Data"={"HEWH Standard"={"Voltage (Volts)"=0.0, "Current (Amps)"=0.0, "Power (Watts)"=0.0, "WattHours (Wh)"=0.0, "TC Tree (AVG)"=0.0, "Flow Rate (GPM)"=0.0, "Gallons (Gal)"=0.0, "RTD Out (Deg F)"=0.0, "RTD In (Deg F)"=0.0, "RTD Amb (Deg F)"=0.0, "TC Down"=0.0, "UE Event Lead"=0, "LE Event Lead"=0, "TC Tree Array"=[]}, "PRAT"={"Power (Watts) A"=4192.0, "Power (Watts) B"=4192.0, "Power (Watts) C"=4192.0, "Power (Watts) D"=4192.0, "TC1"=0.0, "TC2"=0.0, "TC3"=0.0, "TC4"=0.0, "WattHours (Wh) A"=4192.0, "WattHours (Wh) B"=4192.0, "WattHours (Wh) C"=4192.0, "WattHours (Wh) D"=4192.0, "Ambient"=0.0, "Extra Temp"=0.0}, "Additional Power Data"={"Vthd"=236.2, "Frequency (Hz)"=236.2, "Apparent Power (VA)"=236.2, "Power Factor"=236.2, "Current Crest Factor"=236.2, "Voltage Crest Factor"=236.2, "Integration Time (sec)"=236.2}}, "Intellif Valve % Open"=0.0, "Power State"={"UE"=FALSE, "LE"=FALSE, "COMP"=FALSE, "FANS"=FALSE}, "Power Analyzer"=enum."", "Intellifaucet Configuration"=enum."DRK500,Station1"}, "Test Output Data"={"PreDraw Data Table"=[], "Data Table"=[], "MW100 TC Headers"=[]}, "Calc and Calibration"={"RTD Max Min Array"=[], "Draw Statistics"=[], "Calibration Coefficients DBL"=[], "Min RTD Temp\nDuring Draw"=0.0, "Start Gallons"=0.0, "Starting Temp Decline A"=0.0, "Max RTD Temp\nDuring Draw"=0.0, "Draw Start Time"=0.0, "Delay Start Time"=0.0, "Current Purge Start Time"=0.0, "K-Factor (Intellifaucet)"=0.0, "Starting Temp Decline B"=0.0, "Starting Temp Decline C"=0.0, "Starting Temp Decline D"=0.0}, "Current Draw Time"=0.0, "LV Program"=enum."HEWH", "Station ID"=enum."A"}  # Core HEWH Data
        w675 = T77 {"Current VI Reference"=refnum, "Close Panel on Exit?"=FALSE}  # Core
        n290 = local write "Tab Control 3"(T32."Main" ("Tab Control 3")) -> ()
        n291 = local write "Message"(T23 "Select Test...." ("Message")) -> ()
        n292 = Bundle("Core"=w675, "Data File Directory"="Data File Directory", "Core HEWH Data"=w673, "Equipment VISA"="Equipment VISA", "User Controls"=w671, "Save Data"=w670, "Filepath"="Filepath", "LV Program"="LV Program", "Washer Controls"="Washer Controls") -> (w666:T76)  [unwired: 1 in]
        n293 = call <vilib>:"Add State(s) to Queue__jki_lib_state_machine.vi"("State(s) in (\"\")"=w678) -> ("States Out"=w677:string)  [unwired: 14 in]
        "Description" <- "Main 2"
      }
      frame "Data: Cleanup" {
        w683 = u16 0 items=["A", "B", "C", "D"] ("Valve Bank")
        n294 = Unbundle By Name(w689) -> ("Core.Current VI Reference"=w691:refnum<vi>, "Washer Controls.Test Fixture Hardware"=w688:T43, "Washer Controls.Test Fixture Hardware.Analog Data.Yokogawa.MW100"=w682:refnum<visa-resource-name>)
        n295 = local read "Pressurize Tank?"() -> (w680:bool)
        n296 = call "HEWH Set Valves.vi"("VISA session"=w682, "Station ID"=w683, "Pressurize Tank?"=w680, "Valve Bank Setting"=HEWH_Valve_Bank_Positions."Resting", "Stop Intellifaucet?"=TRUE, "Error In"=w686, "Start Intellifaucet?"=FALSE) -> ("Error Out"=w685:errorcluster)  [unwired: 7 in, 1 out]
        n297 = call "HEWH Close Equipmet.vi"("Error In"=w685, "Test Fixture Hardware In"=w688) -> ("Error Out"=w687:errorcluster)  [unwired: 8 in, 1 out]
        n298 = Close Reference(reference=w691, error in (no error)=w687) -> (error out=w690:errorcluster)
        n299 = call <vilib>:"Add State(s) to Queue__jki_lib_state_machine.vi"("State(s) in (\"\")"=w693) -> ("States Out"=w692:string)  [unwired: 14 in]
      }
      frame "---------- Setup ----------" {
        n300 = call <vilib>:"Add State(s) to Queue__jki_lib_state_machine.vi"("State(s) in (\"\")"=w697) -> ("States Out"=w696:string)  [unwired: 14 in]
      }
      frame "UI: Initialize" {
        w701 = 0.0 ("Percent Flow")
        w702 = 58.0 ("Temperature(F)")
        n301 = Current VI's Path() -> (path=w706:path)
        n302 = call "UTILITY This VIs Path.vi"("path"=w706, "error in (no error)"=w705) -> ("FileVersionInfo Out"=w700:T52, "error out"=w704:errorcluster)  [unwired: 7 in, 5 out]
        n303 = Unbundle By Name(w700) -> ("FileVersion"=→"Description 4":string)
        n304 = property on="Temperature" class="Slide (strict)"("Val(Sgnl)"=w702) -> ()  [unwired: 2 in, 2 out]
        n305 = local write "Temperature"(w702) -> ()
        n306 = property on="Valve % Open" class="Slide (strict)"("Val(Sgnl)"=w701) -> ()  [unwired: 2 in, 2 out]
        n307 = local write "Valve % Open"(w701) -> ()
        n308 = call <vilib>:"Add State(s) to Queue__jki_lib_state_machine.vi"("State(s) in (\"\")"=w708) -> ("States Out"=w707:string)  [unwired: 14 in]
        "Tank Display" <- T26 {"TC1"=0.0, "TC2"=0.0, "TC3"=0.0, "TC4"=0.0, "TC5"=0.0, "TIN"=0.0, "TOUT"=0.0, "TC6"=0.0, "TC6-Color"=0, "TC5-Color"=0, "TC4-Color"=0, "TC3-Color"=0, "TC2-Color"=0, "TC1-Color"=0, "RTD-Out"=0, "RTD-In"=0} ("Tank Display")
      }
      frame "UI: Cursor Set" {
        # "Argument"
        n309 = case shown="\"Idle\", Default" w709 {
          tunnel: w711 -> [w716 w718]
          tunnel: [w715 w717] -> w710
          frame "Idle", Default {
            n310 = call <vilib>:"Unset Busy.vi"("error in (no error)"=w716) -> ("error out"=w715:errorcluster)  [unwired: 10 in]
          }
          frame "Busy" {
            n311 = call <vilib>:"Set Busy.vi"("error in (no error)"=w718) -> ("error out"=w717:errorcluster)  [unwired: 9 in, 1 out]
          }
        }
        n312 = call <vilib>:"Add State(s) to Queue__jki_lib_state_machine.vi"("State(s) in (\"\")"=w714) -> ("States Out"=w713:string)  [unwired: 14 in]
      }
      frame "UI: Front Panel State" {
        # "Argument"
        n313 = Unbundle By Name(w721) -> ("Core.Current VI Reference"=w720:refnum<vi>)
        n314 = case shown="\"Close\"" w719 {
          tunnel: w723 -> [w729 w742]
          tunnel: [w731 w743] -> w722
          tunnel: w720 -> [w730 w740]
          frame "Open", Default {
            n315 = property class="VI"(reference=w730, error in=w729) -> (reference out=w727:refnum<vi>, error out=w728:errorcluster, "Front Panel.Open"=w726:bool)
            n316 = case shown="False" w726 {
              tunnel: [w734 w737] -> w731
              tunnel: w728 -> [w733 w737]
              tunnel: w727 -> [w732 _]
              frame False {
                n317 = invoke class="VI" method="FP.Open"(reference=w732, error in=w733, "Activate"=TRUE, "State"=T70."Standard") -> (error out=w734:errorcluster)  [unwired: 1 in, 4 out]
              }
              frame True {
              }
            }
          }
          frame "Close" {
            n318 = property class="VI"(reference=w740, error in=w742) -> (reference out=w739:refnum<vi>, error out=w741:errorcluster, "Front Panel.Open"=w738:bool)
            n319 = case shown="False" w738 {
              tunnel: [w744 w749] -> w743
              tunnel: w741 -> [w744 w748]
              tunnel: w739 -> [_ w747]
              frame False {
              }
              frame True {
                n320 = invoke class="VI" method="FP.Open"(reference=w747, error in=w748, "Activate"=FALSE ("Activate?"), "State"=T70."Standard") -> (error out=w749:errorcluster)  [unwired: 1 in, 4 out]
              }
            }
          }
        }
        n321 = call <vilib>:"Add State(s) to Queue__jki_lib_state_machine.vi"("State(s) in (\"\")"=w725) -> ("States Out"=w724:string)  [unwired: 14 in]
      }
      frame "Start DAQ Write" {
        n322 = call <vilib>:"Add State(s) to Queue__jki_lib_state_machine.vi"("State(s) in (\"\")"=w754) -> ("States Out"=w753:string)  [unwired: 14 in]
        "Start DAQ Write" <- TRUE ("Start DAQ Write")
      }
      frame "File Setup" {
        # "Setup file name and initialization array"
        n323 = Unbundle By Name(w767) -> ("Filepath"=w761:T41, "LV Program"=w760:T17)
        n324 = call "Save File DOE File Setup.vi"("Filepath In"=w761, 1:w760, "error in (no error)"=w764, "Config State"=Save_File_DOE_Configuration_State."Open Front Panel") -> ("Washer Controls Out"=w759:T78, "Filepath Out"=w758:T82, "error out"=w763:errorcluster)  [unwired: 13 in]
        n325 = Bundle By Name(cluster=w767, "Washer Controls"=w759, "Filepath"=w758) -> (w757:T76)
        n326 = Unbundle By Name(w757) -> ("Core HEWH Data"=w766:T73, "User Controls"=w756:T28, "Core HEWH Data.HEWH Specific DAQ.Power State"=w755:T12)
        n327 = flat-sequence {
          tunnel: w763 -> [w771]
          tunnel: [w771] -> w765
          frame #0 {
            n328 = local write "Shutdown DAQ"("Update FileInit Cluster") -> ()
          }
        }
        n329 = local write "Core HEWH Data DAQ LOOP"(w766) -> ()
        n330 = local write "User Controls DAQ LOOP"(w756) -> ()
        n331 = local write "POWER DAQ LOOP"(w755) -> ()
        n332 = call <vilib>:"Add State(s) to Queue__jki_lib_state_machine.vi"("State(s) in (\"\")"=w769) -> ("States Out"=w768:string)  [unwired: 14 in]
      }
      frame "Start UI Loop" {
        # "Pass Startup Data to other SM's"
        n333 = local read "HEWH Power"() -> (w773:bool)
        n334 = Unbundle By Name(w772) -> ("User Controls"=→"User Controls DAQ LOOP":T28, "Core HEWH Data.HEWH Specific DAQ.Power State"=→"POWER DAQ LOOP":T12, "Core HEWH Data"=→"Core HEWH Data DAQ LOOP":T73)
        n335 = property on="HEWH Power" class="Bool (strict)"("Val(Sgnl)"=w773) -> ()  [unwired: 2 in, 2 out]
        n336 = flat-sequence {
          tunnel: w777 -> [w783]
          tunnel: [w782] -> w778
          frame #0 {
            n337 = call "UTILITY Boolean Notifier.vi"("Status"=UTILITY_Notifier."Set", "error in (no error)"=w783, "Set Status"=TRUE, "name (unnamed)"="Start UI Loop") -> ("error out"=w782:errorcluster)  [unwired: 6 in, 1 out]
          }
        }
        n338 = call <vilib>:"Add State(s) to Queue__jki_lib_state_machine.vi"("State(s) in (\"\")"=w780) -> ("States Out"=w779:string)  [unwired: 14 in]
      }
      frame "Init Communication" {
        # "For some reason the initial\nscan rate does not take from \nthe type def"
        # "Does this unit have GEA2?"
        n339 = call "HEWH Read Settings.vi"() -> ("Station"=→"Station":string, "Power Analyzer"=w790:string, "Intellifaucet Type"=w792:string)  [unwired: 6 in, 3 out]
        "Intellifaucet Type" <- w792
        n340 = call "HEWH Panel Communication Settings.vi"("error in (no error)"=w795) -> ("GEA2 HyperData Out"=w794:bool, "error out"=w793:errorcluster)  [unwired: 13 in]
        "Trigger With GEA2" <- w794
        n341 = case shown="\"WT300\"" w790 {
          tunnel: [UTILITY_Power_Analyzer."OSI" ("Power Analyzer") UTILITY_Power_Analyzer."WT210" ("Power Analyzer") UTILITY_Power_Analyzer."WT300" ("Power Analyzer")] -> w788
          frame "OSI", Default {
          }
          frame "WT210" {
          }
          frame "WT300" {
          }
        }
        n342 = case shown="\"DRK250\"" w792 {
          tunnel: [INTELLIFAUCET_Tested_Flowrate_Scenarios."DRK500,Station1" ("Configuration") INTELLIFAUCET_Tested_Flowrate_Scenarios."DRK500,Station1" ("Configuration") INTELLIFAUCET_Tested_Flowrate_Scenarios."DRK500,Station1" ("Configuration")] -> w787
          frame "DRK375", Default {
          }
          frame "DRK250" {
          }
          frame "DRK500" {
          }
        }
        n343 = Bundle By Name(cluster=w796, "Core HEWH Data.Scan Rate Adjust"=1000.0 ("FileInit Cluster.Scan Rate Adjust"), "User Controls.GEA2?"=w794, "Core HEWH Data.HEWH Specific DAQ.Power Analyzer"=w788, "Core HEWH Data.HEWH Specific DAQ.Intellifaucet Configuration"=w787, "LV Program"=Save_File_DOE_LabView_Program."HEWH") -> (w797:T76)
        n344 = call <vilib>:"Add State(s) to Queue__jki_lib_state_machine.vi"("State(s) in (\"\")"=w799) -> ("States Out"=w798:string)  [unwired: 14 in]
      }
      frame "Check for Calibration File" {
        n345 = Unbundle By Name(w808) -> ("Filepath.General Setup Paths.Calibration File Path"=w811:path)
        n346 = call "HEWH Calibration File Check.vi"("error in (no error)"=w810, "Calibration Path"=w811) -> ("error out"=w809:errorcluster, "Calibration File Array"=w807:dbl[][])  [unwired: 6 in, 2 out]
        n347 = Bundle By Name(cluster=w808, "Core HEWH Data.Calc and Calibration.Calibration Coefficients DBL"=w807) -> (w806:T76)
        n348 = call <vilib>:"Add State(s) to Queue__jki_lib_state_machine.vi"("State(s) in (\"\")"=w813) -> ("States Out"=w812:string)  [unwired: 14 in]
      }
      frame "Dispense Schedule" {
        n349 = call "HEWH Dispense Schedule.vi"("Core HEWH Data Input"=TRUE ("Hide PreDraw Tab"), "error in (no error)"=w819) -> ("Core HEWH Data Input Out"=w815:T83, "error out"=w818:errorcluster)  [unwired: 12 in]
        n350 = Bundle By Name(cluster=w817, "Core HEWH Data.Test Patten Setup"=w815) -> (w816:T76)
        n351 = call <vilib>:"Add State(s) to Queue__jki_lib_state_machine.vi"("State(s) in (\"\")"=w821) -> ("States Out"=w820:string)  [unwired: 14 in]
      }
      frame "Draw Until" {
        n352 = call "HEWH Draw Until.vi"("error in (no error)"=w828) -> ("error out"=w827:errorcluster, "Condition Cluster Output"=w823:T11)  [unwired: 8 in]
        n353 = Bundle By Name(cluster=w826, "Core HEWH Data.Condition Cluster Output"=w823) -> (w825:T76)
        n354 = Unbundle By Name(w823) -> ("Return Output Bool"=w822:bool)
        n355 = case shown="False" w822 {
          tunnel: ["Dispense Gallons" ("State(s) in Front (\"\")") ""] -> w824
          frame False {
          }
          frame True {
          }
        }
        n356 = call <vilib>:"Add State(s) to Queue__jki_lib_state_machine.vi"("State(s) in Front (\"\")"=w824, "State(s) in (\"\")"=w829) -> ("States Out"=w830:string)  [unwired: 13 in]
      }
      frame "Set Valve Bank 1" {
        w835 = TRUE
        w840 = u16 0 items=["A", "B", "C", "D"] ("Valve Bank")
        w849 = T85 30 items=["4-20_OUT", "Pres_HI1", "Pres_HI2", "Pres_LOW", "Pres_PIN", "HEATER_TOP", "HEATER_BOT", "T_Shell", "FLOWMETER", "WATT_SENSE", "WH_TICK", "Tc_1", "Tc_2", "Tc_3", "Tc_4", "Tc_5", "Tc_6", "Tc_down", "T_Shell_2", "T_Shell_3", "T_Shell_4", "RTD_IN", "RTD_OUT", "RTD_AMB", "INTF_TEMPFLO", "INTF_READY", "INTF_START", "INTF_STOP", "DRM_LOW", "DRM_HIGH", "PWR_MAIN", "VLV_DUMP", "VLV_OUT", "VLV_IN", "WATT_HOURS", "FLOW(SAMPLE)", "GALLONS", "FLOW(GPM)"] ("Channel_Enum")
        n357 = Unbundle By Name(w833) -> ("Equipment VISA.MW100"=w837:refnum<visa-resource-name>)
        n358 = property on="Inlet Valve A" class="Enum (strict)"("Visible"=w835) -> ()  [unwired: 2 in, 2 out]
        n359 = property on="Drain Valve A" class="Enum (strict)"("Visible"=w835) -> ()  [unwired: 2 in, 2 out]
        n360 = property on="Outlet Valve A" class="Enum (strict)"("Visible"=w835) -> ()  [unwired: 2 in, 2 out]
        n361 = call "YKMW100 VF0 Relay Status.vi"("VISA session"=w837, 5:w849, "Error In"=w846) -> ("dup VISA session"=w834:refnum<visa-resource-name>, "Control Relay ON (Supplying Power to Unit)"=w847:bool, "error out"=w839:errorcluster)  [unwired: 8 in, 2 out]
        n362 = Not(x=w847) -> (.not. x?=w848:bool)
        n363 = local write "HEWH Power"(w848) -> ()
        n364 = local write "Message"(T23 "Initializing...." ("Message")) -> ()
        n365 = local read "Pressurize Tank?"() -> (w842:bool)
        n366 = call "HEWH Set Valves.vi"("VISA session"=w834, "Station ID"=w840, "Pressurize Tank?"=w842, "Valve Bank Setting"=HEWH_Valve_Bank_Positions."Heating", "Stop Intellifaucet?"=TRUE, "Error In"=w839, "Start Intellifaucet?"=FALSE) -> ("Error Out"=w838:errorcluster)  [unwired: 7 in, 1 out]
        n367 = call <vilib>:"Add State(s) to Queue__jki_lib_state_machine.vi"("State(s) in Front (\"\")"="", "State(s) in (\"\")"=w851) -> ("States Out"=w850:string)  [unwired: 13 in]
      }
      frame "Initialize Equipment" {
        # "Give it a second to make sure\neverything is setup."
        n368 = Unbundle By Name(w861) -> ("User Controls.Use Agilent?"=w856:bool, "Washer Controls.Test Fixture Hardware"=w863:T43, "Core HEWH Data"=w862:T73)
        n369 = call "HEWH_Power ON.vi"("error in (no error)"=w854) -> ("error out"=w853:errorcluster, "ON or OFF"=w852:bool)  [unwired: 9 in]
        n370 = local write "Message"(T23 "Initializing...." ("Message")) -> ()
        n371 = call "HEWH Initialize Equipmet.vi"("Use Agilent?"=w856, "Error In"=w853, "Core HEWH Data"=w862, "Test Fixture Hardware"=w863) -> ("Error Out"=w859:errorcluster)  [unwired: 6 in, 1 out]
        n372 = call "UTILITY Delay mS.vi"("Error In"=w859, "milliseconds to wait"=u32 1000) -> ("Error Out"=w858:errorcluster)  [unwired: 13 in]
        n373 = Bundle By Name(cluster=w861, "User Controls.Main Power Control"=w852) -> (w860:T76)
        n374 = local write "HEWH Power"(w852) -> ()
        n375 = call <vilib>:"Add State(s) to Queue__jki_lib_state_machine.vi"("State(s) in (\"\")"=w865) -> ("States Out"=w864:string)  [unwired: 14 in]
      }
      frame "Get Agilent Scan List" {
        n376 = call "HEWH Channel Test Labels.vi"("RunTime"=FALSE) -> ("MW100 Channel Label"=w866:string[], "Agilent Cluster Array"=w867:T46[], "Channel List"=w869:string)  [unwired: 12 in]
        n377 = String Length(string=w869) -> (length=w873:i32)
        n378 = Greater Than 0?(x=w873) -> (x > 0?=w868:bool)
        "Use Agilent?" <- w868
        n379 = Bundle By Name(cluster=w871, "Core HEWH Data.Test Output Data.MW100 TC Headers"=w866, "Washer Controls.Test Fixture Hardware.Analog Data.Agilent.Agilent Cluster Array"=w867, "Washer Controls.Test Fixture Hardware.Analog Data.Agilent.TC Channels-List"=w869, "User Controls.Use Agilent?"=w868) -> (w870:T76)
        n380 = call <vilib>:"Add State(s) to Queue__jki_lib_state_machine.vi"("State(s) in (\"\")"=w876) -> ("States Out"=w875:string)  [unwired: 14 in]
      }
      frame "Reset Totalizer" {
        n381 = Unbundle By Name(w880) -> ("Washer Controls.Test Fixture Hardware"=w881:T43, "Core HEWH Data.HEWH Specific DAQ.Power Analyzer"=w878:T14)
        n382 = case shown="\"APLUS\", Default" w878 {
          tunnel: w881 -> [w887 w892]
          tunnel: w879 -> [w886 w890]
          tunnel: [w885 w889] -> w877
          frame "APLUS", Default {
            n383 = Unbundle By Name(w887) -> ("Analog Data.Yokogawa.MW100"=w884:refnum<visa-resource-name>)
            n384 = call "HEWH Reset MW100.vi"("error in (no error)"=w886, "MW100 VISA In"=w884) -> ("error out"=w885:errorcluster)  [unwired: 8 in, 1 out]
          }
          frame "WT300" {
            n385 = Unbundle By Name(w892) -> ("Power.Yokogawa.WT210.Power VISA Yokogawa WT210"=w891:refnum<visa-resource-name>, "Analog Data.Yokogawa.MW100"=w888:refnum<visa-resource-name>)
            n386 = call "HEWH Reset MW100.vi"("error in (no error)"=w890, "MW100 VISA In"=w888) -> ("error out"=w889:errorcluster)  [unwired: 8 in, 1 out]
            n387 = call "Yokogawa WT300 Series Reset Integrator.vi"("VISA Refnum in"=w891) -> ()  [unwired: 9 in, 2 out]
          }
        }
        n388 = call <vilib>:"Add State(s) to Queue__jki_lib_state_machine.vi"("State(s) in (\"\")"=w882) -> ("States Out"=w883:string)  [unwired: 14 in]
      }
      frame "Totalize Flow" {
        n389 = Unbundle By Name(w897) -> ("Washer Controls.Test Fixture Hardware.Analog Data.Yokogawa.MW100"=w896:refnum<visa-resource-name>, "User Controls.Flow Totalizer Control"=w895:bool)
        n390 = call "HEWH Totalize Flow Control.vi"("VISA session"=w896, "Totalize Flow"=w895, "error in (no error)"=w894) -> ("error out"=w893:errorcluster)  [unwired: 11 in, 1 out]
        n391 = call <vilib>:"Add State(s) to Queue__jki_lib_state_machine.vi"("State(s) in (\"\")"=w898) -> ("States Out"=w899:string)  [unwired: 14 in]
      }
      frame "---------- Macro ----------" {
        n392 = call <vilib>:"Add State(s) to Queue__jki_lib_state_machine.vi"("State(s) in (\"\")"=w903) -> ("States Out"=w902:string)  [unwired: 14 in]
      }
      frame "Macro: Initialize" {
        w906 = "Data: Initialize\nInit Communication\nCheck for Calibration File\nGet Agilent Scan List\nSet Valve Bank 1\nInitialize Equipment\nTerm Purge\nTerm Draw\nReset Totalizer\nMain Power\nStart UI Loop\nInitialize Core Data\nUI: Initialize\nUI: Front Panel State >> Open"  # Data: Initialize Init Communication Check for Calibration File Get Agilent Scan List Set Valve Bank 1 Initialize Equipment Term Purge Term Draw Reset Totalizer Main Power Start UI Loop Initialize Core Data UI: Initialize UI: Front Panel State >> Open
        n393 = call <vilib>:"Add State(s) to Queue__jki_lib_state_machine.vi"("State(s) in Front (\"\")"=w906, "State(s) in (\"\")"=w908) -> ("States Out"=w907:string)  [unwired: 13 in]
      }
      frame "Macro: Exit" {
        n394 = Unbundle By Name(w916) -> ("Core.Close Panel on Exit?"=w915:bool)
        n395 = local write "Start DAQ Write"(FALSE ("Start DAQ Write")) -> ()
        n396 = Select(t="UI: Front Panel State >> Close", s=w915, f="") -> (s? t:f=w912:string)
        n397 = call <vilib>:"Add State(s) to Queue__jki_lib_state_machine.vi"("State(s) in (\"\")"=w912, "State(s) at Back (\"\")"="Data: Cleanup\nExit") -> ("States Out"=w910:string)  [unwired: 13 in]
        n398 = call <vilib>:"Add State(s) to Queue__jki_lib_state_machine.vi"("State(s) in Front (\"\")"=w910, "State(s) in (\"\")"=w919) -> ("States Out"=w918:string)  [unwired: 13 in]
      }
      frame "----------Valve Control----------" {
        n399 = call <vilib>:"Add State(s) to Queue__jki_lib_state_machine.vi"("State(s) in (\"\")"=w921) -> ("States Out"=w923:string)  [unwired: 14 in]
      }
      frame "Main Power" {
        w929 = T85 30 items=["4-20_OUT", "Pres_HI1", "Pres_HI2", "Pres_LOW", "Pres_PIN", "HEATER_TOP", "HEATER_BOT", "T_Shell", "FLOWMETER", "WATT_SENSE", "WH_TICK", "Tc_1", "Tc_2", "Tc_3", "Tc_4", "Tc_5", "Tc_6", "Tc_down", "T_Shell_2", "T_Shell_3", "T_Shell_4", "RTD_IN", "RTD_OUT", "RTD_AMB", "INTF_TEMPFLO", "INTF_READY", "INTF_START", "INTF_STOP", "DRM_LOW", "DRM_HIGH", "PWR_MAIN", "VLV_DUMP", "VLV_OUT", "VLV_IN", "WATT_HOURS", "FLOW(SAMPLE)", "GALLONS", "FLOW(GPM)"] ("Channel_Enum")
        n400 = Unbundle By Name(w931) -> ("Washer Controls.Test Fixture Hardware.Analog Data.Yokogawa.MW100"=w927:refnum<visa-resource-name>, "User Controls.Main Power Control"=w924:bool)
        n401 = Boolean To (0,1)(Boolean=w924) -> (0, 1=w928:i16)
        n402 = call "INTELLIFAUCET DO Control.vi"("VISA session"=w927, "HEWH MW100 Channel Numbers"=w929, "Relay Status (0:CLOSED)"=w928, "Error In"=w926) -> ("error out"=w925:errorcluster)  [unwired: 9 in, 2 out]
        n403 = call <vilib>:"Add State(s) to Queue__jki_lib_state_machine.vi"("State(s) in (\"\")"=w930) -> ("States Out"=w932:string)  [unwired: 14 in]
      }
      frame "Outlet Valve 1" {
        n404 = Unbundle By Name(w938) -> ("Washer Controls.Test Fixture Hardware.Analog Data.Yokogawa.MW100"=w936:refnum<visa-resource-name>)
        n405 = local read "Out VLV UI"() -> (w933:enum8{"CLOSE", "OPEN"})
        n406 = call "HEWH Solenoid Output Set.vi"("Error In"=w935, "OPEN CLOSE"=w933, "VISA session"=w936) -> ("Error Out"=w934:errorcluster)  [unwired: 7 in, 1 out]
        n407 = call <vilib>:"Add State(s) to Queue__jki_lib_state_machine.vi"("State(s) in (\"\")"=w937) -> ("States Out"=w939:string)  [unwired: 14 in]
      }
      frame "In Valve 1" {
        n408 = Unbundle By Name(w945) -> ("Washer Controls.Test Fixture Hardware.Analog Data.Yokogawa.MW100"=w943:refnum<visa-resource-name>)
        n409 = local read "In Valve UI"() -> (w940:enum8{"OPEN", "CLOSE"})
        n410 = call "Solenoid - Fill.vi"("Error In"=w942, "VALVE OPEN CLOSE"=w940, "VISA session"=w943) -> ("Error Out"=w941:errorcluster)  [unwired: 7 in, 1 out]
        n411 = call <vilib>:"Add State(s) to Queue__jki_lib_state_machine.vi"("State(s) in (\"\")"=w944) -> ("States Out"=w946:string)  [unwired: 14 in]
      }
      frame "Drain Valve 1" {
        n412 = Unbundle By Name(w952) -> ("Washer Controls.Test Fixture Hardware.Analog Data.Yokogawa.MW100"=w948:refnum<visa-resource-name>)
        n413 = local read "Drain VLV UI"() -> (w947:enum8{"OPEN", "CLOSE"})
        n414 = call "Solenoid - DRAIN.vi"("Error In"=w950, "VALVE OPEN CLOSE"=w947, "VISA session"=w948) -> ("Error Out"=w949:errorcluster)  [unwired: 7 in, 1 out]
        n415 = call <vilib>:"Add State(s) to Queue__jki_lib_state_machine.vi"("State(s) in (\"\")"=w951) -> ("States Out"=w953:string)  [unwired: 14 in]
      }
      frame "--------Intellifaucet Control------" {
        n416 = call <vilib>:"Add State(s) to Queue__jki_lib_state_machine.vi"("State(s) in (\"\")"=w956) -> ("States Out"=w957:string)  [unwired: 14 in]
      }
      frame "Start Intellifaucet" {
        n417 = Unbundle By Name(w960) -> ("Washer Controls.Test Fixture Hardware.Analog Data.Yokogawa.MW100"=w959:refnum<visa-resource-name>)
        n418 = call "Intellifaucet_Driver.vi"("VISA session"=w959, "Mode"=INTELLIFAUCET_Set_Mode."Start Flow", "Error In"=w961) -> ("Error Out"=w958:errorcluster)  [unwired: 9 in, 3 out]
        n419 = call <vilib>:"Add State(s) to Queue__jki_lib_state_machine.vi"("State(s) in (\"\")"=w963) -> ("States Out"=w964:string)  [unwired: 14 in]
      }
      frame "Stop Intellifaucet" {
        n420 = Unbundle By Name(w967) -> ("Washer Controls.Test Fixture Hardware.Analog Data.Yokogawa.MW100"=w966:refnum<visa-resource-name>)
        n421 = call "Intellifaucet_Driver.vi"("VISA session"=w966, "Mode"=INTELLIFAUCET_Set_Mode."Stop Flow", "Error In"=w968) -> ("Error Out"=w965:errorcluster)  [unwired: 9 in, 3 out]
        n422 = call <vilib>:"Add State(s) to Queue__jki_lib_state_machine.vi"("State(s) in (\"\")"=w970) -> ("States Out"=w971:string)  [unwired: 14 in]
      }
      frame "Adjust Temp" {
        n423 = Unbundle By Name(w977) -> ("Washer Controls.Test Fixture Hardware.Analog Data.Yokogawa.MW100"=w973:refnum<visa-resource-name>, "User Controls.Intellifaucet Temperature"=w972:dbl)
        n424 = call "Intellifaucet_Driver.vi"("VISA session"=w973, "Mode"=INTELLIFAUCET_Set_Mode."Adjust Temp", "Temperature(F)"=w972, "Error In"=w975) -> ("Error Out"=w974:errorcluster)  [unwired: 8 in, 3 out]
        n425 = call <vilib>:"Add State(s) to Queue__jki_lib_state_machine.vi"("State(s) in (\"\")"=w978) -> ("States Out"=w979:string)  [unwired: 14 in]
      }
      frame "Adjust Flow" {
        n426 = Unbundle By Name(w985) -> ("Washer Controls.Test Fixture Hardware.Analog Data.Yokogawa.MW100"=w981:refnum<visa-resource-name>, "User Controls.Percent Flow"=w980:dbl)
        n427 = call "Intellifaucet_Driver.vi"("VISA session"=w981, "Mode"=INTELLIFAUCET_Set_Mode."Adjust Flow", "Flow Rate (GPM)"=w980, "Error In"=w983) -> ("Error Out"=w982:errorcluster)  [unwired: 8 in, 3 out]
        n428 = call <vilib>:"Add State(s) to Queue__jki_lib_state_machine.vi"("State(s) in (\"\")"=w986) -> ("States Out"=w987:string)  [unwired: 14 in]
      }
      frame "---------- Main Control ----------" {
        n429 = call <vilib>:"Add State(s) to Queue__jki_lib_state_machine.vi"("State(s) in (\"\")"=w991) -> ("States Out"=w990:string)  [unwired: 14 in]
      }
      frame "Check for UI Event" {
        # "Shut the power off at the 1 hour mark for First Hour Delivery and 23 hour mark\nfor 24 Hour Rating"
        # "Clear variable"
        n430 = Unbundle By Name(w994) -> ("User Controls"=w993:T28)
        n431 = local read "Program Names Update"() -> (w999:T25)
        n432 = local read "Shutdown"() -> (w1001:string)
        n433 = local read "Draw Time"() -> (w992:T20)
        n434 = call "HEWH Program Type.vi"("Program Names"=w999) -> ("Test_Type:"=w996:string)  [unwired: 9 in, 1 out]
        n435 = case shown="\"Stand Override\", Default" w996 {
          tunnel: ["" ("State(s) in Front (\"\")") w1008 w1014] -> w995
          tunnel: w993 -> [w1005 w1010 w1013]
          tunnel: [w1005 w1009 w1012] -> _
          tunnel: w992 -> [_ w1006 w1011]
          frame "Stand Override", Default {
          }
          frame "24 Hour Rating" {
            n436 = call "HEWH Cut Power.vi"("Cut Power At Time (Sec)"=T20 82800.0 ("y"), "Current Draw Time (Sec)"=w1006, "User Controls in"=w1010) -> ("States Output"=w1008:string, "User Controls out"=w1009:T28)  [unwired: 7 in]
          }
          frame "First Hour Rating" {
            n437 = call "HEWH Cut Power.vi"("Cut Power At Time (Sec)"=T20 3600.0 ("y"), "Current Draw Time (Sec)"=w1011, "User Controls in"=w1013) -> ("States Output"=w1014:string, "User Controls out"=w1012:T28)  [unwired: 7 in]
          }
        }
        n438 = call <vilib>:"Add State(s) to Queue__jki_lib_state_machine.vi"("State(s) in Front (\"\")"=w1001, "State(s) in (\"\")"=w1003) -> ("States Out"=w1000:string)  [unwired: 13 in]
        n439 = flat-sequence {
          tunnel: w1000 -> [w1016]
          tunnel: [w1016] -> w998
          frame #0 {
            n440 = local write "Shutdown"("" ("Shutdown")) -> ()
          }
        }
        n441 = call <vilib>:"Add State(s) to Queue__jki_lib_state_machine.vi"("State(s) in Front (\"\")"=w995, "State(s) in (\"\")"=w998) -> ("States Out"=w997:string)  [unwired: 13 in]
      }
      frame "Gather Data" {
        # "I scan the aglilent and MW at the \nsame time. This allows for an \nadditional 0.5 second scan rate"
        n442 = Unbundle By Name(w1032) -> ("Washer Controls.Test Fixture Hardware.Analog Data.Yokogawa.MW100"=w1021:refnum<visa-resource-name>, "Core HEWH Data"=w1019:T73, "User Controls.GEA2?"=w1020:bool)
        n443 = call "UTILITY E-Time.vi"("error in (no error)"=w1033) -> ("error out"=w1031:errorcluster, "Elapsed Time (sec)"=w1024:dbl)  [unwired: 8 in, 1 out]
        "Elapsed Time" <- w1024
        n444 = local read "Message"() -> (w1029:T23)
        n445 = control-ref of="Tank Display"() -> (w1023:refnum<vi>)
        n446 = local read "Current"() -> (w1022:T19)
        n447 = Build Array(T23 "Program Status" ("element"), w1029) -> (w1027:T23[])
        n448 = call "HEWH Gather Test Data.vi"("MW100"=w1021, "Core HEWH Data Station A"=w1019, "GEA2?"=w1020, "error in (no error)"=w1031, 7:w1024, 11:w1023, 12:w1022) -> ("Core HEWH Data Station A"=w1018:T83, "MW100 Full Data"=w1025:string[][], "error out"=w1030:errorcluster)  [unwired: 8 in, 2 out]
        n449 = Build Array (concatenate)(w1025, w1027) -> (→"MW100 Data":T23[][])
        n450 = Bundle By Name(cluster=w1032, "Core HEWH Data"=w1018) -> (w1034:T76)
        n451 = call <vilib>:"Add State(s) to Queue__jki_lib_state_machine.vi"("State(s) in (\"\")"=w1036) -> ("States Out"=w1035:string)  [unwired: 14 in]
      }
      frame "Update Power Display" {
        n452 = Unbundle By Name(w1038) -> ("User Controls.GEA2?"=w1051:bool, "Core HEWH Data.HEWH Specific DAQ.Power State"=w1052:T12, "Core HEWH Data.HEWH Specific DAQ.Power Analyzer"=w1046:T14, "Core HEWH Data.HEWH Specific DAQ.HEWH Data"=w1040:T13)
        n453 = Unbundle By Name(w1040) -> ("HEWH Standard.Gallons (Gal)"=→"Gallons" →"Total Dispensed Gallons":dbl, "HEWH Standard.TC Tree (AVG)"=→"TC Tree Average":dbl, "HEWH Standard.Flow Rate (GPM)"=→"Flow Rate (GPM)" →"Flow Meter 2" →"Flow Meter":dbl, "HEWH Standard.Voltage (Volts)"=w1045:dbl, "HEWH Standard.Current (Amps)"=w1044:dbl, "HEWH Standard.Power (Watts)"=w1043:dbl, "HEWH Standard.WattHours (Wh)"=w1042:dbl)
        n454 = case shown="False" w1051 {
          tunnel: w1052 -> [_ w1060]
          frame True {
            # "If it has GEA2 let the DAQ loop take care\nof the display"
          }
          frame False, Default {
            # "If no GEA2, skip this section and try to determine\nthe state from the MW100 (I use DI from both Upper\nand Lower elements. I set a current range for the compressor\nand fan. If its above 0.5 A and less than 5A)"
            n455 = call "HEWH Power Notifier.vi"("Status"=UTILITY_Notifier."Set", "Set Status"=w1060, "name (unnamed)"="Power") -> ()  [unwired: 7 in, 2 out]
            "POWER" <- w1060
          }
        }
        n456 = case shown="\"APLUS\", Default" w1046 {
          tunnel: w1045 -> [w1058 _]
          tunnel: w1044 -> [w1057 _]
          tunnel: w1043 -> [w1056 _]
          tunnel: w1042 -> [w1055 _]
          frame "APLUS", Default {
            "Voltage (Volts)" <- w1058
            "Current" <- w1057
            "Power (Watts)" <- w1056
            "Watt Hours (Wh)" <- w1055
          }
          frame "WT300" {
          }
        }
        n457 = call "UTILITY E-Time.vi"("error in (no error)"=w1050) -> ("error out"=w1049:errorcluster, "Elapsed Time (sec)"=→"Power Display Time":dbl)  [unwired: 8 in, 1 out]
        n458 = call <vilib>:"Add State(s) to Queue__jki_lib_state_machine.vi"("State(s) in Front (\"\")"="", "State(s) in (\"\")"=w1054) -> ("States Out"=w1053:string)  [unwired: 13 in]
      }
      frame "Check For Draw" {
        n459 = local read "Program Names Update"() -> (w1069:T25)
        n460 = local read "Purge Time (Seconds)"() -> (w1064:T19)
        n461 = Unbundle By Name(w1067) -> ("Core HEWH Data"=w1068:T73)
        n462 = call "HEWH Check For Draw.vi"("Purge Time (Seconds)"=w1064, "Core HEWH Data in"=w1068, "Program Names Update"=w1069) -> ("State(s) in Front (\"\")"=w1070:string, "Core HEWH Data out"=w1066:T1, "Display Message"=w1063:string)  [unwired: 6 in]
        n463 = local write "Message"(w1063) -> ()
        n464 = Bundle By Name(cluster=w1067, "Core HEWH Data"=w1066) -> (w1065:T76)
        n465 = call <vilib>:"Add State(s) to Queue__jki_lib_state_machine.vi"("State(s) in Front (\"\")"=w1070, "State(s) in (\"\")"=w1072) -> ("States Out"=w1062:string)  [unwired: 13 in]
      }
      frame "Draw Time" {
        # "This is the time when the draw started. This is the time value that is used \nto determine when the next draw happens"
        n466 = call "UTILITY E-Time.vi"("error in (no error)"=w1077) -> ("error out"=w1076:errorcluster, "Elapsed Time (sec)"=w1073:dbl)  [unwired: 8 in, 1 out]
        "Draw Time" <- w1073
        n467 = local write "Message"(T23 "" ("Message")) -> ()
        n468 = Bundle By Name(cluster=w1075, "Core HEWH Data.Current Draw Time"=w1073) -> (w1074:T76)
        n469 = call <vilib>:"Add State(s) to Queue__jki_lib_state_machine.vi"("State(s) in (\"\")"=w1078) -> ("States Out"=w1080:string)  [unwired: 14 in]
      }
      frame "Start Multi Draw" {
        n470 = Unbundle By Name(w1082) -> ("Core HEWH Data.Draw Count"=w1086:i32, "Core HEWH Data.Test Patten Setup"=w1083:T74)
        n471 = Unbundle By Name(w1082) -> ("Core HEWH Data"=w1081:T73)
        n472 = Unbundle By Name(w1083) -> ("Total Gallons Schedule"=w1095:dbl[], "Flow Rate Schedule"=w1094, "Incoming Water Temperature"=w1093)
        n473 = call "HEWH Remaining Draws.vi"("Core HEWH Data"=w1081) -> ("Remaining Draws"=w1087:i32)  [unwired: 10 in]
        "Remaining Draws" <- w1087
        n474 = local read "Program Names Update"() -> (w1084:T25)
        n475 = call "HEWH Program Type.vi"("Program Names"=w1084) -> ("Program Type"=w1085:string)  [unwired: 9 in, 1 out]
        n476 = Index Array(array=w1095, index=w1086) -> (element=w1091:dbl)
        n477 = Index Array(array=w1094, index=w1086) -> (element=w1090)
        n478 = Index Array(array=w1093, index=w1086) -> (element=w1089)
        n479 = Equal To 0?(x=w1087) -> (x = 0?=w1088:bool)
        n480 = case shown="True" w1088 {
          tunnel: ["Dispense Gallons" ("State(s) in Front (\"\")") w1101] -> w1092
          tunnel: w1085 -> [_ w1100]
          frame False {
          }
          frame True {
            n481 = case shown="\"24 Hour Rating\"" w1100 {
              tunnel: ["" ("State(s) in Front (\"\")") "Wait for Heat Cutout" ("State(s) in Front (\"\")") "" ("State(s) in Front (\"\")") "" ("State(s) in Front (\"\")") "" ("State(s) in Front (\"\")")] -> w1101
              frame "Stand Override", Default {
              }
              frame "24 Hour Rating" {
              }
              frame "First Hour Rating" {
              }
              frame "Heat Up" {
              }
              frame "Channel Tester" {
              }
            }
          }
        }
        n482 = local write "Gallon Target"(w1091) -> ()
        n483 = local write "GPM Target"(w1090) -> ()
        n484 = local write "Temperature"(w1089) -> ()
        n485 = call <vilib>:"Add State(s) to Queue__jki_lib_state_machine.vi"("State(s) in Front (\"\")"=w1092, "State(s) in (\"\")"=w1097) -> ("States Out"=w1098:string)  [unwired: 13 in]
      }
      frame "Dispense Gallons" {
        n486 = flat-sequence {
          tunnel: w1110 -> [w1114]
          tunnel: [w1114] -> w1109
          tunnel: w1109 -> [w1116]
          tunnel: [w1116] -> w1108
          tunnel: w1108 -> [w1118]
          tunnel: [w1118] -> w1107
          frame #0 {
            n487 = local write "Dispense"(TRUE ("Start Draw?")) -> ()
          }
          frame #1 {
            n488 = Wait (ms)(milliseconds to wait=u32 500) -> ()  [unwired: 1 out]
          }
          frame #2 {
            n489 = local write "Dispense"(FALSE ("Start Draw?")) -> ()
          }
        }
        n490 = call <vilib>:"Add State(s) to Queue__jki_lib_state_machine.vi"("State(s) in (\"\")"=w1112) -> ("States Out"=w1113:string)  [unwired: 14 in]
      }
      frame "----------24 Hour Rating---------" {
        n491 = call <vilib>:"Add State(s) to Queue__jki_lib_state_machine.vi"("State(s) in (\"\")"=w1122) -> ("States Out"=w1123:string)  [unwired: 14 in]
      }
      frame "Wait for Heat Cutout" {
        # "The DAQ loops takes time\n to get to 1 sec intervals.\nWhen you scan the GEA2\n too fast...it can throw\ngarbage"
        # "The wait for Heat Cutout is called twice in the 24 Hour Rating. The first call is before the first draw. The last is after \nthe last draw."
        n492 = local read "Draw Count"() -> (w1130:T22)
        n493 = local read "Loop Time"() -> (w1127:dbl)
        n494 = Equal?(x=w1130, y=u8 0) -> (x = y?=w1128:bool)
        n495 = Greater?(x=w1127, y=0.8) -> (0:w1125:bool)
        n496 = And(x=w1128, y=w1125) -> (x .and. y?=w1132:bool)
        n497 = local read "Full Cutout"() -> (w1124:bool)
        n498 = local write "Message"(T23 "Waiting for Heat Source Cutout...." ("Message")) -> ()
        n499 = case shown="True" w1124 {
          tunnel: [w1139 "Wait for Temp Decline"] -> w1134
          tunnel: w1132 -> [w1138 _]
          frame False {
            n500 = case shown="True" w1138 {
              tunnel: ["Check for UI Event\nGather Data\nUpdate Power Display\nCheck For Draw\nDraw Time\nWait for Heat Cutout" ("State(s) in Front (\"\")") "Check for UI Event\nGather Data\nUpdate Power Display\nWait for Heat Cutout" ("State(s) in Front (\"\")")] -> w1139
              frame False {
              }
              frame True {
              }
            }
          }
          frame True {
          }
        }
        n501 = call <vilib>:"Add State(s) to Queue__jki_lib_state_machine.vi"("State(s) in Front (\"\")"=w1134, "State(s) in (\"\")"=w1136) -> ("States Out"=w1137:string)  [unwired: 13 in]
      }
      frame "Wait for Temp Decline" {
        # "Validate this routine"
        n502 = Unbundle By Name(w1147) -> ("Core HEWH Data.HEWH Specific DAQ.HEWH Data.HEWH Standard.TC Tree (AVG)"=→"Average TC Tree Temperature":dbl, "Core HEWH Data"=w1148:T73)
        n503 = local read "Program Names Update"() -> (w1143:T25)
        n504 = local read "Draw Time"() -> (w1149:T20)
        n505 = call "HEWH Wait For Temp Decline.vi"("Core HEWH Data"=w1148, "Program Names"=w1143, "Draw Time"=w1149) -> ("State(s) in Front (\"\")"=w1144:string, "Core HEWH Data Output"=w1145:T83)  [unwired: 14 in, 1 out]
        n506 = Bundle By Name(cluster=w1147, "Core HEWH Data"=w1145) -> (w1146:T76)
        n507 = call <vilib>:"Add State(s) to Queue__jki_lib_state_machine.vi"("State(s) in Front (\"\")"=w1144, "State(s) in (\"\")"=w1152) -> ("States Out"=w1153:string)  [unwired: 13 in]
      }
      frame "Wait for Finish Time" {
        # "The predraw for the new standard is basically\nrunning the test twice...this allows for that."
        # "Wait for 24 Hours before completing the test."
        # "24 Hours"
        n508 = Unbundle By Name(w1155) -> ("Core HEWH Data.Current Draw Time"=w1154:dbl)
        n509 = Greater Or Equal?(x=w1154, y=86400.0) -> (x >= y?=w1157:bool)
        "24 Hr Test Complete" <- w1157
        n510 = local write "Message"(T23 "Waiting for End Time...." ("Message")) -> ()
        n511 = case shown="True" w1157 {
          tunnel: ["Gather Data\nUpdate Power Display\nDraw Time\nCheck For Draw\nCheck for UI Event\nWait for Finish Time" ("State(s) in Front (\"\")") "Add Headers" ("State(s) in Front (\"\")")] -> w1159
          frame False {
            # "Test not complete..continue \nscanning"
          }
          frame True {
            # "Test finished"
          }
        }
        n512 = call <vilib>:"Add State(s) to Queue__jki_lib_state_machine.vi"("State(s) in Front (\"\")"=w1159, "State(s) in (\"\")"=w1161) -> ("States Out"=w1162:string)  [unwired: 13 in]
      }
      frame "----------First Hour Rating--------" {
        n513 = call <vilib>:"Add State(s) to Queue__jki_lib_state_machine.vi"("State(s) in (\"\")"=w1167) -> ("States Out"=w1168:string)  [unwired: 14 in]
      }
      frame "First Hour Cutout" {
        w1178 = TRUE
        # "Setup Terminate Cond."
        n514 = Unbundle By Name(w1176) -> ("Core HEWH Data"=w1175:T73)
        n515 = local read "Water Heater GEA2 Data"() -> (w1172:T36)
        n516 = local read "Full Cutout"() -> (w1170:bool)
        n517 = call "HEWH First Hour Cutout.vi"("T2 Degree Diff for Purge"="T2 Degree Diff for Purge", "Water Heater GEA2 Data"=w1172, "Core HEWH Data in"=w1175, "Full Cutout"=w1170) -> ("Core HEWH Data out"=w1174:T1, "State(s) in Front (\"\")"=w1169:string)  [unwired: 6 in]
        n518 = local write "Message"(T23 "Waiting for Cutout...." ("Message")) -> ()
        n519 = Bundle By Name(cluster=w1176, "Core HEWH Data.Condition Cluster Output.Condition #5"=w1178, "Core HEWH Data.Condition Cluster Output.Condition #3"=w1178, "Core HEWH Data.Condition Cluster Output.Decrease Outlet Temperature \nBy (RTD Out)"="Decrease Outlet\nTemperature By (RTD Out)", "Core HEWH Data"=w1174) -> (w1173:T76)
        n520 = call <vilib>:"Add State(s) to Queue__jki_lib_state_machine.vi"("State(s) in Front (\"\")"=w1169, "State(s) in (\"\")"=w1181) -> ("States Out"=w1182:string)  [unwired: 13 in]
      }
      frame "First Hour Last Draw Check" {
        # "Determine purge time for last draw"
        # "This is a flag. If the system is heating, go ahead and do the \nlast draw. If it is not heating (False)...that means it just finished with a draw"
        # "If a draw is not occurring at an elapsed time of one hour,\na final draw shall be imposed at one hour.\nThis draw shall proceed for a minimum of 30\nseconds and shall be immediately terminated\nthereafter when the outlet temperature first\nindicates a value less than or equal to the cutoff\ntemperature used for the previous draw"
        n521 = local read "Draw Time"() -> (w1190:T20)
        n522 = call "HEWH Remaining Time.vi"("Ideal Purge Time"=60.0, "Current Draw Timer"=w1190, "Total Test Timer (1hr)"="Total Test Timer (1hr)") -> ("Purge Time"=w1186:dbl, "Start Draw/Purge Sequence"=w1187:bool, "Test Complete"=w1188:bool)  [unwired: 6 in]
        n523 = Unbundle By Name(w1184) -> ("Heating Flag"=w1183)
        n524 = case shown="True" w1187 {
          tunnel: ["" w1204] -> w1193
          tunnel: w1184 -> [w1197 w1202]
          tunnel: [w1197 w1201] -> w1192
          tunnel: w1183 -> [_ w1203]
          tunnel: w1188 -> [_ w1200]
          tunnel: w1186 -> [_ w1199]
          frame False {
          }
          frame True {
            n525 = case shown="True" w1203 {
              tunnel: [w1207 ""] -> w1204
              tunnel: w1202 -> [w1206 w1213]
              tunnel: [w1206 w1212] -> w1201
              tunnel: w1200 -> [w1205 _]
              tunnel: w1199 -> [_ w1214]
              frame False {
                n526 = case shown="True" w1205 {
                  tunnel: ["" ("State(s) in Front (\"\")") "Add Headers" ("State(s) in Front (\"\")")] -> w1207
                  frame False {
                  }
                  frame True {
                    # "Test finished"
                    # "Shut Down DAQ Loop"
                    n527 = local write "Shutdown DAQ"("Get Final Data\nExit" ("Shutdown DAQ")) -> ()
                  }
                }
              }
              frame True {
                w1211 = TRUE ("Mult-Draw")
                n528 = local write "Purge Time (Seconds)"(w1214) -> ()
                n529 = Bundle By Name(cluster=w1213, "Special Last Draw"=w1211) -> (w1212:T76)
                "Special Last Draw" <- w1211
              }
            }
          }
        }
        n530 = local write "Message"(T23 "Checking for Last Draw...." ("Message")) -> ()
        n531 = call <vilib>:"Add State(s) to Queue__jki_lib_state_machine.vi"("State(s) in Front (\"\")"=w1193, "State(s) in (\"\")"=w1195) -> ("States Out"=w1196:string)  [unwired: 13 in]
      }
      frame "Record Min and Max RTD" {
        # "Get Final Draw Timestamp"
        # "FlowRate"
        n532 = Unbundle By Name(w1227) -> ("Core HEWH Data.Calc and Calibration.RTD Max Min Array"=w1229:dbl[][], "Core HEWH Data.Calc and Calibration.Draw Start Time"=w1223:dbl, "Core HEWH Data.Draw Count"=w1232:i32, "Core HEWH Data.Calc and Calibration.Max RTD Temp\nDuring Draw"=w1231:dbl, "Core HEWH Data.Calc and Calibration.Min RTD Temp\nDuring Draw"=w1230:dbl, "Core HEWH Data.Calc and Calibration.Draw Statistics"=w1221:dbl[][], "Core HEWH Data.HEWH Specific DAQ.HEWH Data.HEWH Standard.Gallons (Gal)"=w1216:dbl)
        n533 = local read "Draw Time"() -> (w1220:T20)
        n534 = Index Array(array=w1221, index (col)=0 ("disabled index (col)")) -> (element=w1219:dbl[])  [unwired: 1 in]
        n535 = call <vilib>:"Std Deviation and Variance.vi"("X"=w1219) -> ("mean"=w1218:dbl, "standard deviation"=w1217:dbl)  [unwired: 1 in, 1 out]
        n536 = Build Array(w1223, w1220, w1232, w1231, w1230, w1218, w1217, w1216) -> (w1228:T20[])
        n537 = local write "Message"(T23 "Recording Max/Min RTD...." ("Message")) -> ()
        n538 = Build Array (concatenate)(w1229, w1228) -> (w1225:T20[][])
        "RTD Max Min Array" <- w1225
        n539 = Bundle By Name(cluster=w1227, "Core HEWH Data.Calc and Calibration.RTD Max Min Array"=w1225) -> (w1226:T76)
        n540 = call <vilib>:"Add State(s) to Queue__jki_lib_state_machine.vi"("State(s) in (\"\")"=w1234) -> ("States Out"=w1235:string)  [unwired: 14 in]
      }
      frame "---------Finalize Output File-------" {
        n541 = call <vilib>:"Add State(s) to Queue__jki_lib_state_machine.vi"("State(s) in (\"\")"=w1238) -> ("States Out"=w1239:string)  [unwired: 14 in]
      }
      frame "Add Headers" {
        # "Shut Down UI Loop"
        # "Make sure I get the latest\nFinal Data. If no delay..it wont have\ntime to finish the second state machine\nand will give wrong data"
        # "If the quit button is pressed and it has a file path. Go\nahead and add the final headers to the file"
        n542 = flat-sequence {
          tunnel: [w1262] -> w1248
          tunnel: w1249 -> [w1262]
          frame #0 {
            # "Shut Down DAQ Loop"
            "Shutdown DAQ" <- "Get Final Data\nExit" ("Shutdown DAQ")
          }
        }
        n543 = Unbundle By Name(w1246) -> ("Core HEWH Data.Calc and Calibration.RTD Max Min Array"=w1245:dbl[][])
        n544 = while {
          tunnel: [w1260] -> w1243
          stop <- w1259 stop-if-true
          n545 = local read "Final Data Cluster"() -> (w1260:T1)
          n546 = local read "DAQ Loop Complete"() -> (w1259:bool)
          n547 = Wait Until Next ms Multiple(millisecond multiple=u32 100) -> ()  [unwired: 1 out]
        }
        n548 = local read "Save File Path"() -> (w1242:path)
        n549 = call "UTILITY Delay mS.vi"("Error In"=w1248, "milliseconds to wait"=u32 5000) -> ("Error Out"=w1244:errorcluster)  [unwired: 13 in]
        n550 = Equal?(x=w1242, y=path "") -> (x = y?=w1250:bool)
        n551 = local read "Sofware Version"() -> (w1241:T23)
        n552 = local write "Message"(T23 "Creating Output File...." ("Message")) -> ()
        n553 = call "HEWH Save Final Data.vi"("RTD Max Min Array"=w1245, "No Path?"=w1250, "Final Data Cluster"=w1243, "error in (no error)"=w1244, "Save File Path"=w1242, "Sofware Version"=w1241) -> ("Data With Header"=→"Data With Header":string[][], "error out"=w1253:errorcluster)  [unwired: 8 in]
        n554 = flat-sequence {
          tunnel: w1253 -> [w1264]
          tunnel: [w1264] -> w1254
          frame #0 {
            n555 = local write "Shutdown Sequence"("Exit" ("State(s) in Front (\"\")")) -> ()
            n556 = local write "Message"(T23 "Complete...." ("Message")) -> ()
          }
        }
        n557 = call <vilib>:"Add State(s) to Queue__jki_lib_state_machine.vi"("State(s) in Front (\"\")"="Macro: Exit" ("State(s) in Front (\"\")"), "State(s) in (\"\")"=w1256) -> ("States Out"=w1257:string)  [unwired: 13 in]
      }
    }
    n558 = case shown="True" "Debug" {
      tunnel: w545 -> [w556 w559]
      tunnel: [w556 w558] -> w544
      tunnel: w543 -> [_ w557]
      frame False {
      }
      frame True {
        n559 = Build Array (concatenate)(w559, w557) -> (w558:string[])
        "States" <- w558
      }
    }
  }
  "Error Out" <- w60
  n560 = while "Heat Up Test" {
    shift-right: [w1269] -> _
    shift-left: _ -> [w1268]
    shift-right: [w1272] -> _
    shift-left: _ -> [w1266]
    shift-right: [w1271] -> _
    shift-left: w53 -> [w1273]
    stop <- w1270 stop-if-true
    w1267 = 1000  # Timeout
    # "Heat Up Test"
    n561 = call <vilib>:"Parse State Queue__jki_lib_state_machine.vi"("State Queue"=w1273, "Error In (no error)"=w1266) -> ("Remaining States"=w1275:string, "Current State"=w1276:string, "Arguments"=w1274:string)  [unwired: 11 in]
    n562 = case shown="\"Step 1\"" w1276 {
      selector: w1276 -> [_ _ w1328 _ _ _ _ _ _ _ _ _ _ _ _ _ _ _ _ _ _ _ _]
      tunnel: w1275 -> [w1283 w1327 w1332 w1344 w1349 w1353 w1358 w1368 w1373 w1377 w1384 w1394 w1409 w1444 w1495 w1544 w1577 w1609 w1702 w1752 w1774 w1797 w1817]
      tunnel: w1274 -> [_ _ _ _ _ _ _ _ _ _ _ _ _ _ _ _ _ _ _ _ _ _ _]
      tunnel: w1268 -> [w1281 w1324 w1330 w1341 w1347 w1350 _ w1365 w1370 w1374 w1382 w1391 w1402 w1438 w1487 w1542 w1575 w1607 w1693 w1750 w1772 w1795 w1815]
      tunnel: [w1280 w1325 w1334 errorcluster {"status"=FALSE, "code"=0, "source"=""} ("error out") w1346 w1351 w1355 w1366 w1371 w1375 w1380 w1392 w1403 w1439 w1489 w1541 w1574 w1599 w1698 w1745 w1769 w1793 w1814] -> w1272
      tunnel: w1266 -> [w1279 w1325 w1333 w1340 w1346 w1351 w1355 w1366 w1371 w1375 w1381 w1392 w1407 w1437 w1488 w1541 w1574 w1603 w1699 w1749 w1771 w1794 w1814]
      tunnel: [w1282 w1326 w1331 w1343 w1348 w1352 w1357 w1367 w1372 w1376 w1383 w1393 w1408 w1443 w1494 w1543 w1576 w1608 w1701 w1751 w1773 w1796 w1816] -> w1271
      tunnel: [_ _ _ _ TRUE _ _ _ _ _ _ _ _ _ _ _ _ _ _ _ _ _ _] -> w1270
      tunnel: [w1278 w1324 w1330 w1341 w1347 w1350 w1356 w1365 w1370 w1374 w1382 w1391 w1402 w1438 w1487 w1542 w1575 w1607 w1693 w1750 w1772 w1795 w1815] -> w1269
      tunnel: w1267 -> [w1277 _ _ _ _ _ _ _ _ _ _ _ _ _ _ _ _ _ _ _ _ _ _]
      frame "", "Idle" {
        n563 = event shown="[1] \"Start Heat Up Test\": Value Change" {
          selector: _ -> [_ _ _]
          dyn-events: _ -> [_ _ _]
          timeout: w1277 -> [_ _ _]
          tunnel: w1283 -> [w1293 w1310 w1323]
          tunnel: [w1292 w1309 w1322] -> w1282
          tunnel: w1281 -> [w1289 w1308 w1320]
          tunnel: [w1290 w1304 w1321] -> w1280
          tunnel: w1279 -> [w1288 w1305 w1321]
          tunnel: [w1289 w1307 w1320] -> w1278
          event Timeout {
            # "Set the correct\nfile/program type"
            n564 = event-data() -> ()  [unwired: 1 in, 1 out]
            n565 = local read "Program Names Update"() -> (w1287:T25)
            n566 = call "HEWH Program Type.vi"("Program Names"=w1287) -> ("Test_Type:"=w1286:string)  [unwired: 9 in, 1 out]
            n567 = Equal?(x=w1286, y="Heat Up") -> (x = y?=w1284:bool)
            n568 = case shown="True" w1284 {
              tunnel: ["Check Exit" w1298] -> w1291
              tunnel: [w1295 w1297] -> w1290
              tunnel: w1288 -> [w1295 w1296]
              frame False {
              }
              frame True {
                n569 = local read "Start DAQ Write"() -> (w1299:bool)
                n570 = case shown="True" w1299 {
                  tunnel: ["" "Set Mode"] -> w1298
                  tunnel: w1296 -> [w1300 w1302]
                  tunnel: [w1300 w1302] -> w1297
                  frame False {
                  }
                  frame True {
                  }
                }
              }
            }
            n571 = call <vilib>:"Add State(s) to Queue__jki_lib_state_machine.vi"("State(s) in Front (\"\")"=w1291, "State(s) in (\"\")"=w1293) -> ("States Out"=w1292:string)  [unwired: 13 in]
          }
          event "Start Heat Up Test": Value Change {
            n572 = event-data() -> ()  [unwired: 1 in, 6 out]
            n573 = flat-sequence {
              tunnel: w1305 -> [w1314]
              tunnel: w1308 -> [w1316]
              tunnel: [w1315] -> w1307
              tunnel: [w1313] -> w1306
              tunnel: [w1317] -> w1304
              tunnel: w1306 -> [w1317]
              frame #0 {
                n574 = call "HEWH Select Unit Type.vi"("error in (no error)"=w1314) -> ("error out"=w1313:errorcluster, "Unit Type"=w1312:string)  [unwired: 9 in]
                n575 = Bundle By Name(cluster=w1316, "Unit Type"=w1312) -> (w1315:cluster{"Unit Type":string})
              }
              frame #1 {
                n576 = local write "Shutdown"("File Setup\nStart DAQ Write\nReset Totalizer" ("State(s) in Front (\"\")")) -> ()
              }
            }
            n577 = property on="Start Heat Up Test" class="Bool (strict)"("Visible"=FALSE) -> ()  [unwired: 2 in, 2 out]
            n578 = call <vilib>:"Add State(s) to Queue__jki_lib_state_machine.vi"("State(s) in (\"\")"=w1310) -> ("States Out"=w1309:string)  [unwired: 14 in]
          }
          event Value Change {
            # "Exit Button Value Change (pressed) Event\n(this executes Macro: Exit to terminate the VI)"
            n579 = event-data() -> ()  [unwired: 1 in, 6 out]
            n580 = call <vilib>:"Add State(s) to Queue__jki_lib_state_machine.vi"("State(s) in Front (\"\")"="Exit", "State(s) in (\"\")"=w1323) -> ("States Out"=w1322:string)  [unwired: 13 in]
          }
        }
      }
      frame "---------- Core ----------" {
        # "Do not put any code in this frame.\n(it is a separator no-op)"
        n581 = call <vilib>:"Add State(s) to Queue__jki_lib_state_machine.vi"("State(s) in (\"\")"=w1327) -> ("States Out"=w1326:string)  [unwired: 14 in]
      }
      frame Default {
        w1337 = 42 items=["No error", "Argument error", "Memory is full", "Out of zone", "End of file", "File already open", "Generic file I/O error", "File not found", "File permission error", "Disk is full", "Duplicate path", "Too many files open", "System feature not enabled", "Resource file not found", "Cannot add resource", "Resource not found", "Image not found", "Image memory error", "Pen does not exist", "Config type invalid", "Config token not found", "Config parse error", "Config memory error", "Bad external code format", "Bad external code offset", "External code not present", "Null window", "Destroy window error", "Null menu", "Print aborted", "Bad print record", "Print driver error", "Windows error during printing", "Memory error during printing", "Print dialog error", "Generic print error", "Invalid device refnum", "Device not found", "Device parameter error", "Device unit error", "Cannot open device", "Device call aborted", "Generic error", "Cancelled by user", "Object ID too low", "Object ID too high", "Object not in heap", "Unknown heap", "Unknown object (invalid DefProc)", "Unknown object (DefProc not in table)", "Message out of range", "Invalid (null) method", "Unknown message", "Manager call not supported", "Bad address", "Network operation in progress", "Network operation timed out", "Connection is busy", "Network attribute not supported", "Network error", "Address in use", "System out of memory", "Connection aborted", "Connection refused", "Not connected", "Already connected", "Connection closed", "Initialization error (interapplication manager)", "Bad occurrence", "Wait on unbound occurrence handler", "Occurrence queue overflow", "Datalog type conflict", "Unused", "Unrecognized type (interapplication manager)", "Memory corrupt", "Failed to make temporary DLL", "Old CIN version", "Drag socket not found", "Failed to load drop-object", "Failed to register OLE object", "Failed to release OLE object", "Format specifier type mismatch", "Unknown format specifier", "Too few format specifiers", "Too many format specifiers", "Scan failed", "Newer CIN version", "Error converting to variant", "Runtime menu error", "Password tampered", "Variant attribute not found", "Incompatible variant data type", "Event data is not available", "Event Store is not present", "Occurrence is not found", "Event Queue is not created", "Event info is not available", "Refnum passed is NULL", "Error retrieving Class GUID", "Error retrieving CoClass GUID", "Error retrieving TypeLib GUID.", "Bad built application magic bytes.", "Specific driver is different from the specific driver associated with the Logical Name.", "There is no session opened to the class driver.", "Max Error", "MAX - Error with config objects", "MAX - Error loading configuration", "MAX - Group not supported"]
        # "Current State"
        # "Do not delete, rename, or modify this frame.\n(this is used to capture unhandled states and typos)"
        # "Handle mistyped state name (developer tool)"
        n582 = Format Into String(format string="Software Exception: Unhandled State \"%s\"." ("message"), error in=w1333, w1328) -> (resulting string=w1336:string, error out=w1335:errorcluster)  [unwired: 1 in]
        n583 = call <vilib>:"Error Cluster From Error Code.vi"("show call chain? (False)"=TRUE, "error in (no error)"=w1335, "error message (\"\")"=w1336, "error code (0)"=w1337) -> ("error out"=w1334:errorcluster)  [unwired: 5 in]
        n584 = call <vilib>:"Add State(s) to Queue__jki_lib_state_machine.vi"("State(s) in (\"\")"=w1332) -> ("States Out"=w1331:string)  [unwired: 14 in]
      }
      frame "Error Handler" {
        # "Unhandled Error -- Display it"
        # "Handle any errors here.\nYou can also output any states to clean-up after errors occur"
        # "Clear error"
        n585 = call <vilib>:"General Error Handler.vi"("error in (no error)"=w1340) -> ()  [unwired: 10 in, 5 out]
        n586 = call <vilib>:"Add State(s) to Queue__jki_lib_state_machine.vi"("State(s) in Front (\"\")"="/* Post Error States", "State(s) in (\"\")"=w1344) -> ("States Out"=w1343:string)  [unwired: 13 in]
      }
      frame "Exit" {
        # "Do not put any code in this frame.\n(No errors that occur here will be handled.)"
        n587 = call <vilib>:"Add State(s) to Queue__jki_lib_state_machine.vi"("State(s) in (\"\")"=w1349) -> ("States Out"=w1348:string)  [unwired: 14 in]
      }
      frame "---------- Data ----------" {
        # "Do not put any code in this frame.\n(It is a separator no-op. You can make a copy of this frame to create a new Data frame)"
        n588 = call <vilib>:"Add State(s) to Queue__jki_lib_state_machine.vi"("State(s) in (\"\")"=w1353) -> ("States Out"=w1352:string)  [unwired: 14 in]
      }
      frame "Data: Initialize" {
        # "Initialize the shift-register data, here.\n(data names are defined by what you wire into the bundle function)"
        n589 = while {
          tunnel: [w1363] -> w1354
          stop <- w1360 stop-if-true
          w1363 = ""  # Unit Type
          n590 = call "UTILITY Boolean Notifier.vi"("Status"=UTILITY_Notifier."Read", "Set Status"=FALSE, "name (unnamed)"="Start UI Loop") -> ("latest READ notification"=w1360:bool)  [unwired: 7 in, 1 out]
          n591 = Wait Until Next ms Multiple(millisecond multiple=u32 250) -> ()  [unwired: 1 out]
        }
        n592 = Bundle("Unit Type"=w1354) -> (w1356:cluster{"Unit Type":string})  [unwired: 1 in]
        n593 = call <vilib>:"Add State(s) to Queue__jki_lib_state_machine.vi"("State(s) in (\"\")"=w1358) -> ("States Out"=w1357:string)  [unwired: 14 in]
      }
      frame "---------- Macro ----------" {
        # "Do not put any code in this frame.\n(It is a separator no-op. You can make a copy of this frame to create a new Macro frame)"
        n594 = call <vilib>:"Add State(s) to Queue__jki_lib_state_machine.vi"("State(s) in (\"\")"=w1368) -> ("States Out"=w1367:string)  [unwired: 14 in]
      }
      frame "Macro: Initialize" {
        # "Initialization Macro\n(This is called once, when the VI starts)"
        n595 = call <vilib>:"Add State(s) to Queue__jki_lib_state_machine.vi"("State(s) in Front (\"\")"="Data: Initialize", "State(s) in (\"\")"=w1373) -> ("States Out"=w1372:string)  [unwired: 13 in]
      }
      frame "---------- Heat Up Test ----------" {
        n596 = call <vilib>:"Add State(s) to Queue__jki_lib_state_machine.vi"("State(s) in (\"\")"=w1377) -> ("States Out"=w1376:string)  [unwired: 14 in]
      }
      frame "Set Mode" {
        n597 = flat-sequence {
          tunnel: w1381 -> [w1386]
          tunnel: [w1385] -> w1379
          tunnel: [w1388] -> w1380
          tunnel: w1379 -> [w1388]
          tunnel: ["Full Cutout"] -> w1378
          frame #0 {
            n598 = call "HEWH Set Mode.vi"("error in (no error)"=w1386) -> ("error out"=w1385:errorcluster)  [unwired: 10 in]
          }
          frame #1 {
          }
        }
        n599 = call <vilib>:"Add State(s) to Queue__jki_lib_state_machine.vi"("State(s) in Front (\"\")"=w1378, "State(s) in (\"\")"=w1384) -> ("States Out"=w1383:string)  [unwired: 13 in]
      }
      frame "Full Cutout" {
        # "Wait for stabilization.  Checks heat sources every second.  \nIf the heat sources are both off, the water heater is stabilized. \nFor StdElect. Looks at the heating element.  For other heating\nmodes, looks at the RS232 feedback on fans and compressor."
        n600 = while {
          tunnel: [w1397] -> w1390
          stop <- w1397 stop-if-true
          n601 = local read "Full Cutout"() -> (w1397:bool)
          n602 = local write "Message"(T23 "Waiting for Full Cutout...." ("Message")) -> ()
          n603 = Wait Until Next ms Multiple(millisecond multiple=u32 500) -> ()  [unwired: 1 out]
        }
        n604 = case shown="True" w1390 {
          tunnel: ["" "Step 1"] -> w1389
          frame False {
          }
          frame True {
            n605 = local write "Start Draw Timer"(TRUE ("Start Draw Timer")) -> ()
          }
        }
        n606 = call <vilib>:"Add State(s) to Queue__jki_lib_state_machine.vi"("State(s) in Front (\"\")"=w1389, "State(s) in (\"\")"=w1394) -> ("States Out"=w1393:string)  [unwired: 13 in]
      }
      frame "Step 1" {
        # "1.\tAfter unit has been stable for 30+/-5 minutes, \nOpen valve, and draw 10.75 +/- .25 gallons of\n water at a rate of 3+/-.25 gpm"
        n607 = flat-sequence {
          tunnel: w1407 -> [w1412]
          tunnel: [w1411] -> w1406
          tunnel: [w1410] -> w1404
          tunnel: [w1426] -> w1403
          tunnel: w1406 -> [w1426]
          tunnel: [w1425] -> w1405
          tunnel: w1404 -> [w1424]
          tunnel: w1401 -> [w1423]
          frame #0 {
            n608 = while {
              shift-right: [w1418] -> w1411
              shift-left: w1412 -> [w1418]
              tunnel: [w1413] -> w1410
              stop <- w1414 stop-if-true
              n609 = local read "Shutdown Sequence"() -> (w1417:string)
              n610 = local read "Draw Time"() -> (w1422:T20)
              n611 = Greater?(x=w1422, y="Step 1 Wait Time") -> (0:w1415:bool)
              n612 = Equal?(x=w1417, y="Exit" ("State(s) in Front (\"\")")) -> (x = y?=w1413:bool)
              n613 = Or(x=w1413, y=w1415) -> (x .or. y?=w1414:bool)
              n614 = local write "Message"(T23 "Step 1: Stabilizing for 30 Min...." ("Message")) -> ()
              n615 = Wait Until Next ms Multiple(millisecond multiple=u32 500) -> ()  [unwired: 1 out]
            }
          }
          frame #1 {
            n616 = case shown="False" w1424 {
              tunnel: [w1430 "Exit" ("State(s) in Front (\"\")")] -> w1425
              tunnel: w1423 -> [w1427 _]
              frame False {
                n617 = local write "Gallon Target"("Step 1A Gallon Target") -> ()
                n618 = local write "GPM Target"("Heat Up GPM Target") -> ()
                n619 = local write "Temperature"("Heat Up Temperature") -> ()
                n620 = local write "Shutdown"("Set Temp\nAdjust Temp\nDispense Gallons" ("State(s) in Front (\"\")")) -> ()
                n621 = case shown="\"50 Gallon\", Default" w1427 {
                  tunnel: ["Step 2" "Step 1A"] -> w1430
                  frame "50 Gallon", Default {
                  }
                  frame "80 Gallon" {
                  }
                }
              }
              frame True {
              }
            }
          }
        }
        n622 = Unbundle By Name(w1402) -> ("Unit Type"=w1401:string)
        n623 = call <vilib>:"Add State(s) to Queue__jki_lib_state_machine.vi"("State(s) in Front (\"\")"=w1405, "State(s) in (\"\")"=w1409) -> ("States Out"=w1408:string)  [unwired: 13 in]
      }
      frame "Step 1A" {
        # "2.\t80 Gallon Only. Wait for 1 hour after\ndraw start. \n3.\tDraw another 10.75 gallons."
        n624 = flat-sequence {
          tunnel: w1436 -> [w1460]
          tunnel: [w1459] -> w1442
          tunnel: [w1458] -> w1440
          tunnel: [w1475] -> w1439
          tunnel: w1442 -> [w1475]
          tunnel: [w1474] -> w1441
          tunnel: w1440 -> [w1473]
          frame #0 {
            n625 = while {
              shift-right: [w1468] -> w1459
              shift-left: w1460 -> [w1468]
              tunnel: [w1464] -> w1458
              i -> [w1462]
              stop <- w1465 stop-if-true
              n626 = local read "Shutdown Sequence"() -> (w1467:string)
              n627 = Wait Until Next ms Multiple(millisecond multiple=u32 1000) -> ()  [unwired: 1 out]
              n628 = Greater?(x=w1462, y=3600) -> (0:w1461:bool)
              n629 = Equal?(x=w1467, y="Exit" ("State(s) in Front (\"\")")) -> (x = y?=w1464:bool)
              n630 = local write "Message"(T23 "Step 1A: Stabilizing for 1 Hour...." ("Message")) -> ()
              n631 = Or(x=w1464, y=w1461) -> (x .or. y?=w1465:bool)
            }
          }
          frame #1 {
            # "If using GEA2, draw until\nsmall draw flag. The 15 is a \ndummy value"
            n632 = case shown="False" w1473 {
              tunnel: ["Step 2" "Exit" ("State(s) in Front (\"\")")] -> w1474
              frame False {
                n633 = local read "Heat Up Temperature"() -> (w1479:T19)
                n634 = local read "Heat Up GPM Target"() -> (w1478:T19)
                n635 = local write "Shutdown"("Set Temp\nAdjust Temp\nDispense Gallons" ("State(s) in Front (\"\")")) -> ()
                n636 = local write "GPM Target"(w1478) -> ()
                n637 = local write "Temperature"(w1479) -> ()
              }
              frame True {
              }
            }
            n638 = local read "Trigger With GEA2"() -> (w1471:bool)
            n639 = case shown="True" w1471 {
              tunnel: [w1476 T19 10.75 ("Step 1A Gallon Target")] -> w1472
              frame False {
                n640 = local read "Step 1A Gallon Target"() -> (w1476:T19)
              }
              frame True {
              }
            }
            n641 = local write "Gallon Target"(w1472) -> ()
          }
        }
        n642 = while {
          tunnel: w1437 -> [w1456]
          tunnel: [w1456] -> w1436
          i -> [w1450]
          stop <- w1446 stop-if-true
          n643 = local read "Start Draw Routine"() -> (w1457:bool)
          n644 = local read "Shutdown Sequence"() -> (w1454:string)
          n645 = call "HEWH Draw Routing Start.vi"("Start Draw Routine"=w1457) -> ("Start Draw Routine Output"=w1451:bool)  [unwired: 10 in]
          n646 = Equal?(x=w1454, y="Exit" ("State(s) in Front (\"\")")) -> (x = y?=w1452:bool)
          n647 = Compound Arithmetic op=OR(w1452, invert w1451) -> (w1447:bool)
          n648 = Greater?(x=w1450, y=8) -> (0:w1448:bool)
          n649 = local write "Message"(T23 "Step 1A: Waiting for First Draw to Complete...." ("Message")) -> ()
          n650 = And(x=w1447, y=w1448) -> (x .and. y?=w1446:bool)
          n651 = Wait Until Next ms Multiple(millisecond multiple=u32 1000) -> ()  [unwired: 1 out]
        }
        n652 = call <vilib>:"Add State(s) to Queue__jki_lib_state_machine.vi"("State(s) in Front (\"\")"=w1441, "State(s) in (\"\")"=w1444) -> ("States Out"=w1443:string)  [unwired: 13 in]
      }
      frame "Step 2" {
        # "If the lower heat source come on at exactly 10.72 gal\nthan this program could get \"stuck\"..it does not initialize the \ndraw sequence again...fix this. Solution: Increased draw amount\non GEA2 version to 11.5 since it triggers from the flag"
        # "If GEA2, trigger with\nsmall draw event flag"
        # "4.\tIf lower heat source energizes (Hybrid Mode/Heat Pump Mode = FAN ON\n follow by Compressor, Standard Electric Mode = Lower Element ON) before\n 10.75 gallons, then continue drawing water until Upper element engages as \nshown in step 5 (skip to step 5)."
        n653 = flat-sequence {
          tunnel: [w1499] -> w1492
          tunnel: [w1498] -> w1491
          tunnel: w1488 -> [w1497]
          tunnel: [w1497] -> w1490
          tunnel: w1483 -> [w1496]
          tunnel: [w1531] -> w1493
          tunnel: w1492 -> [w1530]
          tunnel: w1491 -> [w1529]
          tunnel: w1490 -> [w1528]
          tunnel: [w1528] -> w1489
          frame #0 {
            # "Wait for a complete\ndraw"
            n654 = while {
              tunnel: [w1511] -> w1499
              tunnel: [w1510] -> w1498
              tunnel: w1496 -> [w1502]
              i -> [w1507]
              stop <- w1503 stop-if-true
              n655 = local read "Start Draw Routine"() -> (w1509:bool)
              n656 = local read "Trigger With GEA2"() -> (w1501:bool)
              n657 = case shown="False" w1501 {
                tunnel: [w1518 w1526] -> w1510
                tunnel: w1502 -> [w1516 _]
                tunnel: [T23 "Step 2: Drawing 10.72 Gal...." ("Message") T23 "Step 2: Drawing until Small Draw Flag...." ("Message")] -> w1500
                frame False {
                  # "If an element turns on"
                  n658 = local read "Gallons"() -> (w1517:T19)
                  n659 = local read "Full Cutout"() -> (w1522:bool)
                  n660 = Less Or Equal?(x=w1517, y=w1516) -> (x <= y?=w1520:bool)
                  n661 = Equal?(x=w1522, y=FALSE) -> (x = y?=w1519:bool)
                  n662 = And(x=w1520, y=w1519) -> (x .and. y?=w1518:bool)
                }
                frame True {
                  n663 = local read "Water Heater GEA2 Data"() -> (w1527:T36)
                  n664 = Unbundle By Name(w1527) -> ("Hyperterminal Data.Flow Events (Bit Encoded)"=w1525:u16)
                  n665 = Equal?(x=w1525, y=u16 1) -> (x = y?=w1526:bool)
                }
              }
              n666 = local read "Shutdown Sequence"() -> (w1513:string)
              n667 = Equal?(x=w1513, y="Exit" ("State(s) in Front (\"\")")) -> (x = y?=w1511:bool)
              n668 = call "HEWH Draw Routing Start.vi"("Start Draw Routine"=w1509) -> ("Start Draw Routine Output"=w1508:bool)  [unwired: 10 in]
              n669 = Compound Arithmetic op=OR(w1511, invert w1508, w1510) -> (w1505:bool)
              n670 = local write "Message"(w1500) -> ()
              n671 = Wait Until Next ms Multiple(millisecond multiple=u32 1000) -> ()  [unwired: 1 out]
              n672 = Greater?(x=w1507, y=8) -> (0:w1504:bool)
              n673 = And(x=w1505, y=w1504) -> (x .and. y?=w1503:bool)
            }
          }
          frame #1 {
            n674 = case shown="False" w1530 {
              tunnel: w1529 -> [w1533 _]
              tunnel: [w1532 "Exit" ("State(s) in Front (\"\")")] -> w1531
              frame False {
                n675 = case shown="False" w1533 {
                  tunnel: ["Step 3" "Step 5"] -> w1532
                  frame False {
                  }
                  frame True {
                    n676 = local write "Gallon Target"(T19 100.0 ("Gallon Target")) -> ()
                  }
                }
              }
              frame True {
              }
            }
          }
        }
        n677 = local read "Step 1A Gallon Target"() -> (w1486:T19)
        n678 = Unbundle By Name(w1487) -> ("Unit Type"=w1485:string)
        n679 = call "HEWH Gallon Target.vi"("Step 2 Gallon Target"="Step 2 Gallon Target", "Unit Type"=w1485, "Step 1A Gallon Target"=w1486) -> ("Gallon Target"=w1483:dbl)  [unwired: 8 in]
        n680 = call <vilib>:"Add State(s) to Queue__jki_lib_state_machine.vi"("State(s) in Front (\"\")"=w1493, "State(s) in (\"\")"=w1495) -> ("States Out"=w1494:string)  [unwired: 13 in]
      }
      frame "Step 3" {
        # "5.\tIf lower heat source does not energize during 10.75 gallon draw, then wait a maximum of 10 minutes to see if lower heat source will energize (If it does not energize, it is considered a failure).  If it does, then allow the water heater to recover to set point."
        n681 = while {
          tunnel: [w1564] -> w1540
          tunnel: [w1559] -> w1538
          i -> [w1566]
          stop <- w1560 stop-if-true
          # "The fan is not a heat \nsource"
          n682 = local read "Shutdown Sequence"() -> (w1563:string)
          n683 = local read "POWER"() -> (w1569:T12)
          n684 = Greater?(x=w1566, y=600) -> (0:w1561:bool)
          n685 = Equal?(x=w1563, y="Exit" ("State(s) in Front (\"\")")) -> (x = y?=w1559:bool)
          n686 = local write "Message"(T23 "Step 3: Waiting 10 Min...." ("Message")) -> ()
          n687 = Unbundle By Name(w1569) -> ("LE"=w1568:bool, "COMP"=w1567:bool)
          n688 = Or(x=w1559, y=w1561) -> (x .or. y?=w1560:bool)
          n689 = Wait Until Next ms Multiple(millisecond multiple=u32 1000) -> ()  [unwired: 1 out]
          n690 = Compound Arithmetic op=OR(w1568, w1567) -> (w1564:bool)
        }
        n691 = case shown="False" w1538 {
          tunnel: w1540 -> [w1546 _]
          tunnel: [w1545 "Exit" ("State(s) in Front (\"\")")] -> w1539
          frame False {
            n692 = case shown="True" w1546 {
              tunnel: ["Step 4" w1548] -> w1545
              frame False {
              }
              frame True {
                n693 = while {
                  tunnel: ["Step 4"] -> w1548
                  i -> [w1553]
                  stop <- w1549 stop-if-true
                  n694 = local read "Full Cutout"() -> (w1550:bool)
                  n695 = Greater?(x=w1553, y=8) -> (0:w1551:bool)
                  n696 = local write "Message"(T23 "Step 3: Waiting for Full Cutout...." ("Message")) -> ()
                  n697 = And(x=w1551, y=w1550) -> (x .and. y?=w1549:bool)
                  n698 = Wait Until Next ms Multiple(millisecond multiple=u32 1000) -> ()  [unwired: 1 out]
                }
              }
            }
          }
          frame True {
          }
        }
        n699 = call <vilib>:"Add State(s) to Queue__jki_lib_state_machine.vi"("State(s) in Front (\"\")"=w1539, "State(s) in (\"\")"=w1544) -> ("States Out"=w1543:string)  [unwired: 13 in]
      }
      frame "Step 4" {
        # "Reset the flow meter and \nwatt meter when you start step 5"
        # "6.\tAllow unit to sit 5 to 10 minutes in stabilized conditions, then:\n7.\tOpen valve and draw water at 3+/-.25 gpm until the Upper \nElement energizes.  Water draw must stop within 5 seconds after\n Upper Element energizes.  NOTE: when running the unit in e-Heat\n mode, (no upper element) draw 40+/-0.25 gallons of water."
        n700 = flat-sequence {
          tunnel: [w1579] -> w1572
          tunnel: [w1578] -> w1571
          tunnel: [w1591] -> w1573
          tunnel: w1572 -> [w1590]
          tunnel: w1571 -> [w1592]
          frame #0 {
            n701 = while {
              tunnel: ["Step 5"] -> w1579
              tunnel: [w1581] -> w1578
              i -> [w1588]
              stop <- w1582 stop-if-true
              n702 = local read "Shutdown Sequence"() -> (w1585:string)
              n703 = Wait Until Next ms Multiple(millisecond multiple=u32 1000) -> ()  [unwired: 1 out]
              n704 = Greater?(x=w1588, y=300) -> (0:w1583:bool)
              "Heat Up Step 4 Flag" <- w1583
              n705 = Equal?(x=w1585, y="Exit" ("State(s) in Front (\"\")")) -> (x = y?=w1581:bool)
              n706 = local write "Message"(T23 "Step 4: Waiting 10 Min...." ("Message")) -> ()
              n707 = Or(x=w1581, y=w1583) -> (x .or. y?=w1582:bool)
            }
          }
          frame #1 {
            n708 = case shown="False" w1592 {
              tunnel: [w1595 "Exit" ("State(s) in Front (\"\")")] -> w1591
              tunnel: w1590 -> [w1595 _]
              frame False {
                # "Start drawing water for \nstep 5...adjust when you\nget the step 5"
                n709 = local read "Heat Up Temperature"() -> (w1594:T19)
                n710 = local read "Heat Up GPM Target"() -> (w1593:T19)
                n711 = local write "Gallon Target"(T19 100.0 ("Gallon Target")) -> ()
                n712 = local write "Shutdown"("Reset Totalizer\nSet Temp\nAdjust Temp\nDispense Gallons" ("State(s) in Front (\"\")")) -> ()
                n713 = local write "GPM Target"(w1593) -> ()
                n714 = local write "Temperature"(w1594) -> ()
              }
              frame True {
              }
            }
          }
        }
        n715 = call <vilib>:"Add State(s) to Queue__jki_lib_state_machine.vi"("State(s) in Front (\"\")"=w1573, "State(s) in (\"\")"=w1577) -> ("States Out"=w1576:string)  [unwired: 13 in]
      }
      frame "Step 5" {
        n716 = local read "Heat Up Step 4 Flag"() -> (w1606:bool)
        n717 = local read "Water Heater GEA2 Data"() -> (w1605:T36)
        n718 = Unbundle By Name(w1605) -> ("Hyperterminal Data.Heating Control Mode"=w1604:u16)
        n719 = case shown="True" w1606 {
          tunnel: w1604 -> [w1618 w1656]
          tunnel: w1603 -> [w1617 w1655]
          tunnel: [w1617 w1655] -> w1600
          tunnel: [w1616 w1654] -> w1602
          frame False {
            n720 = while {
              tunnel: w1618 -> [w1625]
              tunnel: [w1620] -> w1616
              i -> [w1619]
              stop <- w1621 stop-if-true
              n721 = case shown="3" w1625 {
                tunnel: [w1627 w1642] -> w1622
                tunnel: w1619 -> [_ w1641]
                frame 0, Default {
                  n722 = local read "Trigger With GEA2"() -> (w1629:bool)
                  n723 = case shown="False" w1629 {
                    tunnel: [w1630 w1634] -> w1627
                    frame False {
                      n724 = local read "POWER"() -> (w1631:T12)
                      n725 = Unbundle By Name(w1631) -> ("UE"=w1630:bool)
                    }
                    frame True {
                      # "Make sure large draw happens"
                      n726 = local read "Water Heater GEA2 Data"() -> (w1636:T36)
                      n727 = for {
                        N: 2 -> [_]
                        tunnel: [w1639] -> w1635
                        n728 = local read "POWER"() -> (w1640:T12)
                        n729 = Wait Until Next ms Multiple(millisecond multiple=u32 1000) -> ()  [unwired: 1 out]
                        n730 = Unbundle By Name(w1640) -> ("UE"=w1639:bool)
                      }
                      n731 = Unbundle By Name(w1636) -> ("Hyperterminal Data.Flow Events (Bit Encoded)"=w1633:u16)
                      n732 = call "HEWH Check Heating Control Mode.vi"("Flow Event"=w1633) -> ("Large Flag Detected"=w1632:bool)  [unwired: 10 in]
                      n733 = And(x=w1635, y=w1632) -> (x .and. y?=w1634:bool)
                    }
                  }
                  n734 = local write "Stop Custom Draw"(w1627) -> ()
                  n735 = local write "Message"(T23 "Step 5: Drawing Until UE & Large Flag...." ("Message")) -> ()
                }
                frame 3 {
                  n736 = Less?(x=w1641, y=1) -> (x < y?=w1644:bool)
                  n737 = case shown="False" w1644 {
                    tunnel: [w1646 w1648] -> w1642
                    frame False {
                      n738 = local read "Start Draw Routine"() -> (w1647:bool)
                      n739 = Not(x=w1647) -> (.not. x?=w1646:bool)
                    }
                    frame True {
                      n740 = while {
                        tunnel: [FALSE] -> w1648
                        i -> [w1652]
                        stop <- w1650 stop-if-true
                        # "Delay to insure\ndraw flag starts"
                        n741 = Greater?(x=w1652, y=30) -> (0:w1650:bool)
                        n742 = Wait Until Next ms Multiple(millisecond multiple=u32 1000) -> ()  [unwired: 1 out]
                      }
                    }
                  }
                  n743 = local write "Message"(T23 "Step 5: Drawing Water Until 40 Gal...." ("Message")) -> ()
                }
              }
              n744 = local read "Shutdown Sequence"() -> (w1624:string)
              n745 = Equal?(x=w1624, y="Exit" ("State(s) in Front (\"\")")) -> (x = y?=w1620:bool)
              n746 = Or(x=w1620, y=w1622) -> (x .or. y?=w1621:bool)
              n747 = Wait Until Next ms Multiple(millisecond multiple=u32 250) -> ()  [unwired: 1 out]
            }
          }
          frame True {
            n748 = while {
              tunnel: w1656 -> [w1663]
              tunnel: [w1658] -> w1654
              i -> [w1657]
              stop <- w1659 stop-if-true
              n749 = case shown="0, Default" w1663 {
                tunnel: [w1665 w1683] -> w1660
                tunnel: w1657 -> [_ w1680]
                frame 0, Default {
                  n750 = local read "Trigger With GEA2"() -> (w1667:bool)
                  n751 = case shown="True" w1667 {
                    tunnel: [w1668 w1670] -> w1665
                    frame False {
                      n752 = local read "POWER"() -> (w1669:T12)
                      n753 = Unbundle By Name(w1669) -> ("UE"=w1668:bool)
                    }
                    frame True {
                      # "Make sure large draw happens"
                      n754 = local read "Water Heater GEA2 Data"() -> (w1674:T36)
                      n755 = Unbundle By Name(w1674) -> ("Hyperterminal Data.Flow Events (Bit Encoded)"=w1673:u16)
                      n756 = for {
                        N: 2 -> [_]
                        tunnel: [w1677] -> w1672
                        n757 = local read "POWER"() -> (w1678:T12)
                        n758 = Wait Until Next ms Multiple(millisecond multiple=u32 1000) -> ()  [unwired: 1 out]
                        n759 = Unbundle By Name(w1678) -> ("UE"=w1677:bool)
                      }
                      n760 = call "HEWH Check Heating Control Mode.vi"("Flow Event"=w1673) -> ("Large Flag Detected"=w1671:bool)  [unwired: 10 in]
                      n761 = And(x=w1672, y=w1671) -> (x .and. y?=w1670:bool)
                    }
                  }
                  n762 = local write "Message"(T23 "Step 5: Drawing Until UE & Large Flag...." ("Message")) -> ()
                  n763 = local write "Stop Custom Draw"(w1665) -> ()
                }
                frame 3 {
                  n764 = Less?(x=w1680, y=1) -> (x < y?=w1681:bool)
                  n765 = case shown="False" w1681 {
                    tunnel: [w1684 w1686] -> w1683
                    frame False {
                      n766 = local read "Start Draw Routine"() -> (w1685:bool)
                      n767 = Not(x=w1685) -> (.not. x?=w1684:bool)
                    }
                    frame True {
                      n768 = while {
                        tunnel: [FALSE] -> w1686
                        i -> [w1690]
                        stop <- w1688 stop-if-true
                        # "Delay to insure\ndraw flag starts"
                        n769 = Greater?(x=w1690, y=30) -> (0:w1688:bool)
                        n770 = Wait Until Next ms Multiple(millisecond multiple=u32 1000) -> ()  [unwired: 1 out]
                      }
                    }
                  }
                  n771 = local write "Message"(T23 "Step 5: Drawing Water Until 40 Gal...." ("Message")) -> ()
                }
              }
              n772 = Wait Until Next ms Multiple(millisecond multiple=u32 250) -> ()  [unwired: 1 out]
              n773 = local read "Shutdown Sequence"() -> (w1662:string)
              n774 = Equal?(x=w1662, y="Exit" ("State(s) in Front (\"\")")) -> (x = y?=w1658:bool)
              n775 = Or(x=w1658, y=w1660) -> (x .or. y?=w1659:bool)
            }
          }
        }
        n776 = case shown="3" w1604 {
          frame 0, Default {
          }
          frame 3 {
            n777 = local write "Gallon Target"(T19 40.0 ("Gallon Target")) -> ()
          }
        }
        n778 = case shown="False" w1602 {
          tunnel: ["Step 6" "Exit" ("State(s) in Front (\"\")")] -> w1601
          tunnel: w1600 -> [w1611 w1613]
          tunnel: [w1611 w1613] -> w1599
          frame False {
            n779 = local write "Stop Custom Draw"(TRUE ("Stop Custom Draw")) -> ()
          }
          frame True {
          }
        }
        n780 = call <vilib>:"Add State(s) to Queue__jki_lib_state_machine.vi"("State(s) in Front (\"\")"=w1601, "State(s) in (\"\")"=w1609) -> ("States Out"=w1608:string)  [unwired: 13 in]
      }
      frame "Step 6" {
        # "Send a few time to\ninsure the HEWH gets\nthe message"
        # "8.\tIn Hybrid Mode: when the Upper Element stops and switches to Lower Element,\n switch the unit to Heat Pump Mode.  This will switch the lower heating source to \nCompressor."
        n781 = while {
          tunnel: w1699 -> [w1743]
          tunnel: [w1743] -> w1700
          tunnel: [w1740] -> w1697
          i -> [w1738]
          stop <- w1734 stop-if-true
          n782 = local read "Shutdown Sequence"() -> (w1742:string)
          n783 = Greater?(x=w1738, y=8) -> (0:w1735:bool)
          n784 = call "UTILITY Boolean Notifier.vi"("Status"=UTILITY_Notifier."Read", "name (unnamed)"="First Hour Cutout") -> ("latest READ notification"=w1731:bool)  [unwired: 8 in, 1 out]
          n785 = Equal?(x=w1742, y="Exit" ("State(s) in Front (\"\")")) -> (x = y?=w1740:bool)
          n786 = local write "Message"(T23 "Step 6: Waiting for UE Cutout...." ("Message")) -> ()
          n787 = Or(x=w1740, y=w1731) -> (x .or. y?=w1736:bool)
          n788 = And(x=w1736, y=w1735) -> (x .and. y?=w1734:bool)
          n789 = Wait Until Next ms Multiple(millisecond multiple=u32 1000) -> ()  [unwired: 1 out]
        }
        n790 = local read "Water Heater GEA2 Data"() -> (w1695:T36)
        n791 = Unbundle By Name(w1695) -> ("Hyperterminal Data.Heating Control Mode"=w1694:u16)
        n792 = Unbundle By Name(w1693) -> ("Unit Type"=w1692:string)
        n793 = case shown="1, 3, 4, Default" w1694 {
          tunnel: w1700 -> [w1706 w1716]
          tunnel: [w1706 w1715] -> w1698
          tunnel: w1697 -> [w1704 w1714]
          tunnel: [w1705 w1713] -> w1696
          tunnel: w1692 -> [w1703 w1712]
          frame 2 {
            n794 = case shown="False" w1704 {
              tunnel: [w1708 "Exit" ("State(s) in Front (\"\")")] -> w1705
              tunnel: w1703 -> [w1707 _]
              frame False {
                n795 = case shown="\"50 Gallon\", Default" w1707 {
                  tunnel: ["Step 7" "Step 6A"] -> w1708
                  frame "50 Gallon", Default {
                  }
                  frame "80 Gallon" {
                  }
                }
              }
              frame True {
              }
            }
          }
          frame 1, 3, 4, Default {
            n796 = case shown="False" w1714 {
              tunnel: w1716 -> [w1719 w1729]
              tunnel: [w1718 w1729] -> w1715
              tunnel: [w1721 "Exit" ("State(s) in Front (\"\")")] -> w1713
              tunnel: w1712 -> [w1720 _]
              frame False {
                n797 = for {
                  N: 3 -> [_]
                  tunnel: w1719 -> [w1724]
                  tunnel: [w1722] -> w1718
                  n798 = call "HEWH_DSM_CMD.vi"("Heating Mode"=GEA2_Commands_HEWH_Mode."eHeat" ("Mode"), "GEA2 Commands and Requests"=GEA2_Commands."CMD_UPDATE_MODE") -> ("Input Data"=w1723:T59)  [unwired: 7 in, 1 out]
                  n799 = call "Send Example.vi"("Input Data"=w1723, "Error In"=w1724) -> ("Error Out"=w1722:errorcluster)  [unwired: 13 in]
                }
                n800 = case shown="\"80 Gallon\"" w1720 {
                  tunnel: ["Step 7" "Step 6A"] -> w1721
                  frame "50 Gallon", Default {
                  }
                  frame "80 Gallon" {
                  }
                }
              }
              frame True {
              }
            }
          }
        }
        n801 = call <vilib>:"Add State(s) to Queue__jki_lib_state_machine.vi"("State(s) in Front (\"\")"=w1696, "State(s) in (\"\")"=w1702) -> ("States Out"=w1701:string)  [unwired: 13 in]
      }
      frame "Step 6A" {
        # "The 80 gallons have a 5 minute EEV stabilization to help protect against vapor lock"
        n802 = while {
          tunnel: w1749 -> [w1765]
          tunnel: [w1765] -> w1746
          tunnel: [w1757] -> w1748
          i -> [w1764]
          stop <- w1759 stop-if-true
          n803 = local read "Shutdown Sequence"() -> (w1762:string)
          n804 = Greater?(x=w1764, y=300) -> (0:w1760:bool)
          n805 = Equal?(x=w1762, y="Exit" ("State(s) in Front (\"\")")) -> (x = y?=w1757:bool)
          n806 = Or(x=w1757, y=w1760) -> (x .or. y?=w1759:bool)
          n807 = Wait Until Next ms Multiple(millisecond multiple=u32 1000) -> ()  [unwired: 1 out]
          n808 = local write "Message"(T23 "Step 6A Stabilizing EEV for 5 Min...." ("Message")) -> ()
        }
        n809 = case shown="False" w1748 {
          tunnel: ["Step 7" "Exit" ("State(s) in Front (\"\")")] -> w1747
          tunnel: w1746 -> [w1753 w1755]
          tunnel: [w1753 w1755] -> w1745
          frame False {
          }
          frame True {
          }
        }
        n810 = call <vilib>:"Add State(s) to Queue__jki_lib_state_machine.vi"("State(s) in Front (\"\")"=w1747, "State(s) in (\"\")"=w1752) -> ("States Out"=w1751:string)  [unwired: 13 in]
      }
      frame "Step 7" {
        # "9.\tAllow water heater to stabilize this second time.\n (Recover water temperature back to set point)."
        n811 = while {
          tunnel: w1771 -> [w1789]
          tunnel: [w1789] -> w1770
          tunnel: [w1785] -> w1768
          i -> [w1783]
          stop <- w1779 stop-if-true
          n812 = local read "Shutdown Sequence"() -> (w1788:string)
          n813 = local read "Full Cutout"() -> (w1786:bool)
          n814 = Equal?(x=w1788, y="Exit" ("State(s) in Front (\"\")")) -> (x = y?=w1785:bool)
          n815 = Greater?(x=w1783, y=8) -> (0:w1780:bool)
          n816 = Wait Until Next ms Multiple(millisecond multiple=u32 1000) -> ()  [unwired: 1 out]
          n817 = Or(x=w1785, y=w1786) -> (x .or. y?=w1781:bool)
          n818 = local write "Message"(T23 "Step 7: Waiting for Full Cutout...." ("Message")) -> ()
          n819 = And(x=w1781, y=w1780) -> (x .and. y?=w1779:bool)
        }
        n820 = case shown="False" w1768 {
          tunnel: w1770 -> [w1775 w1778]
          tunnel: [w1775 w1778] -> w1769
          tunnel: ["Step 8" "Exit" ("State(s) in Front (\"\")")] -> w1767
          frame False {
          }
          frame True {
          }
        }
        n821 = call <vilib>:"Add State(s) to Queue__jki_lib_state_machine.vi"("State(s) in Front (\"\")"=w1767, "State(s) in (\"\")"=w1774) -> ("States Out"=w1773:string)  [unwired: 13 in]
      }
      frame "Step 8" {
        # "11.\tStop Data Logger session. \n12.\tCapture all data into format shown in attached spreadsheet"
        # "10.\tAllow unit to sit a minimum of 30 minutes in stabilized conditions, then;"
        n822 = flat-sequence {
          tunnel: w1794 -> [w1799]
          tunnel: [w1798] -> w1792
          tunnel: [w1812] -> w1793
          tunnel: w1792 -> [w1812]
          tunnel: ["Exit"] -> w1791
          frame #0 {
            n823 = while {
              tunnel: w1799 -> [w1808]
              tunnel: [w1808] -> w1798
              i -> [w1807]
              stop <- w1801 stop-if-true
              n824 = local read "Shutdown Sequence"() -> (w1805:string)
              n825 = Greater?(x=w1807, y=1800) -> (0:w1802:bool)
              n826 = Equal?(x=w1805, y="Exit" ("State(s) in Front (\"\")")) -> (x = y?=w1803:bool)
              n827 = local write "Message"(T23 "Step 8: Waiting 30 Min...." ("Message")) -> ()
              n828 = Or(x=w1803, y=w1802) -> (x .or. y?=w1801:bool)
              n829 = Wait Until Next ms Multiple(millisecond multiple=u32 1000) -> ()  [unwired: 1 out]
            }
          }
          frame #1 {
            n830 = local write "Shutdown"("Add Headers" ("Shutdown")) -> ()
          }
        }
        n831 = call <vilib>:"Add State(s) to Queue__jki_lib_state_machine.vi"("State(s) in Front (\"\")"=w1791, "State(s) in (\"\")"=w1797) -> ("States Out"=w1796:string)  [unwired: 13 in]
      }
      frame "Check Exit" {
        n832 = local read "Shutdown Sequence"() -> (w1813:string)
        n833 = call <vilib>:"Add State(s) to Queue__jki_lib_state_machine.vi"("State(s) in Front (\"\")"=w1813, "State(s) in (\"\")"=w1817) -> ("States Out"=w1816:string)  [unwired: 13 in]
      }
    }
  }
  n834 = while "Write to File" {
    shift-right: [w1823] -> _
    shift-left: _ -> [w1822]
    shift-right: [w1826] -> w36
    shift-left: w38 -> [w1820]
    shift-right: [w1825] -> _
    shift-left: w39 -> [w1827]
    tunnel: w37 -> [w1819]
    tunnel: [w1818] -> w35
    stop <- w1824 stop-if-true
    w1821 = 1000  # Timeout
    # "Write To File"
    n835 = call <vilib>:"Parse State Queue__jki_lib_state_machine.vi"("State Queue"=w1827, "Error In (no error)"=w1820) -> ("Remaining States"=w1829:string, "Current State"=w1830:string, "Arguments"=w1828:string)  [unwired: 11 in]
    n836 = case shown="\"Write\"" w1830 {
      selector: w1830 -> [_ _ w1860 _ _ _ _ _ _ _ _ _]
      tunnel: w1829 -> [w1838 w1858 w1864 w1877 w1883 w1888 w1895 w1900 w1906 w1911 w1920 w1945]
      tunnel: w1828 -> [_ _ _ _ _ _ _ _ _ _ _ _]
      tunnel: w1822 -> [w1836 w1855 w1862 w1874 w1881 w1885 _ w1897 w1903 w1908 w1912 w1943]
      tunnel: [w1835 w1856 w1866 errorcluster {"status"=FALSE, "code"=0, "source"=""} ("error out") w1880 w1886 w1892 w1898 w1904 w1909 w1916 w1942] -> w1826
      tunnel: w1820 -> [w1834 w1856 w1865 w1873 w1880 w1886 w1892 w1898 w1904 w1909 w1917 w1942]
      tunnel: [w1837 w1857 w1863 w1876 w1882 w1887 w1894 w1899 w1905 w1910 w1919 w1944] -> w1825
      tunnel: [_ _ _ _ TRUE _ _ _ _ _ _ _] -> w1824
      tunnel: [w1833 w1855 w1862 w1874 w1881 w1885 w1893 w1897 w1903 w1908 w1912 w1943] -> w1823
      tunnel: w1821 -> [w1832 _ _ _ _ _ _ _ _ _ _ _]
      tunnel: w1819 -> [w1831 w1854 w1859 w1871 w1878 w1884 w1891 w1896 w1901 w1907 w1915 w1940]
      tunnel: [w1831 w1854 w1859 w1871 w1878 w1884 w1891 w1896 w1901 w1907 w1914 w1940] -> w1818
      frame "", "Idle" {
        n837 = event shown="[1] \"Data Table\": Value Change" {
          selector: _ -> [_ _ _]
          dyn-events: _ -> [_ _ _]
          timeout: w1832 -> [_ _ _]
          tunnel: w1838 -> [w1843 w1846 w1853]
          tunnel: [w1842 w1845 w1852] -> w1837
          tunnel: w1836 -> [w1841 w1848 w1850]
          tunnel: [w1840 w1847 w1851] -> w1835
          tunnel: w1834 -> [w1840 w1847 w1851]
          tunnel: [w1841 w1848 w1850] -> w1833
          event Timeout {
            n838 = event-data() -> ()  [unwired: 1 in, 1 out]
            n839 = call <vilib>:"Add State(s) to Queue__jki_lib_state_machine.vi"("State(s) in Front (\"\")"="Check Exit" ("State(s) in Front (\"\")"), "State(s) in (\"\")"=w1843) -> ("States Out"=w1842:string)  [unwired: 13 in]
          }
          event "Data Table": Value Change {
            n840 = event-data() -> ()  [unwired: 1 in, 6 out]
            n841 = call <vilib>:"Add State(s) to Queue__jki_lib_state_machine.vi"("State(s) in Front (\"\")"="Write" ("State(s) in Front (\"\")"), "State(s) in (\"\")"=w1846) -> ("States Out"=w1845:string)  [unwired: 13 in]
          }
          event Value Change {
            # "Exit Button Value Change (pressed) Event\n(this executes Macro: Exit to terminate the VI)"
            n842 = event-data() -> ()  [unwired: 1 in, 6 out]
            n843 = call <vilib>:"Add State(s) to Queue__jki_lib_state_machine.vi"("State(s) in Front (\"\")"="Exit", "State(s) in (\"\")"=w1853) -> ("States Out"=w1852:string)  [unwired: 13 in]
          }
        }
      }
      frame "---------- Core ----------" {
        # "Do not put any code in this frame.\n(it is a separator no-op)"
        n844 = call <vilib>:"Add State(s) to Queue__jki_lib_state_machine.vi"("State(s) in (\"\")"=w1858) -> ("States Out"=w1857:string)  [unwired: 14 in]
      }
      frame Default {
        w1869 = 42 items=["No error", "Argument error", "Memory is full", "Out of zone", "End of file", "File already open", "Generic file I/O error", "File not found", "File permission error", "Disk is full", "Duplicate path", "Too many files open", "System feature not enabled", "Resource file not found", "Cannot add resource", "Resource not found", "Image not found", "Image memory error", "Pen does not exist", "Config type invalid", "Config token not found", "Config parse error", "Config memory error", "Bad external code format", "Bad external code offset", "External code not present", "Null window", "Destroy window error", "Null menu", "Print aborted", "Bad print record", "Print driver error", "Windows error during printing", "Memory error during printing", "Print dialog error", "Generic print error", "Invalid device refnum", "Device not found", "Device parameter error", "Device unit error", "Cannot open device", "Device call aborted", "Generic error", "Cancelled by user", "Object ID too low", "Object ID too high", "Object not in heap", "Unknown heap", "Unknown object (invalid DefProc)", "Unknown object (DefProc not in table)", "Message out of range", "Invalid (null) method", "Unknown message", "Manager call not supported", "Bad address", "Network operation in progress", "Network operation timed out", "Connection is busy", "Network attribute not supported", "Network error", "Address in use", "System out of memory", "Connection aborted", "Connection refused", "Not connected", "Already connected", "Connection closed", "Initialization error (interapplication manager)", "Bad occurrence", "Wait on unbound occurrence handler", "Occurrence queue overflow", "Datalog type conflict", "Unused", "Unrecognized type (interapplication manager)", "Memory corrupt", "Failed to make temporary DLL", "Old CIN version", "Drag socket not found", "Failed to load drop-object", "Failed to register OLE object", "Failed to release OLE object", "Format specifier type mismatch", "Unknown format specifier", "Too few format specifiers", "Too many format specifiers", "Scan failed", "Newer CIN version", "Error converting to variant", "Runtime menu error", "Password tampered", "Variant attribute not found", "Incompatible variant data type", "Event data is not available", "Event Store is not present", "Occurrence is not found", "Event Queue is not created", "Event info is not available", "Refnum passed is NULL", "Error retrieving Class GUID", "Error retrieving CoClass GUID", "Error retrieving TypeLib GUID.", "Bad built application magic bytes.", "Specific driver is different from the specific driver associated with the Logical Name.", "There is no session opened to the class driver.", "Max Error", "MAX - Error with config objects", "MAX - Error loading configuration", "MAX - Group not supported"]
        # "Current State"
        # "Do not delete, rename, or modify this frame.\n(this is used to capture unhandled states and typos)"
        # "Handle mistyped state name (developer tool)"
        n845 = Format Into String(format string="Software Exception: Unhandled State \"%s\"." ("message"), error in=w1865, w1860) -> (resulting string=w1868:string, error out=w1867:errorcluster)  [unwired: 1 in]
        n846 = call <vilib>:"Error Cluster From Error Code.vi"("show call chain? (False)"=TRUE, "error in (no error)"=w1867, "error message (\"\")"=w1868, "error code (0)"=w1869) -> ("error out"=w1866:errorcluster)  [unwired: 5 in]
        n847 = call <vilib>:"Add State(s) to Queue__jki_lib_state_machine.vi"("State(s) in (\"\")"=w1864) -> ("States Out"=w1863:string)  [unwired: 14 in]
      }
      frame "Error Handler" {
        # "Unhandled Error -- Display it"
        # "Handle any errors here.\nYou can also output any states to clean-up after errors occur"
        # "Clear error"
        n848 = call <vilib>:"General Error Handler.vi"("error in (no error)"=w1873) -> ()  [unwired: 10 in, 5 out]
        n849 = call <vilib>:"Add State(s) to Queue__jki_lib_state_machine.vi"("State(s) in Front (\"\")"="/* Post Error States", "State(s) in (\"\")"=w1877) -> ("States Out"=w1876:string)  [unwired: 13 in]
      }
      frame "Exit" {
        # "Do not put any code in this frame.\n(No errors that occur here will be handled.)"
        n850 = call <vilib>:"Add State(s) to Queue__jki_lib_state_machine.vi"("State(s) in (\"\")"=w1883) -> ("States Out"=w1882:string)  [unwired: 14 in]
      }
      frame "---------- Data ----------" {
        # "Do not put any code in this frame.\n(It is a separator no-op. You can make a copy of this frame to create a new Data frame)"
        n851 = call <vilib>:"Add State(s) to Queue__jki_lib_state_machine.vi"("State(s) in (\"\")"=w1888) -> ("States Out"=w1887:string)  [unwired: 14 in]
      }
      frame "Data: Initialize" {
        w1889 = TRUE  # Place Holder
        n852 = Bundle("Place Holder"=w1889) -> (w1893:cluster{"Place Holder":bool})  [unwired: 1 in]
        n853 = call <vilib>:"Add State(s) to Queue__jki_lib_state_machine.vi"("State(s) in (\"\")"=w1895) -> ("States Out"=w1894:string)  [unwired: 14 in]
        "Start Value Signal Data Table" <- FALSE ("First Time Through?")
      }
      frame "---------- Macro ----------" {
        # "Do not put any code in this frame.\n(It is a separator no-op. You can make a copy of this frame to create a new Macro frame)"
        n854 = call <vilib>:"Add State(s) to Queue__jki_lib_state_machine.vi"("State(s) in (\"\")"=w1900) -> ("States Out"=w1899:string)  [unwired: 14 in]
      }
      frame "Macro: Initialize" {
        # "Initialization Macro\n(This is called once, when the VI starts)"
        n855 = call <vilib>:"Add State(s) to Queue__jki_lib_state_machine.vi"("State(s) in Front (\"\")"="Data: Initialize", "State(s) in (\"\")"=w1906) -> ("States Out"=w1905:string)  [unwired: 13 in]
      }
      frame "---------- Write To File ----------" {
        n856 = call <vilib>:"Add State(s) to Queue__jki_lib_state_machine.vi"("State(s) in (\"\")"=w1911) -> ("States Out"=w1910:string)  [unwired: 14 in]
      }
      frame "Write" {
        n857 = local read "Data Table"() -> (w1918:string[][])
        n858 = First Call?() -> (First Call?: T/F=w1913:bool)
        n859 = case shown="True" w1913 {
          tunnel: w1918 -> [w1927 w1937]
          tunnel: w1915 -> [w1925 w1935]
          tunnel: w1917 -> [w1923 w1929]
          tunnel: [w1922 w1928] -> w1916
          tunnel: [w1921 w1933] -> w1914
          frame False {
            # "Only save the data (no header)"
            n860 = Delete From Array(array=w1927, index (col)=1 ("index (row)")) -> (deleted portion=w1924:string[])  [unwired: 2 in, 1 out]
            n861 = call "Write CSV File.vi"("Refnum In"=w1925, "Data"=w1924, "Error In"=w1923) -> ("Refnum Out"=w1921:refnum<file>, "Error Out"=w1922:errorcluster)  [unwired: 11 in]
          }
          frame True {
            # "Save the label and data the \nfirst time through"
            n862 = Delete From Array(array=w1937, index (col)=1 ("disabled index (col)")) -> (deleted portion=w1930:string[])  [unwired: 2 in, 1 out]
            n863 = Delete From Array(array=w1937, index (col)=0 ("index (row)")) -> (deleted portion=w1932:string[])  [unwired: 2 in, 1 out]
            n864 = call "Write CSV File.vi"("Refnum In"=w1935, "Data"=w1932, "Error In"=w1929) -> ("Refnum Out"=w1934:refnum<file>, "Error Out"=w1931:errorcluster)  [unwired: 11 in]
            n865 = call "Write CSV File.vi"("Refnum In"=w1934, "Data"=w1930, "Error In"=w1931) -> ("Refnum Out"=w1933:refnum<file>, "Error Out"=w1928:errorcluster)  [unwired: 11 in]
          }
        }
        n866 = call <vilib>:"Add State(s) to Queue__jki_lib_state_machine.vi"("State(s) in (\"\")"=w1920) -> ("States Out"=w1919:string)  [unwired: 14 in]
      }
      frame "Check Exit" {
        n867 = local read "Shutdown Sequence"() -> (w1941:string)
        n868 = local write "Start Value Signal Data Table"(TRUE ("Start Value Signal Data Table")) -> ()
        n869 = call <vilib>:"Add State(s) to Queue__jki_lib_state_machine.vi"("State(s) in Front (\"\")"=w1941, "State(s) in (\"\")"=w1945) -> ("States Out"=w1944:string)  [unwired: 13 in]
      }
    }
  }
  n870 = while "Check Heating Status" {
    shift-right: [w1949] -> _
    shift-left: _ -> [w1948]
    shift-right: [w1952] -> _
    shift-left: _ -> [w1946]
    shift-right: [w1951] -> _
    shift-left: w42 -> [w1953]
    stop <- w1950 stop-if-true
    w1947 = 1000  # Timeout
    # "Check Heating Status"
    n871 = call <vilib>:"Parse State Queue__jki_lib_state_machine.vi"("State Queue"=w1953, "Error In (no error)"=w1946) -> ("Remaining States"=w1955:string, "Current State"=w1956:string, "Arguments"=w1954:string)  [unwired: 11 in]
    n872 = case shown="\"Full Cutout\"" w1956 {
      selector: w1956 -> [_ _ w1981 _ _ _ _ _ _ _ _ _ _]
      tunnel: w1955 -> [w1963 w1980 w1985 w1997 w2002 w2006 w2011 w2021 w2026 w2030 w2038 w2088 w2120]
      tunnel: w1954 -> [_ _ _ _ _ _ _ _ _ _ _ _ _]
      tunnel: w1948 -> [w1961 w1977 w1983 w1994 w2000 w2003 _ w2018 w2023 w2027 w2035 w2085 w2117]
      tunnel: [w1960 w1978 w1987 errorcluster {"status"=FALSE, "code"=0, "source"=""} ("error out") w1999 w2004 w2008 w2019 w2024 w2028 w2036 w2086 w2118] -> w1952
      tunnel: w1946 -> [w1959 w1978 w1986 w1993 w1999 w2004 w2008 w2019 w2024 w2028 w2036 w2086 w2118]
      tunnel: [w1962 w1979 w1984 w1996 w2001 w2005 w2010 w2020 w2025 w2029 w2037 w2087 w2119] -> w1951
      tunnel: [_ _ _ _ TRUE _ _ _ _ _ _ _ _] -> w1950
      tunnel: [w1958 w1977 w1983 w1994 w2000 w2003 w2009 w2018 w2023 w2027 w2035 w2085 w2117] -> w1949
      tunnel: w1947 -> [w1957 _ _ _ _ _ _ _ _ _ _ _ _]
      frame "", "Idle" {
        n873 = event shown="[0] Timeout" {
          selector: _ -> [_ _]
          dyn-events: _ -> [_ _]
          timeout: w1957 -> [_ _]
          tunnel: w1963 -> [w1969 w1974]
          tunnel: [w1968 w1972] -> w1962
          tunnel: w1961 -> [w1966 w1976]
          tunnel: [w1967 w1975] -> w1960
          tunnel: w1959 -> [w1967 w1975]
          tunnel: [w1966 w1976] -> w1958
          event Timeout {
            n874 = event-data() -> ()  [unwired: 1 in, 1 out]
            n875 = local read item#-1() -> (w1964)
            n876 = case shown="False" w1964 {
              tunnel: ["First Hour Check Status\nFull Cutout\nCheck for Exit" ("State(s) in Front (\"\")") "" ("State(s) in Front (\"\")")] -> w1965
              frame False {
              }
              frame True {
              }
            }
            n877 = call <vilib>:"Add State(s) to Queue__jki_lib_state_machine.vi"("State(s) in Front (\"\")"=w1965, "State(s) in (\"\")"=w1969) -> ("States Out"=w1968:string)  [unwired: 13 in]
          }
          event Value Change {
            n878 = event-data() -> ()  [unwired: 1 in, 6 out]
            n879 = call <vilib>:"Add State(s) to Queue__jki_lib_state_machine.vi"("State(s) in Front (\"\")"="Exit" ("State(s) in Front (\"\")"), "State(s) in (\"\")"=w1974) -> ("States Out"=w1972:string)  [unwired: 13 in]
          }
        }
      }
      frame "---------- Core ----------" {
        # "Do not put any code in this frame.\n(it is a separator no-op)"
        n880 = call <vilib>:"Add State(s) to Queue__jki_lib_state_machine.vi"("State(s) in (\"\")"=w1980) -> ("States Out"=w1979:string)  [unwired: 14 in]
      }
      frame Default {
        w1990 = 42 items=["No error", "Argument error", "Memory is full", "Out of zone", "End of file", "File already open", "Generic file I/O error", "File not found", "File permission error", "Disk is full", "Duplicate path", "Too many files open", "System feature not enabled", "Resource file not found", "Cannot add resource", "Resource not found", "Image not found", "Image memory error", "Pen does not exist", "Config type invalid", "Config token not found", "Config parse error", "Config memory error", "Bad external code format", "Bad external code offset", "External code not present", "Null window", "Destroy window error", "Null menu", "Print aborted", "Bad print record", "Print driver error", "Windows error during printing", "Memory error during printing", "Print dialog error", "Generic print error", "Invalid device refnum", "Device not found", "Device parameter error", "Device unit error", "Cannot open device", "Device call aborted", "Generic error", "Cancelled by user", "Object ID too low", "Object ID too high", "Object not in heap", "Unknown heap", "Unknown object (invalid DefProc)", "Unknown object (DefProc not in table)", "Message out of range", "Invalid (null) method", "Unknown message", "Manager call not supported", "Bad address", "Network operation in progress", "Network operation timed out", "Connection is busy", "Network attribute not supported", "Network error", "Address in use", "System out of memory", "Connection aborted", "Connection refused", "Not connected", "Already connected", "Connection closed", "Initialization error (interapplication manager)", "Bad occurrence", "Wait on unbound occurrence handler", "Occurrence queue overflow", "Datalog type conflict", "Unused", "Unrecognized type (interapplication manager)", "Memory corrupt", "Failed to make temporary DLL", "Old CIN version", "Drag socket not found", "Failed to load drop-object", "Failed to register OLE object", "Failed to release OLE object", "Format specifier type mismatch", "Unknown format specifier", "Too few format specifiers", "Too many format specifiers", "Scan failed", "Newer CIN version", "Error converting to variant", "Runtime menu error", "Password tampered", "Variant attribute not found", "Incompatible variant data type", "Event data is not available", "Event Store is not present", "Occurrence is not found", "Event Queue is not created", "Event info is not available", "Refnum passed is NULL", "Error retrieving Class GUID", "Error retrieving CoClass GUID", "Error retrieving TypeLib GUID.", "Bad built application magic bytes.", "Specific driver is different from the specific driver associated with the Logical Name.", "There is no session opened to the class driver.", "Max Error", "MAX - Error with config objects", "MAX - Error loading configuration", "MAX - Group not supported"]
        # "Current State"
        # "Do not delete, rename, or modify this frame.\n(this is used to capture unhandled states and typos)"
        # "Handle mistyped state name (developer tool)"
        n881 = Format Into String(format string="Software Exception: Unhandled State \"%s\"." ("message"), error in=w1986, w1981) -> (resulting string=w1989:string, error out=w1988:errorcluster)  [unwired: 1 in]
        n882 = call <vilib>:"Error Cluster From Error Code.vi"("show call chain? (False)"=TRUE, "error in (no error)"=w1988, "error message (\"\")"=w1989, "error code (0)"=w1990) -> ("error out"=w1987:errorcluster)  [unwired: 5 in]
        n883 = call <vilib>:"Add State(s) to Queue__jki_lib_state_machine.vi"("State(s) in (\"\")"=w1985) -> ("States Out"=w1984:string)  [unwired: 14 in]
      }
      frame "Error Handler" {
        # "Unhandled Error -- Display it"
        # "Handle any errors here.\nYou can also output any states to clean-up after errors occur"
        # "Clear error"
        n884 = call <vilib>:"General Error Handler.vi"("error in (no error)"=w1993) -> ()  [unwired: 10 in, 5 out]
        n885 = call <vilib>:"Add State(s) to Queue__jki_lib_state_machine.vi"("State(s) in Front (\"\")"="/* Post Error States", "State(s) in (\"\")"=w1997) -> ("States Out"=w1996:string)  [unwired: 13 in]
      }
      frame "Exit" {
        # "Do not put any code in this frame.\n(No errors that occur here will be handled.)"
        n886 = call <vilib>:"Add State(s) to Queue__jki_lib_state_machine.vi"("State(s) in (\"\")"=w2002) -> ("States Out"=w2001:string)  [unwired: 14 in]
      }
      frame "---------- Data ----------" {
        # "Do not put any code in this frame.\n(It is a separator no-op. You can make a copy of this frame to create a new Data frame)"
        n887 = call <vilib>:"Add State(s) to Queue__jki_lib_state_machine.vi"("State(s) in (\"\")"=w2006) -> ("States Out"=w2005:string)  [unwired: 14 in]
      }
      frame "Data: Initialize" {
        n888 = while {
          tunnel: [""] -> w2007
          stop <- w2013 stop-if-true
          n889 = Wait Until Next ms Multiple(millisecond multiple=u32 250) -> ()  [unwired: 1 out]
          n890 = call "UTILITY Boolean Notifier.vi"("Status"=UTILITY_Notifier."Read", "Set Status"=FALSE, "name (unnamed)"="Start UI Loop") -> ("latest READ notification"=w2013:bool)  [unwired: 7 in, 1 out]
        }
        n891 = Bundle(w2007) -> (w2009:cluster{string})  [unwired: 1 in]
        n892 = call <vilib>:"Add State(s) to Queue__jki_lib_state_machine.vi"("State(s) in (\"\")"=w2011) -> ("States Out"=w2010:string)  [unwired: 14 in]
      }
      frame "---------- Macro ----------" {
        # "Do not put any code in this frame.\n(It is a separator no-op. You can make a copy of this frame to create a new Macro frame)"
        n893 = call <vilib>:"Add State(s) to Queue__jki_lib_state_machine.vi"("State(s) in (\"\")"=w2021) -> ("States Out"=w2020:string)  [unwired: 14 in]
      }
      frame "Macro: Initialize" {
        # "Initialization Macro\n(This is called once, when the VI starts)"
        n894 = call <vilib>:"Add State(s) to Queue__jki_lib_state_machine.vi"("State(s) in Front (\"\")"="Data: Initialize", "State(s) in (\"\")"=w2026) -> ("States Out"=w2025:string)  [unwired: 13 in]
      }
      frame "------- Main Control Updater--------" {
        n895 = call <vilib>:"Add State(s) to Queue__jki_lib_state_machine.vi"("State(s) in (\"\")"=w2030) -> ("States Out"=w2029:string)  [unwired: 14 in]
      }
      frame "First Hour Check Status" {
        # "I have the cutout check in a seperate loop because the newfi can throw garbage sometimes and when\nthe elements switch it displays as a cutout. Secondly, since i check every 10 seconds...it slows my main\ncontrol loop, and therefore hinders PID performance on the intellifaucet"
        n896 = local read "Trigger With GEA2"() -> (w2034:bool)
        n897 = case shown="True" w2034 {
          tunnel: [w2039 w2058] -> w2032
          frame False {
            # "Event leads are more reliable"
            # "GEA2 can throw garbage...\ncheck to see if anything is still on."
            n898 = local read "POWER"() -> (w2051:T12)
            n899 = local read "Current"() -> (w2049:T19)
            n900 = Unbundle By Name(w2051) -> ("UE"=w2046:bool, "COMP"=w2047:bool, "LE"=w2043:bool)
            n901 = Unbundle By Name(w2051) -> ("COMP"=w2052:bool, "LE"=w2053:bool)
            n902 = Build Array(w2052, w2053) -> (w2054:bool[])
            n903 = Less?(x=w2049, y=0.5) -> (x < y?=w2045:bool)
            n904 = Build Array(w2046, w2047) -> (w2048:bool[])
            n905 = And Array Elements(Boolean array=w2054) -> (logical AND=w2055:bool)
            n906 = case shown="True" w2043 {
              tunnel: [w2056 TRUE] -> w2044
              tunnel: w2045 -> [w2056 _]
              frame False {
              }
              frame True {
              }
            }
            n907 = Or Array Elements(Boolean array=w2048) -> (logical OR=w2040:bool)
            n908 = Not(x=w2040) -> (.not. x?=w2042:bool)
            n909 = And(x=w2042, y=w2044) -> (x .and. y?=w2050:bool)
            n910 = Or(x=w2050, y=w2055) -> (x .or. y?=w2039:bool)
          }
          frame True {
            n911 = for {
              N: 3 -> [_]
              tunnel: [w2065] -> w2058
              # "We have the capability to turn the LE and COMP at\nthe same time...consider this condition a cutout"
              # "The standard says this"
              # "GEA2 can throw garbage...\ncheck to see if anything is still on."
              n912 = local read "POWER"() -> (w2064:T12)
              n913 = Wait Until Next ms Multiple(millisecond multiple=u32 1000) -> ()  [unwired: 1 out]
              n914 = local read "Current"() -> (w2068:T19)
              n915 = Unbundle By Name(w2064) -> ("UE"=w2071:bool, "COMP"=w2070:bool, "LE"=w2074:bool)
              n916 = Unbundle By Name(w2064) -> ("COMP"=w2063:bool, "LE"=w2062:bool)
              n917 = Build Array(w2063, w2062) -> (w2061:bool[])
              n918 = Less?(x=w2068, y=0.5) -> (x < y?=w2072:bool)
              n919 = Build Array(w2071, w2070) -> (w2069:bool[])
              n920 = And Array Elements(Boolean array=w2061) -> (logical AND=w2060:bool)
              n921 = case shown="False" w2074 {
                tunnel: [w2078 TRUE] -> w2073
                tunnel: w2072 -> [w2078 _]
                frame False {
                }
                frame True {
                }
              }
              n922 = Or Array Elements(Boolean array=w2069) -> (logical OR=w2077:bool)
              n923 = Not(x=w2077) -> (.not. x?=w2075:bool)
              n924 = And(x=w2075, y=w2073) -> (x .and. y?=w2066:bool)
              n925 = Or(x=w2066, y=w2060) -> (x .or. y?=w2065:bool)
            }
          }
        }
        n926 = call "UTILITY Boolean Notifier.vi"("Status"=UTILITY_Notifier."Set", "Set Status"=w2032, "name (unnamed)"="First Hour Cutout") -> ()  [unwired: 7 in, 2 out]
        n927 = call <vilib>:"Add State(s) to Queue__jki_lib_state_machine.vi"("State(s) in (\"\")"=w2038) -> ("States Out"=w2037:string)  [unwired: 14 in]
      }
      frame "Full Cutout" {
        # "I have the cutout check in a seperate loop because the newfi can throw garbage sometimes and when\nthe elements switch it displays as a cutout. Secondly, since i check every 10 seconds...it slows my main\ncontrol loop, and therefore hinders PID performance on the intellifaucet"
        n928 = local read "Trigger With GEA2"() -> (w2084:bool)
        n929 = case shown="True" w2084 {
          tunnel: [w2090 w2107] -> w2080
          tunnel: 3 -> [w2089 w2099]
          frame False {
            # "Ignore fan. It is not a heat\nsource"
            n930 = for {
              N: w2089 -> [_]
              tunnel: [w2097] -> w2093
              n931 = local read "POWER"() -> (w2098:T12)
              n932 = Wait Until Next ms Multiple(millisecond multiple=u32 1000) -> ()  [unwired: 1 out]
              n933 = call "HEWH Full Cutout Check.vi"("POWER"=w2098) -> ("Heat Source ON (1=ON)"=w2097:bool)  [unwired: 8 in, 2 out]
            }
            n934 = local read "Current"() -> (w2094:T19)
            n935 = Not(x=w2093) -> (.not. x?=w2092:bool)
            n936 = Less?(x=w2094, y=0.5) -> (x < y?=w2091:bool)
            n937 = Compound Arithmetic op=AND(w2092, w2091) -> (w2090:bool)
          }
          frame True {
            # "Ignore fan. It is not a heat\nsource"
            # "Helps prevent false triggers...comp should not turn off until >1 deg from T2"
            # "GEA2 can throw garbage...\ncheck to see if anything is still on."
            n938 = local read "Water Heater GEA2 Data"() -> (w2106:T36)
            n939 = for {
              N: w2099 -> [_]
              tunnel: [w2114] -> w2110
              n940 = local read "POWER"() -> (w2115:T12)
              n941 = Wait Until Next ms Multiple(millisecond multiple=u32 1000) -> ()  [unwired: 1 out]
              n942 = call "HEWH Full Cutout Check.vi"("POWER"=w2115) -> ("Heat Source ON (1=ON)"=w2114:bool)  [unwired: 8 in, 2 out]
            }
            n943 = Unbundle By Name(w2106) -> ("Hyperterminal Data.Setpoint Deg F"=w2105:i32, "Hyperterminal Data.T2(TankSensor)"=w2101:dbl)
            n944 = local read "Current"() -> (w2111:T19)
            n945 = Round Toward +Infinity(x=w2101) -> (ceil(x): smallest int >= x=w2100:dbl)
            n946 = Subtract(x=w2105, y=w2100) -> (x-y=w2104:dbl)
            n947 = Less Or Equal?(x=w2104, y=1.0) -> (x <= y?=w2102:bool)
            n948 = Not(x=w2110) -> (.not. x?=w2109:bool)
            n949 = Less?(x=w2111, y=0.5) -> (x < y?=w2108:bool)
            n950 = Compound Arithmetic op=AND(w2109, w2108, w2102) -> (w2107:bool)
          }
        }
        "Full Cutout" <- w2080
        n951 = call "UTILITY Boolean Notifier.vi"("Status"=UTILITY_Notifier."Set", "Set Status"=w2080, "name (unnamed)"="Full Cutout") -> ()  [unwired: 7 in, 2 out]
        n952 = call <vilib>:"Add State(s) to Queue__jki_lib_state_machine.vi"("State(s) in (\"\")"=w2088) -> ("States Out"=w2087:string)  [unwired: 14 in]
      }
      frame "Check for Exit" {
        n953 = local read "Shutdown Sequence"() -> (w2116:string)
        n954 = call <vilib>:"Add State(s) to Queue__jki_lib_state_machine.vi"("State(s) in Front (\"\")"=w2116, "State(s) in (\"\")"=w2120) -> ("States Out"=w2119:string)  [unwired: 13 in]
      }
    }
  }
  n955 = while "UI Events" {
    shift-right: [w2124] -> _
    shift-left: _ -> [w2123]
    shift-right: [w2127] -> _
    shift-left: _ -> [w2121]
    shift-right: [w2126] -> _
    shift-left: w59 -> [w2128]
    stop <- w2125 stop-if-true
    w2122 = 1000  # Timeout
    # "UI Events"
    n956 = call <vilib>:"Parse State Queue__jki_lib_state_machine.vi"("State Queue"=w2128, "Error In (no error)"=w2121) -> ("Remaining States"=w2130:string, "Current State"=w2131:string, "Arguments"=w2129:string)  [unwired: 11 in]
    n957 = case shown="\"\", \"Idle\"" w2131 {
      selector: w2131 -> [_ _ w2364 _ _ _ _ _ _ _ _ _ _ _ _ _ _ _ _]
      tunnel: w2130 -> [w2138 w2363 w2368 w2380 w2385 w2389 w2395 w2406 w2411 w2415 w2420 w2426 w2432 w2438 w2443 w2448 w2453 w2458 w2463]
      tunnel: w2129 -> [_ _ _ _ _ _ _ _ _ _ _ _ _ _ _ _ _ _ _]
      tunnel: w2123 -> [w2136 w2360 w2366 w2377 w2383 w2386 _ w2403 w2408 w2412 w2417 w2422 w2428 w2434 w2439 w2444 w2449 w2455 w2460]
      tunnel: [w2135 w2361 w2370 errorcluster {"status"=FALSE, "code"=0, "source"=""} ("error out") w2382 w2387 w2392 w2404 w2409 w2413 w2418 w2424 w2430 w2436 w2441 w2446 w2451 w2456 w2461] -> w2127
      tunnel: w2121 -> [w2134 w2361 w2369 w2376 w2382 w2387 w2392 w2404 w2409 w2413 w2418 w2424 w2430 w2436 w2441 w2446 w2451 w2456 w2461]
      tunnel: [w2137 w2362 w2367 w2379 w2384 w2388 w2394 w2405 w2410 w2414 w2419 w2425 w2431 w2437 w2442 w2447 w2452 w2457 w2462] -> w2126
      tunnel: [_ _ _ _ TRUE _ _ _ _ _ _ _ _ _ _ _ _ _ _] -> w2125
      tunnel: [w2133 w2360 w2366 w2377 w2383 w2386 w2393 w2403 w2408 w2412 w2417 w2422 w2428 w2434 w2439 w2444 w2449 w2455 w2460] -> w2124
      tunnel: w2122 -> [w2132 _ _ _ _ _ _ _ _ _ _ _ _ _ _ _ _ _ _]
      frame "", "Idle" {
        n958 = event shown="[18] \"Start 24 Hour Rating\": Value Change" {
          selector: _ -> [_ _ _ _ _ _ _ _ _ _ _ _ _ _ _ _ _ _ _ _ _ _ _ _]
          dyn-events: _ -> [_ _ _ _ _ _ _ _ _ _ _ _ _ _ _ _ _ _ _ _ _ _ _ _]
          timeout: w2132 -> [_ _ _ _ _ _ _ _ _ _ _ _ _ _ _ _ _ _ _ _ _ _ _ _]
          tunnel: w2138 -> [w2143 w2146 w2165 w2174 w2180 w2185 w2196 w2207 w2218 w2229 w2239 w2247 w2254 w2261 w2270 w2281 w2286 w2291 w2297 w2311 w2319 w2324 w2334 w2358]
          tunnel: [w2142 w2144 w2165 w2173 w2180 w2184 w2195 w2206 w2217 w2228 w2238 w2246 w2253 w2260 w2270 w2281 w2285 w2290 w2296 w2310 w2319 w2324 w2333 w2358] -> w2137
          tunnel: w2136 -> [w2140 w2148 w2166 w2175 w2181 w2188 w2200 w2211 w2222 w2233 w2241 w2244 w2251 w2258 w2271 w2282 w2287 w2293 w2299 w2312 w2320 w2325 w2335 w2359]
          tunnel: [w2141 w2147 w2164 w2171 w2179 w2192 w2201 w2214 w2225 w2234 w2240 w2248 w2255 w2262 w2264 w2276 w2288 w2292 w2298 w2307 w2321 w2326 w2331 w2353] -> w2135
          tunnel: w2134 -> [w2141 w2147 w2164 w2172 w2179 w2192 w2201 w2214 w2225 w2234 w2240 w2248 w2255 w2262 w2267 w2277 w2288 w2292 w2298 w2304 w2321 w2326 w2330 w2354]
          tunnel: [w2140 w2148 w2166 w2175 w2181 w2187 w2199 w2210 w2221 w2232 w2241 w2243 w2250 w2257 w2271 w2282 w2287 w2293 w2299 w2312 w2320 w2325 w2335 w2359] -> w2133
          event Timeout {
            n959 = event-data() -> ()  [unwired: 1 in, 1 out]
            n960 = call <vilib>:"Add State(s) to Queue__jki_lib_state_machine.vi"("State(s) in Front (\"\")"="Check for Exit" ("State(s) in Front (\"\")"), "State(s) in (\"\")"=w2143) -> ("States Out"=w2142:string)  [unwired: 13 in]
          }
          event Value Change {
            n961 = event-data() -> ()  [unwired: 1 in, 6 out]
            n962 = call <vilib>:"Add State(s) to Queue__jki_lib_state_machine.vi"("State(s) in Front (\"\")"="Start Shutdown\nExit" ("State(s) in Front (\"\")"), "State(s) in (\"\")"=w2146) -> ("States Out"=w2144:string)  [unwired: 13 in]
          }
          event "X-Axis", "Y-Axis": Value Change {
            n963 = event-data() -> ()  [unwired: 1 in, 6 out]
            n964 = local read "Plot File"() -> (w2163:path)
            n965 = call-poly <vilib>:"Read From Spreadsheet File.vi"("delimiter (\\t)"="," ("delimiter (\\t)"), "file path (dialog if empty)"=w2163) -> ("all rows"=w2158:string[][])  [unwired: 5 in, 4 out]
            n966 = Delete From Array(array=w2158, index (row)=0) -> (deleted portion=w2156:string[], array with subset deleted=w2155:string[][])  [unwired: 2 in]
            n967 = Search 1D Array(1D array=w2156, element="X-Axis") -> (index of element=w2160:i32)  [unwired: 1 in]
            n968 = Search 1D Array(1D array=w2156, element="Y-Axis") -> (index of element=w2159:i32)  [unwired: 1 in]
            n969 = Index Array(array=w2155, index (col)=w2160) -> (element=w2154:string[])  [unwired: 1 in]
            n970 = Index Array(array=w2155, index (col)=w2159) -> (element=w2153:string[])  [unwired: 1 in]
            n971 = for {
              tunnel: w2154 -> [w2170] mode=indexing
              tunnel: w2153 -> [w2169] mode=indexing
              tunnel: [w2168] -> w2151 mode=indexing
              tunnel: [w2167] -> w2152 mode=indexing
              n972 = Fract/Exp String To Number(string=w2170) -> (number=w2167:dbl)  [unwired: 3 in, 1 out]
              n973 = Fract/Exp String To Number(string=w2169) -> (number=w2168:dbl)  [unwired: 3 in, 1 out]
            }
            n974 = Bundle(w2152, w2151) -> (→"XY Graph":cluster{dbl[], dbl[]})  [unwired: 1 in]
          }
          event "Super Water Heater": Value Change {
            n975 = event-data() -> ()  [unwired: 1 in, 6 out]
            n976 = call "HEWH Panel Super Water Heater.vi"("error in (no error)"=w2172) -> ("error out"=w2171:errorcluster)  [unwired: 10 in]
            n977 = call <vilib>:"Add State(s) to Queue__jki_lib_state_machine.vi"("State(s) in (\"\")"=w2174) -> ("States Out"=w2173:string)  [unwired: 14 in]
          }
          event Value Change {
            w2176 = FALSE ("Visible")
            n978 = event-data() -> ()  [unwired: 1 in, 6 out]
            n979 = local write "Tab Control 3"(T32."Settings" ("Tab Control 3")) -> ()
            n980 = local write "Description"("Settings 2") -> ()
            n981 = property on="Average TC Tree Temperature" class="WFChart (strict)"("Visible"=w2176) -> ()  [unwired: 2 in, 2 out]
            n982 = property on="Flow Meter" class="WFChart (strict)"("Visible"=w2176) -> ()  [unwired: 2 in, 2 out]
            n983 = property on="Total Dispensed Gallons" class="WFChart (strict)"("Visible"=w2176) -> ()  [unwired: 2 in, 2 out]
          }
          event Value Change {
            w2182 = FALSE ("Visible")
            w2186 = FALSE
            n984 = event-data() -> ()  [unwired: 1 in, 6 out]
            n985 = property on="Flow Meter" class="WFChart (strict)"("Visible"=w2182) -> ()  [unwired: 2 in, 2 out]
            n986 = property on="Average TC Tree Temperature" class="WFChart (strict)"("Visible"=w2182) -> ()  [unwired: 2 in, 2 out]
            n987 = property on="Total Dispensed Gallons" class="WFChart (strict)"("Visible"=w2182) -> ()  [unwired: 2 in, 2 out]
            n988 = local read "Main 2"() -> (w2190:string)
            n989 = local write "Tab Control 3"(T32."Main" ("Tab Control 3")) -> ()
            n990 = local write "Message"(T23 "Select Test...." ("Message")) -> ()
            n991 = local write "Description"(w2190) -> ()
            n992 = Bundle By Name(cluster=w2188, "Program Names.Stand Override"=w2186, "Program Names.24 Hour Rating"=w2186, "Program Names.First Hour Rating"=w2186, "Program Names.Heat Up"=w2186, "Program Names.Channel Tester"=w2186) -> (w2187:T86)
            n993 = call <vilib>:"Add State(s) to Queue__jki_lib_state_machine.vi"("State(s) in Front (\"\")"="Update Program Status" ("State(s) in Front (\"\")"), "State(s) in (\"\")"=w2185) -> ("States Out"=w2184:string)  [unwired: 13 in]
          }
          event "Stand Override Panel": Value Change {
            w2193 = FALSE ("Visible")
            w2198 = FALSE
            n994 = event-data() -> ()  [unwired: 1 in, 6 out]
            n995 = local write "Description"("Stand Override") -> ()
            n996 = local write "Tab Control 3"(T32."Stand Override" ("Tab Control 3")) -> ()
            n997 = call <vilib>:"Add State(s) to Queue__jki_lib_state_machine.vi"("State(s) in Front (\"\")"="Update Program Status" ("State(s) in Front (\"\")"), "State(s) in (\"\")"=w2196) -> ("States Out"=w2195:string)  [unwired: 13 in]
            n998 = property on="Average TC Tree Temperature" class="WFChart (strict)"("Visible"=w2193) -> ()  [unwired: 2 in, 2 out]
            n999 = property on="Flow Meter" class="WFChart (strict)"("Visible"=w2193) -> ()  [unwired: 2 in, 2 out]
            n1000 = property on="Total Dispensed Gallons" class="WFChart (strict)"("Visible"=w2193) -> ()  [unwired: 2 in, 2 out]
            n1001 = Bundle By Name(cluster=w2200, "Program Names.Stand Override"=TRUE, "Program Names.24 Hour Rating"=w2198, "Program Names.First Hour Rating"=w2198, "Program Names.Heat Up"=w2198, "Program Names.Channel Tester"=w2198) -> (w2199:T86)
          }
          event "Heat Up Panel": Value Change {
            w2204 = TRUE ("Visible")
            w2208 = FALSE ("Program Names.Heat Up")
            n1002 = event-data() -> ()  [unwired: 1 in, 6 out]
            n1003 = property on="Average TC Tree Temperature" class="WFChart (strict)"("Visible"=w2204) -> ()  [unwired: 2 in, 2 out]
            n1004 = property on="Flow Meter" class="WFChart (strict)"("Visible"=w2204) -> ()  [unwired: 2 in, 2 out]
            n1005 = property on="Total Dispensed Gallons" class="WFChart (strict)"("Visible"=w2204) -> ()  [unwired: 2 in, 2 out]
            n1006 = local write "Tab Control 3"(T32."Heat Up" ("Tab Control 3")) -> ()
            n1007 = call <vilib>:"Add State(s) to Queue__jki_lib_state_machine.vi"("State(s) in Front (\"\")"="Update Program Status" ("State(s) in Front (\"\")"), "State(s) in (\"\")"=w2207) -> ("States Out"=w2206:string)  [unwired: 13 in]
            n1008 = local write "Description"("Heat Up") -> ()
            n1009 = Bundle By Name(cluster=w2211, "Program Names.Stand Override"=w2208, "Program Names.24 Hour Rating"=w2208, "Program Names.First Hour Rating"=w2208, "Program Names.Heat Up"=TRUE, "Program Names.Channel Tester"=w2208) -> (w2210:T86)
          }
          event "First Hour Rating Panel": Value Change {
            w2215 = TRUE ("Visible")
            w2219 = FALSE ("Program Names.First Hour Rating")
            n1010 = event-data() -> ()  [unwired: 1 in, 6 out]
            n1011 = property on="Flow Meter" class="WFChart (strict)"("Visible"=w2215) -> ()  [unwired: 2 in, 2 out]
            n1012 = property on="Average TC Tree Temperature" class="WFChart (strict)"("Visible"=w2215) -> ()  [unwired: 2 in, 2 out]
            n1013 = property on="Total Dispensed Gallons" class="WFChart (strict)"("Visible"=w2215) -> ()  [unwired: 2 in, 2 out]
            n1014 = local write "Tab Control 3"(T32."First Hour Rating" ("Tab Control 3")) -> ()
            n1015 = call <vilib>:"Add State(s) to Queue__jki_lib_state_machine.vi"("State(s) in Front (\"\")"="Update Program Status" ("State(s) in Front (\"\")"), "State(s) in (\"\")"=w2218) -> ("States Out"=w2217:string)  [unwired: 13 in]
            n1016 = local write "Description"("First Hour Rating") -> ()
            n1017 = Bundle By Name(cluster=w2222, "Program Names.Stand Override"=w2219, "Program Names.24 Hour Rating"=w2219, "Program Names.First Hour Rating"=TRUE, "Program Names.Heat Up"=w2219, "Program Names.Channel Tester"=w2219) -> (w2221:T86)
          }
          event "24 Hour Rating Panel": Value Change {
            w2226 = TRUE ("Visible")
            w2230 = FALSE ("Program Names.Stand Override")
            n1018 = event-data() -> ()  [unwired: 1 in, 6 out]
            n1019 = local write "Tab Control 3"(T32."24 Hour Rating" ("Tab Control 3")) -> ()
            n1020 = local write "Description"("24 Hour Rating") -> ()
            n1021 = call <vilib>:"Add State(s) to Queue__jki_lib_state_machine.vi"("State(s) in Front (\"\")"="Update Program Status" ("State(s) in Front (\"\")"), "State(s) in (\"\")"=w2229) -> ("States Out"=w2228:string)  [unwired: 13 in]
            n1022 = Bundle By Name(cluster=w2233, "Program Names.Stand Override"=w2230, "Program Names.24 Hour Rating"=TRUE, "Program Names.First Hour Rating"=w2230, "Program Names.Heat Up"=w2230, "Program Names.Channel Tester"=w2230) -> (w2232:T86)
            n1023 = property on="Flow Meter" class="WFChart (strict)"("Visible"=w2226) -> ()  [unwired: 2 in, 2 out]
            n1024 = property on="Average TC Tree Temperature" class="WFChart (strict)"("Visible"=w2226) -> ()  [unwired: 2 in, 2 out]
            n1025 = property on="Total Dispensed Gallons" class="WFChart (strict)"("Visible"=w2226) -> ()  [unwired: 2 in, 2 out]
          }
          event "Draw Schedule": Value Change {
            n1026 = event-data() -> ()  [unwired: 1 in, 6 out]
            n1027 = call <vilib>:"Add State(s) to Queue__jki_lib_state_machine.vi"("State(s) in Front (\"\")"="Draw Schedule" ("State(s) in Front (\"\")"), "State(s) in (\"\")"=w2239) -> ("States Out"=w2238:string)  [unwired: 13 in]
          }
          event "Inlet Valve A": Value Change {
            n1028 = event-data() -> ("NewVal"=w2242:enum8{"OPEN", "CLOSE"})  [unwired: 1 in, 5 out]
            n1029 = Bundle By Name(cluster=w2244, "User Controls DAQ LOOP.Valves.In VLV A"=w2242) -> (w2243:T86)
            n1030 = call <vilib>:"Add State(s) to Queue__jki_lib_state_machine.vi"("State(s) in Front (\"\")"="Inlet Valve" ("State(s) in Front (\"\")"), "State(s) in (\"\")"=w2247) -> ("States Out"=w2246:string)  [unwired: 13 in]
          }
          event "Drain Valve A": Value Change {
            n1031 = event-data() -> ("NewVal"=w2249:enum8{"OPEN", "CLOSE"})  [unwired: 1 in, 5 out]
            n1032 = Bundle By Name(cluster=w2251, "User Controls DAQ LOOP.Valves.Drain VLV A"=w2249) -> (w2250:T86)
            n1033 = call <vilib>:"Add State(s) to Queue__jki_lib_state_machine.vi"("State(s) in Front (\"\")"="Drain Valve" ("State(s) in Front (\"\")"), "State(s) in (\"\")"=w2254) -> ("States Out"=w2253:string)  [unwired: 13 in]
          }
          event "Outlet Valve A": Value Change {
            n1034 = event-data() -> ("NewVal"=w2256:enum8{"CLOSE", "OPEN"})  [unwired: 1 in, 5 out]
            n1035 = Bundle By Name(cluster=w2258, "User Controls DAQ LOOP.Valves.Out VLV A"=w2256) -> (w2257:T86)
            n1036 = call <vilib>:"Add State(s) to Queue__jki_lib_state_machine.vi"("State(s) in Front (\"\")"="Outlet Valve" ("State(s) in Front (\"\")"), "State(s) in (\"\")"=w2261) -> ("States Out"=w2260:string)  [unwired: 13 in]
          }
          event "Setpoint": Value Change {
            n1037 = event-data() -> ()  [unwired: 1 in, 6 out]
            n1038 = call "HEWH_DSM_CMD.vi"("Heating Mode"="Mode", "GEA2 Commands and Requests"=GEA2_Commands."CMD_UPDATE_MODE") -> ("Input Data"=w2266:T59)  [unwired: 7 in, 1 out]
            n1039 = call "HEWH_DSM_CMD.vi"("Temperature"="HEWH Setpoint", "GEA2 Commands and Requests"=GEA2_Commands."CMD_WRITE_SETPOINTS") -> ("Input Data"=w2263:T59)  [unwired: 7 in, 1 out]
            n1040 = call "Send Example.vi"("Input Data"=w2266, "Error In"=w2267) -> ("Error Out"=w2265:errorcluster)  [unwired: 13 in]
            n1041 = call "Send Example.vi"("Input Data"=w2263, "Error In"=w2265) -> ("Error Out"=w2264:errorcluster)  [unwired: 13 in]
          }
          event "Software Version": Value Change {
            w2275 = GEA2_Commands."RQST_Software_Version" ("GEA2 Commands and Requests")
            n1042 = event-data() -> ()  [unwired: 1 in, 6 out]
            n1043 = call "HEWH_DSM_CMD.vi"("GEA2 Commands and Requests"=w2275) -> ("Input Data"=w2278:T59)  [unwired: 8 in, 1 out]
            n1044 = call "Send and Receive Example.vi"("Input Data"=w2278, "Error In"=w2277) -> ("Coverted Data Out"=w2274:T62, "Error Out"=w2276:errorcluster)  [unwired: 11 in, 1 out]
            n1045 = call "GEA2 Message Decoder.vi"("GEA2 Commands and Requests"=w2275, "Coverted Data Out"=w2274) -> ("GEA Information Out"=w2280:T63)  [unwired: 9 in]
            n1046 = Unbundle By Name(w2280) -> ("Software String"=→"Sofware Version":string)
          }
          event "Start Multi-Draw": Value Change {
            n1047 = event-data() -> ()  [unwired: 1 in, 6 out]
            n1048 = call <vilib>:"Add State(s) to Queue__jki_lib_state_machine.vi"("State(s) in Front (\"\")"="Start Multi Draw" ("State(s) in Front (\"\")"), "State(s) in (\"\")"=w2286) -> ("States Out"=w2285:string)  [unwired: 13 in]
            "Multi-Draw" <- TRUE ("Mult-Draw")
          }
          event "Draw Until?": Value Change {
            n1049 = event-data() -> ()  [unwired: 1 in, 6 out]
            n1050 = call <vilib>:"Add State(s) to Queue__jki_lib_state_machine.vi"("State(s) in Front (\"\")"="Draw Until" ("State(s) in Front (\"\")"), "State(s) in (\"\")"=w2291) -> ("States Out"=w2290:string)  [unwired: 13 in]
          }
          event "Start 24 Hour Rating": Value Change {
            n1051 = event-data() -> ()  [unwired: 1 in, 6 out]
            n1052 = local write "Shutdown"("Dispense Schedule\nFile Setup\nPreDraw\nStart DAQ Write\nReset Totalizer\nWait for Heat Cutout" ("State(s) in Front (\"\")")) -> ()
            n1053 = property on="Start 24 Hour Rating" class="Bool"("Visible"=FALSE) -> ()  [unwired: 2 in, 2 out]
            n1054 = call <vilib>:"Add State(s) to Queue__jki_lib_state_machine.vi"("State(s) in (\"\")"=w2297) -> ("States Out"=w2296:string)  [unwired: 14 in]
          }
          event "Start First Hour Rating": Value Change {
            # "Update mode to hybrid"
            n1055 = event-data() -> ()  [unwired: 1 in, 6 out]
            n1056 = call "HEWH_DSM_CMD.vi"("Heating Mode"=GEA2_Commands_HEWH_Mode."Hybrid" ("Mode"), "GEA2 Commands and Requests"=GEA2_Commands."CMD_UPDATE_MODE") -> ("Input Data"=w2301:T59)  [unwired: 7 in, 1 out]
            n1057 = property on="Start First Hour Rating" class="Bool"("Visible"=FALSE) -> ()  [unwired: 2 in, 2 out]
            n1058 = call "Send Example.vi"("Input Data"=w2301, "Retry Count"=u32 3, "Error In"=w2304) -> ("Error Out"=w2303:errorcluster)  [unwired: 12 in]
            n1059 = call "HEWH Temperature Decrease FHD.vi"("error in (no error)"=w2303) -> ("error out"=w2306:errorcluster, "Temperature Decrease Output"=w2305:T19)  [unwired: 8 in]
            n1060 = flat-sequence {
              tunnel: w2306 -> [w2317]
              tunnel: [w2317] -> w2307
              tunnel: w2305 -> [w2313]
              frame #0 {
                n1061 = local write "Decrease Outlet\nTemperature By (RTD Out)"(w2313) -> ()
                n1062 = local write "GPM Target"("First Hour GPM Target") -> ()
                n1063 = local write "Temperature"("First Hour Temperature") -> ()
                n1064 = local write "Shutdown"("File Setup\nPreDraw\nStart DAQ Write\nReset Totalizer\nFirst Hour Cutout" ("State(s) in Front (\"\")")) -> ()
              }
            }
            n1065 = call <vilib>:"Add State(s) to Queue__jki_lib_state_machine.vi"("State(s) in (\"\")"=w2311) -> ("States Out"=w2310:string)  [unwired: 14 in]
          }
          event "IF Start": Value Change {
            n1066 = event-data() -> ("NewVal"=w2318:bool)  [unwired: 1 in, 5 out]
            n1067 = case shown="False" w2318 {
              frame False {
              }
              frame True {
                n1068 = local write "Shutdown"("Start Intellifaucet" ("State(s) in Front (\"\")")) -> ()
              }
            }
          }
          event "IF Stop": Value Change {
            n1069 = event-data() -> ("NewVal"=w2323:bool)  [unwired: 1 in, 5 out]
            n1070 = case shown="True" w2323 {
              frame False {
              }
              frame True {
                n1071 = local write "Shutdown"("Stop Intellifaucet" ("State(s) in Front (\"\")")) -> ()
              }
            }
          }
          event "Write To File": Value Change {
            # "When you start data collection it will send you to the\nFileInit setup. When you turn off, it will stop the DAQ \nloop. Each time you turn on data collection it will \nsend you to the FileInit screen...thereby creating a \nnew file. If you use the same TR and Lab ID number\nit will save in the same folder"
            n1072 = event-data() -> ()  [unwired: 1 in, 6 out]
            n1073 = local read "Start DAQ Write"() -> (w2332:bool)
            n1074 = case shown="True" w2332 {
              tunnel: w2330 -> [w2340 w2351]
              tunnel: [w2338 w2351] -> w2331
              tunnel: ["" "Exit"] -> w2328
              frame False {
                n1075 = flat-sequence {
                  tunnel: w2340 -> [w2343]
                  tunnel: [w2342] -> w2339
                  tunnel: [w2341] -> w2337
                  tunnel: w2339 -> [w2347]
                  tunnel: [w2347] -> w2338
                  tunnel: w2337 -> [w2346]
                  frame #0 {
                    n1076 = call "HEWH Panel Collect Data for Specific Time.vi"("error in (no error)"=w2343) -> ("error out"=w2342:errorcluster, "Back Button"=w2341:bool, "Elapsed Time Output"=→"Elapsed Time Output":T20, "Continuous Data Collection Output"=→"Continuous Data Collection Output":bool)  [unwired: 7 in]
                  }
                  frame #1 {
                    n1077 = case shown="False" w2346 {
                      frame False {
                        n1078 = local write "Shutdown"("File Setup\nStart DAQ Write" ("Shutdown")) -> ()
                      }
                      frame True {
                      }
                    }
                  }
                }
              }
              frame True {
                # "Turn off the data collection without\ngoing back to the FileInit state"
                n1079 = local write "Start DAQ Write"(FALSE ("Start DAQ Write")) -> ()
                n1080 = local write "Shutdown"("Add Headers" ("Shutdown")) -> ()
              }
            }
            n1081 = call <vilib>:"Add State(s) to Queue__jki_lib_state_machine.vi"("State(s) in Front (\"\")"=w2328, "State(s) in (\"\")"=w2334) -> ("States Out"=w2333:string)  [unwired: 13 in]
            "Write To File Change" <- TRUE ("Write To File Change")
          }
          event "Stop Custom Draw": Value Change {
            n1082 = event-data() -> ()  [unwired: 1 in, 6 out]
            n1083 = call "UTILITY Boolean Notifier.vi"("Status"=UTILITY_Notifier."Set", "error in (no error)"=w2354, "Set Status"=TRUE, "name (unnamed)"="Stop Custom Draw") -> ("error out"=w2353:errorcluster)  [unwired: 6 in, 1 out]
          }
        }
      }
      frame "---------- Core ----------" {
        # "Do not put any code in this frame.\n(it is a separator no-op)"
        n1084 = call <vilib>:"Add State(s) to Queue__jki_lib_state_machine.vi"("State(s) in (\"\")"=w2363) -> ("States Out"=w2362:string)  [unwired: 14 in]
      }
      frame Default {
        w2373 = 42 items=["No error", "Argument error", "Memory is full", "Out of zone", "End of file", "File already open", "Generic file I/O error", "File not found", "File permission error", "Disk is full", "Duplicate path", "Too many files open", "System feature not enabled", "Resource file not found", "Cannot add resource", "Resource not found", "Image not found", "Image memory error", "Pen does not exist", "Config type invalid", "Config token not found", "Config parse error", "Config memory error", "Bad external code format", "Bad external code offset", "External code not present", "Null window", "Destroy window error", "Null menu", "Print aborted", "Bad print record", "Print driver error", "Windows error during printing", "Memory error during printing", "Print dialog error", "Generic print error", "Invalid device refnum", "Device not found", "Device parameter error", "Device unit error", "Cannot open device", "Device call aborted", "Generic error", "Cancelled by user", "Object ID too low", "Object ID too high", "Object not in heap", "Unknown heap", "Unknown object (invalid DefProc)", "Unknown object (DefProc not in table)", "Message out of range", "Invalid (null) method", "Unknown message", "Manager call not supported", "Bad address", "Network operation in progress", "Network operation timed out", "Connection is busy", "Network attribute not supported", "Network error", "Address in use", "System out of memory", "Connection aborted", "Connection refused", "Not connected", "Already connected", "Connection closed", "Initialization error (interapplication manager)", "Bad occurrence", "Wait on unbound occurrence handler", "Occurrence queue overflow", "Datalog type conflict", "Unused", "Unrecognized type (interapplication manager)", "Memory corrupt", "Failed to make temporary DLL", "Old CIN version", "Drag socket not found", "Failed to load drop-object", "Failed to register OLE object", "Failed to release OLE object", "Format specifier type mismatch", "Unknown format specifier", "Too few format specifiers", "Too many format specifiers", "Scan failed", "Newer CIN version", "Error converting to variant", "Runtime menu error", "Password tampered", "Variant attribute not found", "Incompatible variant data type", "Event data is not available", "Event Store is not present", "Occurrence is not found", "Event Queue is not created", "Event info is not available", "Refnum passed is NULL", "Error retrieving Class GUID", "Error retrieving CoClass GUID", "Error retrieving TypeLib GUID.", "Bad built application magic bytes.", "Specific driver is different from the specific driver associated with the Logical Name.", "There is no session opened to the class driver.", "Max Error", "MAX - Error with config objects", "MAX - Error loading configuration", "MAX - Group not supported"]
        # "Current State"
        # "Do not delete, rename, or modify this frame.\n(this is used to capture unhandled states and typos)"
        # "Handle mistyped state name (developer tool)"
        n1085 = Format Into String(format string="Software Exception: Unhandled State \"%s\"." ("message"), error in=w2369, w2364) -> (resulting string=w2372:string, error out=w2371:errorcluster)  [unwired: 1 in]
        n1086 = call <vilib>:"Error Cluster From Error Code.vi"("show call chain? (False)"=TRUE, "error in (no error)"=w2371, "error message (\"\")"=w2372, "error code (0)"=w2373) -> ("error out"=w2370:errorcluster)  [unwired: 5 in]
        n1087 = call <vilib>:"Add State(s) to Queue__jki_lib_state_machine.vi"("State(s) in (\"\")"=w2368) -> ("States Out"=w2367:string)  [unwired: 14 in]
      }
      frame "Error Handler" {
        # "Unhandled Error -- Display it"
        # "Handle any errors here.\nYou can also output any states to clean-up after errors occur"
        # "Clear error"
        n1088 = call <vilib>:"General Error Handler.vi"("error in (no error)"=w2376) -> ()  [unwired: 10 in, 5 out]
        n1089 = call <vilib>:"Add State(s) to Queue__jki_lib_state_machine.vi"("State(s) in Front (\"\")"="/* Post Error States", "State(s) in (\"\")"=w2380) -> ("States Out"=w2379:string)  [unwired: 13 in]
      }
      frame "Exit" {
        # "Do not put any code in this frame.\n(No errors that occur here will be handled.)"
        n1090 = call <vilib>:"Add State(s) to Queue__jki_lib_state_machine.vi"("State(s) in (\"\")"=w2385) -> ("States Out"=w2384:string)  [unwired: 14 in]
      }
      frame "---------- Data ----------" {
        # "Do not put any code in this frame.\n(It is a separator no-op. You can make a copy of this frame to create a new Data frame)"
        n1091 = call <vilib>:"Add State(s) to Queue__jki_lib_state_machine.vi"("State(s) in (\"\")"=w2389) -> ("States Out"=w2388:string)  [unwired: 14 in]
      }
      frame "Data: Initialize" {
        n1092 = while {
          tunnel: [w2401] -> w2391
          tunnel: [w2400] -> w2390
          stop <- w2397 stop-if-true
          n1093 = local read "Program Names"() -> (w2400:T25)
          n1094 = call "UTILITY Boolean Notifier.vi"("Status"=UTILITY_Notifier."Read", "Set Status"=FALSE, "name (unnamed)"="Start UI Loop") -> ("latest READ notification"=w2397:bool)  [unwired: 7 in, 1 out]
          n1095 = local read "User Controls DAQ LOOP"() -> (w2401:T28)
          n1096 = Wait Until Next ms Multiple(millisecond multiple=u32 250) -> ()  [unwired: 1 out]
        }
        n1097 = Bundle("User Controls DAQ LOOP"=w2391, "Program Names"=w2390) -> (w2393:T86)  [unwired: 1 in]
        n1098 = call <vilib>:"Add State(s) to Queue__jki_lib_state_machine.vi"("State(s) in (\"\")"=w2395) -> ("States Out"=w2394:string)  [unwired: 14 in]
      }
      frame "---------- Macro ----------" {
        # "Do not put any code in this frame.\n(It is a separator no-op. You can make a copy of this frame to create a new Macro frame)"
        n1099 = call <vilib>:"Add State(s) to Queue__jki_lib_state_machine.vi"("State(s) in (\"\")"=w2406) -> ("States Out"=w2405:string)  [unwired: 14 in]
      }
      frame "Macro: Initialize" {
        # "Initialization Macro\n(This is called once, when the VI starts)"
        n1100 = call <vilib>:"Add State(s) to Queue__jki_lib_state_machine.vi"("State(s) in Front (\"\")"="Data: Initialize", "State(s) in (\"\")"=w2411) -> ("States Out"=w2410:string)  [unwired: 13 in]
      }
      frame "------- Main Control Updater--------" {
        n1101 = call <vilib>:"Add State(s) to Queue__jki_lib_state_machine.vi"("State(s) in (\"\")"=w2415) -> ("States Out"=w2414:string)  [unwired: 14 in]
      }
      frame "Start Shutdown" {
        n1102 = call <vilib>:"Add State(s) to Queue__jki_lib_state_machine.vi"("State(s) in (\"\")"=w2420) -> ("States Out"=w2419:string)  [unwired: 14 in]
        "Shutdown" <- "Term Purge\nTerm Draw\nAdd Headers\nMacro: Exit"
      }
      frame "Inlet Valve" {
        n1103 = Unbundle By Name(w2422) -> ("User Controls DAQ LOOP.Valves.In VLV A"=→"In Valve UI":T29)
        n1104 = local write "Shutdown"("In Valve 1" ("State(s) in Front (\"\")")) -> ()
        n1105 = call <vilib>:"Add State(s) to Queue__jki_lib_state_machine.vi"("State(s) in (\"\")"=w2426) -> ("States Out"=w2425:string)  [unwired: 14 in]
      }
      frame "Drain Valve" {
        n1106 = Unbundle By Name(w2428) -> ("User Controls DAQ LOOP.Valves.Drain VLV A"=→"Drain VLV UI":T29)
        n1107 = local write "Shutdown"("Drain Valve 1" ("State(s) in Front (\"\")")) -> ()
        n1108 = call <vilib>:"Add State(s) to Queue__jki_lib_state_machine.vi"("State(s) in (\"\")"=w2432) -> ("States Out"=w2431:string)  [unwired: 14 in]
      }
      frame "Outlet Valve" {
        n1109 = Unbundle By Name(w2434) -> ("User Controls DAQ LOOP.Valves.Out VLV A"=→"Out VLV UI":T29)
        n1110 = local write "Shutdown"("Outlet Valve 1" ("State(s) in Front (\"\")")) -> ()
        n1111 = call <vilib>:"Add State(s) to Queue__jki_lib_state_machine.vi"("State(s) in (\"\")"=w2438) -> ("States Out"=w2437:string)  [unwired: 14 in]
      }
      frame "Draw Schedule" {
        # "Communicate with the control loop"
        n1112 = local write "Shutdown"("Dispense Schedule" ("State(s) in Front (\"\")")) -> ()
        n1113 = call <vilib>:"Add State(s) to Queue__jki_lib_state_machine.vi"("State(s) in (\"\")"=w2443) -> ("States Out"=w2442:string)  [unwired: 14 in]
      }
      frame "Start Multi Draw" {
        # "Communicate with the control loop"
        n1114 = local write "Shutdown"("Start Multi Draw" ("State(s) in Front (\"\")")) -> ()
        n1115 = call <vilib>:"Add State(s) to Queue__jki_lib_state_machine.vi"("State(s) in (\"\")"=w2448) -> ("States Out"=w2447:string)  [unwired: 14 in]
      }
      frame "Draw Until" {
        # "Communicate with the control loop"
        n1116 = local write "Shutdown"("Draw Until" ("State(s) in Front (\"\")")) -> ()
        n1117 = call <vilib>:"Add State(s) to Queue__jki_lib_state_machine.vi"("State(s) in (\"\")"=w2453) -> ("States Out"=w2452:string)  [unwired: 14 in]
      }
      frame "Update Program Status" {
        # "When you select a program from the main screen...update the main control loop\nso it knows the sequence to run"
        n1118 = Unbundle By Name(w2455) -> ("Program Names"=→"Program Names Update":T25)
        n1119 = call <vilib>:"Add State(s) to Queue__jki_lib_state_machine.vi"("State(s) in (\"\")"=w2458) -> ("States Out"=w2457:string)  [unwired: 14 in]
      }
      frame "Check for Exit" {
        # "Check for EXIT"
        n1120 = call <vilib>:"Add State(s) to Queue__jki_lib_state_machine.vi"("State(s) in Front (\"\")"="Shutdown Sequence", "State(s) in (\"\")"=w2463) -> ("States Out"=w2462:string)  [unwired: 13 in]
      }
    }
  }
  n1121 = while {
    tunnel: w2 -> [w2469]
    tunnel: [w2467] -> _
    stop <- w2465 stop-if-true
    # "Validate this routine"
    n1122 = Wait Until Next ms Multiple(millisecond multiple=u32 100) -> ()  [unwired: 1 out]
    n1123 = local read "Program Names Update"() -> (w2474:T25)
    n1124 = call "UTILITY String Notifier.vi"("Status"=UTILITY_Notifier."Set", "error in (no error)"=w2469, "Set Status"=T23 "Waiting for Max Stabilized Temp...." ("Message"), "name (unnamed)"="Message") -> ("error out"=w2468:errorcluster)  [unwired: 6 in, 1 out]
    n1125 = call "HEWH Wait For Temp Decline.vi"("Program Names"=w2474, "Error In"=w2468, "Last Draw TC Tree AVG Decline Amount (Degrees F)"="Last Draw TC Tree AVG Decline Amount (Degrees F)") -> ("Core HEWH Data Output"=w2466:T83, "Error Out"=w2467:errorcluster)  [unwired: 14 in, 1 out]
    n1126 = Unbundle By Name(w2466) -> ("Start Dispense Pattern"=w2465:bool)
  }
  n1127 = local read "Message"() -> ()  [unwired: 1 in]
  n1128 = while {
    stop <- _ stop-if-true
    n1129 = local read "Remaining Draws"() -> ()  [unwired: 1 in]
    n1130 = flat-sequence {
      frame #0 {
        "Start Draw Routine" <- TRUE ("Dispensing")
        "Start Draw Timer" <- TRUE ("Start Draw Timer")
      }
      frame #1 {
        n1131 = case shown="True" "Dispense" {
          frame False {
          }
          frame True {
            n1132 = local read "POWER"() -> ()  [unwired: 1 out]
            n1133 = call "HEWH Purge Draw Sequence.vi"("Purge Time (Seconds)"="Purge Time (Seconds)", "Station Draw Info"="Temperature", "Current Cond"="GPM Target", 4:"Gallon Target", "Skip Purge"="Skip Purge", "Skip Draw"="Skip Draw") -> ("Use Fuzzy Logic"=w2479:bool)  [unwired: 11 in, 2 out]
            n1134 = Unbundle By Name(w2479) -> ("In VLV A"=w2484, "Drain VLV A"=w2483, "Out VLV A"=w2482)
            n1135 = property on="Drain Valve A" class="Enum (strict)"("Value"=w2483) -> ()  [unwired: 2 in, 2 out]
            n1136 = property on="Inlet Valve A" class="Enum (strict)"("Value"=w2484) -> ()  [unwired: 2 in, 2 out]
            n1137 = property on="Outlet Valve A" class="Enum (strict)"("Value"=w2482) -> ()  [unwired: 2 in, 2 out]
          }
        }
      }
      frame #2 {
        n1138 = local write "Start Draw Routine"(FALSE ("Dispensing")) -> ()
      }
    }
    n1139 = local write "Message"(T23 "Terminating Purge and Setting Valves...." ("Message")) -> ()
  }
  n1140 = Unbundle By Name(w48) -> ("Equipment VISA.WT210"=w46:refnum<visa-resource-name>, "Core HEWH Data DAQ LOOP.HEWH Specific DAQ.Power Analyzer"=w47:T14)
  n1141 = call "GEA2 Stop.vi"("GEA2 Reference Out"=w50, "Error In"=w45) -> ()  [unwired: 13 in, 1 out]
  n1142 = case shown="True" w34 {
    tunnel: w36 -> [w2491 _]
    tunnel: w35 -> [w2490 _]
    frame False {
      n1143 = Close File(refnum=w2490, error in=w2491) -> ()  [unwired: 2 out]
    }
    frame True {
    }
  }
  n1144 = case shown="\"WT300\"" w47 {
    tunnel: w46 -> [_ w2492 w2495]
    tunnel: w45 -> [_ w2493 w2494]
    frame "OSI", Default {
    }
    frame "WT210" {
      n1145 = call "Close.vi"("VISA resource name"=w2492, "error in (no error)"=w2493) -> ()  [unwired: 13 in, 1 out]
    }
    frame "WT300" {
      n1146 = call "Close.vi"("error in (no error)"=w2494, "VISA resource name"=w2495) -> ()  [unwired: 9 in, 1 out]
    }
  }
  n1147 = disable-structure shown="Disabled" {
    frame Disabled {
      n1148 = local read "Flow Rate (GPM)"() -> ()  [unwired: 1 out]
      n1149 = local write "Shutdown"("Set Temp\nAdjust Temp\nDispense Gallons" ("State(s) in Front (\"\")")) -> ()
    }
    frame Enabled {
    }
  }
  n1150 = stacked-sequence {
    frame #0 {
    }
    frame #1 {
    }
  }
